vi "Cascade front panel-blockissues.vi"() -> ()   [LabVIEW 2016]
uses:
  sdi_12/SDI-12/Sonde Vertical Graph.ctl
  controls/Vertical Chart.ctl
  sdi_12/Groundwater header.ctl
  controls/MCC DAQ Setup.ctl
  controls/Aux Sensor.ctl
  KPRO_2016 subvis/Control 2.ctl
  KPRO_2016 subvis/Graph Controls 2.ctl
  KPRO_2016 subvis/Ik control.ctl
  controls/MCC DAQ Readings.ctl
  controls/Kpro pressure measurement cluster.ctl
  controls/Kpro hydraulic measurement cluster.ctl
  activeXtest/activeXtest 2015 Folder/sonde cluster from excel.ctl
  sdi_12/Sonde Value Percent Tol.ctl
  activeXtest/activeXtest 2015 Folder/sample data row cluster.ctl
  activeXtest/activeXtest 2015 Folder/sonde cluster.ctl
  KPRO_2016 subvis/Sensor Physical Measurements.ctl
  KPRO_2016 subvis/SS Control 7.ctl
  <vilib>/Utility/NIReport.llb/NI_report.lvclass
  controls/Action Control 1.ctl
  <extravilib>/ChannelInstances/One Element Stream-t'Action Control 1.ctl'/Instantiate.vi
  <extravilib>/ChannelInstances/One Element Stream-t'Action Control 1.ctl'/Endpoint.vi
  KPRO_2016 subvis/Kpro Globals.vi
  <vilib>/Utility/file.llb/Write Delimited Spreadsheet (string).vi
  <userlib>/_OpenG.lib/file/file.llb/Strip Path - Traditional__ogtk.vi
  <userlib>/_OpenG.lib/file/file.llb/Build Path - Traditional__ogtk.vi
  <vilib>/Utility/file.llb/Write Delimited Spreadsheet (DBL).vi
  <vilib>/ULx/Create Channel.llb/ULx Create Channel (AI-Voltage-Basic).vi
  <userlib>/_OpenG.lib/file/file.llb/Strip Path Extension - Path__ogtk.vi
  KPRO_2016 subvis/Global_SIM_switch.vi
  C:/Program Files (x86)/National Instruments/LabVIEW 2016/vi.lib/ULx/ULx_LV.dll
  Program Files (x86)/National Instruments/LabVIEW 2016/vi.lib/ULx/ULx_LV.dll
  <vilib>/Utility/config.llb/NI_LVConfig.lvlib
  <extravilib>/ChannelInstances/One Element Stream-t'Action Control 1.ctl'.lvlib
panel:
  out "Sonde OK":bool
  out "DAQ On":bool
  out "Number of Sample Sheets":i32
  out "Columns":i32[](array[numeric])
  in  "Create Excel File":bool
  out "output cluster":T1 caption="Cluster" {"Salinity" format="%_3g"; "Temp\ndeg C" format="%_2g"; "ORP" format="%_4g"; "pH" format="%_4g"; "Dissolved\nOxygen mg/L" format="%_3g"; "Specific\nCond (mS)" format="%_4g"; "Cumulative\nVolume (ml)" format="%#_4g"}
  out "Serial Number/MISC":string
  in  "Depth mode":bool caption="Use \nIncrement"
  in  "Sample Sheet Data Row Cluster 2":T2={"Head\nPressure"=0.0, "Depth"=0.0, "comment string"="", "Sonde Data Cluster"={"Cumulative\nVolume (ml)"=100.0, "Specific\nCond (mS)"=2.0, "Dissolved\nOxygen mg/L"=3.0, "pH"=4.0, "ORP"=5.0, "Temp\ndeg C"=26.0, "Salinity"=7.0}, "Aux1"=0.0, "Aux2"=0.0, "Aux3"=0.0} {"Sonde Data Cluster"."Salinity" format="%_3g"; "Sonde Data Cluster"."Temp\ndeg C" format="%_2g"; "Sonde Data Cluster"."ORP" format="%_4g"; "Sonde Data Cluster"."pH" format="%_4g"; "Sonde Data Cluster"."Dissolved\nOxygen mg/L" format="%_4g"; "Sonde Data Cluster"."Specific\nCond (mS)" format="%_4g"; "Sonde Data Cluster"."Cumulative\nVolume (ml)" format="%#_4g"; "Depth" format="%#.3g"; "Head\nPressure" format="%#.4g"}
  out "subarray":string[][](array[string])
  out "Initialization":i32
  in  "Increment Depth":bool
  in  "Finish Tests":bool
  in  "Start KPRO":bool
  in  "Record Continuous Samples":bool
  out "Current Time (s)":dbl
  in  "stop":bool
  in  "Write Data to csv file":bool
  in  "Sample Not Collected":bool
  in  "Record Single Sample":bool
  in  "Tab Control":T3(tab)
  out "12V Voltage Monitor":dbl format="%_3f"
  out "Found Quanta Sonde Com Port":refnum<visa-resource-name>
  in  "Temporary csv Data Files Directory":path=path "C:/Cascade/Data/Output Files"
  in  "Data File Directory":path=path "C:/Cascade/Data/Excel Reports"
  out "Quanta Sonde found?":bool
  in  "template file path":path=path "C:/Cascade/templates/Groundwater Profiling Log_empty_labview_template.xlsx"
  in  "Config File Path":path=path "C:/Cascade/Data/config files/DAQ Setup Config.ini"
  in  "Read Configuration File?":bool
  out "H-4191 Adapter found":bool
  in  "Save Configuration File?":bool
  out "Sonde Communication Error Out":errorcluster
  in  "Search for Comm Ports?":bool=TRUE
  in  "USB Serial Port Manual Entry":refnum<visa-resource-name>="COM13"
  in  "Sonde Parameters \nTolerance Limits":T4={"SC %"=10.0, "DO %"=10.0, "pH % "=10.0, "ORP % "=10.0, "Temp % "=10.0, "Salinity %"=10.0} {"Salinity %" format="%_2f%%"; "Temp %" format="%_2f%%"; "ORP %" format="%_2f%%"; "pH %" format="%_2f%%"; "DO %" format="%_2f%%"; "SC %" format="%_2f%%"}
  in  "Sonde Parameters \nInitial Values":T5 {"Salinity Initial" format="%_2f"; "Temp Initial" format="%_2f"; "ORP  Initial" format="%_2f"; "pH Initial" format="%_2f"; "DO Initial" format="%_2f"; "SC Initial" format="%_2f"}
  in  "Header path":path=path "C:/Cascade/templates/Fields for Excel sheets.xlsx"
  out "Sensor  Real \nMeasurements":T6 {"9V Monitor" format="%#.3g"; "Aux 3" format="%#.3g"; "Aux 2" format="%#.3g"; "Aux 1" format="%#.3g"; "String Pot" format="%#.3g"; "Top String Pot" format="%#_4g"; "Downhole Pressure" format="%#_4g"; "Flow" format="%#_4g"; "Uphole Pressure" format="%#_4g"}
  in  "MCC USB-DAQ Setup":T7={"Device Name in InstaCal"="Dev0", "Omega Pressure Sensor"={"DAQ Channel"=2.0, "Output Voltage Range"=1, "Enabled"=TRUE, "Description"="Uphole Pressure"}, "McMillian 102 Flowmeter"={"DAQ Channel"=11.0, "Output Voltage Range"=0, "Enabled"=TRUE, "Description"="Flow"}, "DHT Pressure Sensor"={"DAQ Channel"=3.0, "Output Voltage Range"=1, "Enabled"=TRUE, "Description"="Downhole Pressure"}, "Top String Pot"={"DAQ Channel"=0.0, "Output Voltage Range"=0, "Enabled"=TRUE, "Description"="Top String Pot"}, "String Pot Signal"={"DAQ Channel"=1.0, "Output Voltage Range"=0, "Enabled"=TRUE, "Description"="String Pot"}, "Aux Sensor 1"={"DAQ Channel"=5.0, "Output Voltage Range"=1, "Enabled"=TRUE, "Description"="Aux 1"}, "Aux Sensor 2"={"DAQ Channel"=6.0, "Output Voltage Range"=1, "Enabled"=TRUE, "Description"="Aux 2"}, "Aux Sensor 3"={"DAQ Channel"=7.0, "Output Voltage Range"=1, "Enabled"=TRUE, "Description"="Aux 3"}, "Voltage Monitor"={"DAQ Channel"=8.0, "Output Voltage Range"=0, "Enabled"=TRUE, "Description"="9V Monitor"}} {"Voltage Monitor"."Output Voltage Range" items=["+/-10 V Range", "+/-5 V Range", "+/-2.5V Range", "+/-1.25 V Range", "+/-0.625 V Range", "+/-0.3125 V Range", "+/-0.1562V Range", "+/-0.078125 V Range"]; "Aux Sensor 3"."Output Voltage Range" items=["+/-10 V Range", "+/-5 V Range", "+/-2.5V Range", "+/-1.25 V Range", "+/-0.625 V Range", "+/-0.3125 V Range", "+/-0.1562V Range", "+/-0.078125 V Range"]; "Aux Sensor 2"."Output Voltage Range" items=["+/-10 V Range", "+/-5 V Range", "+/-2.5V Range", "+/-1.25 V Range", "+/-0.625 V Range", "+/-0.3125 V Range", "+/-0.1562V Range", "+/-0.078125 V Range"]; "Aux Sensor 1"."Output Voltage Range" items=["+/-10 V Range", "+/-5 V Range", "+/-2.5V Range", "+/-1.25 V Range", "+/-0.625 V Range", "+/-0.3125 V Range", "+/-0.1562V Range", "+/-0.078125 V Range"]; "String Pot Signal"."Output Voltage Range" items=["+/-10 V Range", "+/-5 V Range", "+/-2.5V Range", "+/-1.25 V Range", "+/-0.625 V Range", "+/-0.3125 V Range", "+/-0.1562V Range", "+/-0.078125 V Range"]; "Top String Pot"."Output Voltage Range" items=["+/-10 V Range", "+/-5 V Range", "+/-2.5V Range", "+/-1.25 V Range", "+/-0.625 V Range", "+/-0.3125 V Range", "+/-0.1562V Range", "+/-0.078125 V Range"]; "DHT Pressure Sensor"."Output Voltage Range" items=["+/-10 V Range", "+/-5 V Range", "+/-2.5V Range", "+/-1.25 V Range", "+/-0.625 V Range", "+/-0.3125 V Range", "+/-0.1562V Range", "+/-0.078125 V Range"]; "McMillian 102 Flowmeter"."Output Voltage Range" items=["+/-10 V Range", "+/-5 V Range", "+/-2.5V Range", "+/-1.25 V Range", "+/-0.625 V Range", "+/-0.3125 V Range", "+/-0.1562V Range", "+/-0.078125 V Range"]; "Omega Pressure Sensor"."Output Voltage Range" items=["+/-10 V Range", "+/-5 V Range", "+/-2.5V Range", "+/-1.25 V Range", "+/-0.625 V Range", "+/-0.3125 V Range", "+/-0.1562V Range", "+/-0.078125 V Range"]}
  out "Rate":dbl=1000.0 caption="Sample Rate (Hz)"
  out "Number \nof Channels":u16
  in  "Channel \nData Rate S/s":dbl=3720.0 format="%#_13g"
  out "Descriptions":string[](array[string])
  out "Raw Voltages":dbl[](array[numeric])
  out "9V Voltage Monitor":dbl format="%#_3g"
  in  "Record DAQ Raw Voltages":bool
  out "Sensor Voltage Cluster":T9 {"9V Monitor" format="%#.3g"; "Aux 3" format="%#_3g"; "Aux 2" format="%#.3g"; "Aux 1" format="%#.3g"; "String Pot" format="%#.3g"; "Top String Pot" format="%#_3g"; "Downhole Pressure" format="%#.3g"; "Flow" format="%#_3g"; "Uphole Pressure" format="%-#1.3g"}
  out "KPRO Cumulative Output File Path":path=path "C:/Cascade/Data/Output Files/Output_files"
  in  "Clear Groundwater Header Values":bool
  in  "Groundwater Header":T10
  in  "Excel report file path":path=path "C:/Cascade/Data/Excel Reports/Groundwater Profiling Log_ara1.xlsx"
  out "Data Setup Indicator":string
  in  "Start Initialization":bool
  in  "Input Variables and Slopes":T11={"Total Volume"=0.0, "String Pot Slope"=1.6619999408721924, "Flow Slope"=39.040000915527344, "Up Hole Pressure Slope"=48.27000045776367, "Depth to Water Table"=-0.0, "Atmospheric Pressure"=32.22022530555725, "Reservoir Pressure"=-0.004827000045779073, "Height of Sample Box"=0.0, "DH Pressure Trans Slope"=42.0, "DH Pressure Offset"=0.0, "Up Hole  Pressure Offset"=0.0, "Aux 1 Slope"=1.0, "Aux 2 Slope"=1.0, "Aux 3 Slope"=1.0} {"Aux 3 Slope" format="%.2f"; "Aux 2 Slope" format="%.2f"; "Aux 1 Slope" format="%.2f"; "Up Hole  Pressure Offset" format="%.2f"; "DH Pressure Offset" format="%.2f"; "DH Pressure Trans Slope" format="%.2f"; "Height of Sample Box" format="%.2f"; "Reservoir Pressure" format="%.2f"; "Atmospheric Pressure" format="%.2f"; "Depth to Water Table" format="%.2f"; "Up Hole Pressure Slope" format="%.2f"; "Flow Slope" format="%.2f"; "String Pot Slope" format="%.2f"; "Total Volume" format="%.2f"}
  out "Pressure Offset":dbl
  out "appended path":path
  out "Down hole Pressure Transducer CSV":path
  out "Static IK path":path=path "C:/Cascade/Data/Output Files/Static Ik.csv"
  in  "Slopes File Path":path=path "C:/Cascade/Data/Output Files/slopes.csv"
  out "Output File Directory":path=path "C:/KPRO_2010/Output_files/Static Ik.txt"
  out "KPRO Session Output File Path":path=path "C:/Cascade/Data/Output Files/Output_files"
  in  "Slopes History File Path":path=path "C:/Cascade/Data/Output Files/slopes.csv"
  out "Sonde Recording Error file":path
  out "IK Recording Error file":path
  out "Sonde Data File":path
  out "Select Worksheet Index":i32
  out "NI_report out":refnum<class "NI_report.lvclass">
  out "column max value":i32
  out "Current Sample Sheet":string="Sample 1"
  out "last occupied cell's name":string
  out "row max value":i32
  in  "Current Sheet":i32=1
  out "Worksheet Names":string[](array[string])
  in  "Update Sonde":bool
  out "Sonde Data Array":T12[](array[typedef]) {"Salinity"."%" format="%_2f%%"; "Salinity"."Value" format="%_4g"; "Temperature"."%" format="%_2f%%"; "Temperature"."Value" format="%_4g"; "ORP"."%" format="%_2f%%"; "ORP"."Value" format="%_4g"; "pH"."%" format="%_2f%%"; "pH"."Value" format="%_4g"; "Dissolved Oxygen"."%" format="%_2f%%"; "Dissolved Oxygen"."Value" format="%_4g"; "Sp. Conductance"."%" format="%_2f%%"; "Sp. Conductance"."Value" format="%_4g"; "Cumulative\nVolume" format="%#_4g"}
  out "Table Label":string="Data from Sample Sheet %d from Excel File"
  out "Sonde Data Display Graphs":T14
  out "Temperature":cluster{"Y":dbl[], "Y":dbl[]}[](graph)
  in  "Record  Sonde Reason":bool
  in  "Select Reasons to Record Data":u16(ring) items=["Per Client Request", "Timed Out", "Sample stopped flowing", "Equipment Issue"]
  out "Sonde Recording Failure Path":path
  out "Sonde IK Behavior Path":path
  out "Recording Reason Sonde array":string[][](array[string])
  out "IK Reason array":string[][](array[string])
  out "SC Reference Calibration Response":string
  out "DO Reference Calibration Response":string
  out "Salinity Reference Calibration Response":string
  out "ORP Reference Calibration Response":string
  out "pH Reference Calibration Response":string
  out "SC  Reference\nCalibrate Response":bool
  out "DO  Reference\nCalibrate Response":bool
  in  "Salinity \nReference":dbl
  out "Salinity  Reference\nCalibrate Response":bool
  out "ORP  Reference\nCalibrate Response":bool
  in  "SC \nReference":dbl
  in  "DO \nReference":dbl
  in  "ORP Reference":dbl
  in  "pH Reference":dbl
  in  "pH Zero":dbl
  in  "Record  SC Calibration":bool
  in  "Record DO Calibration":bool
  in  "Record Salinity Calibration":bool
  in  "Record ORP Calibration":bool
  in  "Record pH Calibration Reference":bool
  in  "Record pH Calibration Zero":bool
  out "pH Zero \nCalibrate Response":bool
  out "pH  Reference\nCalibrate Response":bool
  out "pH Zero Calibration Response":string
  out "KPRO Finish\nIndicator":bool
  in  "Input Depths \nand Parameters Cluster":T16={"Flow"=0.21081600494384767, "Zeroed \nPressure"=74.74207969932556, "Ik"=0.003788962123473114, "Current Depth"=-100.6, "Feet of Stainless"=40, "Start Depth"=0.0, "Abs Start Depth"=0.0} {"Abs Start Depth" format="%.2f"; "Start Depth" format="%.2f"; "Current Depth" format="%.2f"; "Ik" format="%.2f"; "Zeroed \nPressure" format="%.2f"; "Flow" format="%.2f"}
  out "Zero Pressure\nIndicator":bool
  in  "Zero\nPressure":bool caption="Zero Pressure"
  in  "enable_IKMGS_file":bool
  in  "enable_slug_file":bool
  in  "enable_kpro_file":bool=TRUE
  in  "Simulate AD6B":bool
  out "KPRO Test\nIndicator":bool
  in  "Record DTW File":bool
  in  "Zero In-Line Pressure\n(F = leave as is)":bool=TRUE
  out "Current Session":sgl[][](array[numeric]) format="%.2f"
  in  "KPRO test report header":string[](array[string])=["Time(msecs)", "Uncorrected Depth", "Corrected Depth", "Drive_Rate", "Flow", "Feet_of Stainless", "Up Hole Pressure", "IK", "Corrected Pressure", "Atm Pressure", "Depth to water", "Height of box", "Res_Pressure", "Secs_since_1_JAN_1904", "Depth jumps more than 1_foot", "Down hole Pressure"]
  in  "Depth Cluster":T17
  out "Cumulative_data_from_file":sgl[][](array[numeric]) format="%.2f"
  in  "KPRO test report header 2":string[](array[string])=["Time(msecs)", "Uncorrected Depth", "Corrected Depth", "Drive_Rate", "Flow", "Feet_of Stainless", "Up Hole Pressure", "IK", "Corrected Pressure", "Atm Pressure", "Depth to water", "Height of box", "Res_Pressure", "Secs_since_1_JAN_1904", "Depth jumps more than 1_foot", "Down hole Pressure"]
  out "Cumulative_data_ready":bool
  out "Depth Rate\nft/min":dbl format="%#.2g"
  out "Ik":dbl=0.003788962123473114 caption="Real Time - Depth vs. lk" format="%.2f"
  out "Uphole Pressure":dbl format="%.2f"
  in  "New Depth":dbl
  in  "Update Depth":bool
  in  "Select Entry for IK Log File":u16(ring) items=["IK Increase", "IK stayed the Same", "IK decreased"]
  out "Large Depth IK Graph Cluster":T18={[0.003788962123473114, 0.0037174584307500765, 0.0037174584307500765, 0.0037174584307500765, 0.0037174584307500765, 0.003788962123473114], [-100.1, -100.2, -100.3, -100.4, -100.5, -100.6]}
  in  "Culmulative Graph Cluster":T19={"Cumulative - Depth vs. Ik"={[], []}, "Real Time - Depth vs. lk "={[0.003788962123473114, 0.0037174584307500765, 0.0037174584307500765, 0.0037174584307500765, 0.0037174584307500765, 0.003788962123473114], [-100.1, -100.2, -100.3, -100.4, -100.5, -100.6]}, "Cumulative - Depth vs. Drive Rate"={[], []}, "Real Time - Depth vs. Drive Rate"={[0.02036245163917736, 0.125, 0.16666666666666674, 0.16666666666666663, 0.16666666666666663, 0.16666666666666663], [-100.1, -100.2, -100.3, -100.4, -100.5, -100.6]}}
  out "Down hole Pressure":dbl format="%.2f"
  in  "Record IK Reason":bool
  in  "Corrected Pressure Cluster":T20
  out "Flow":dbl format="%#.2g"
  out "Current Depth":sgl=-100.6 format="%.2f"
  out "Current \nDepth (m)":sgl=-30.661383 format="%.2f"
  in  "Read String Pot":bool
  out "Large Depth IK Graph":dbl(graph)
  out "DAQ Error":errorcluster
  out "Initialization Finished":bool=TRUE
  out "Stop":bool
  out "error out":errorcluster
  in  "error in (no error)":errorcluster
  out "producer loop":i32
  out "consumer loop":i32
  out "Active Channel Array":string[](array[string])
  out "delimited string":string
  out "Voltage Range":dbl[](array[numeric])
  out "Stop 2":bool
  # "ft. water"
  # "mL/min."
  # "ft. water"
  # "ft."
  # "ft."
  # "Instructions for Sonde Calibration:\n1.  Use the Record Single Point to Record the Data prior to start of calibration procedure to record the initial points to the excel worksheet.\n2.  pH Calibration is a 2 step process:  A pH standard between 6.8 and 7.2 is treated as the “zero”\nand all other values are treated as the “slope”. First calibrate “zero”, then  add a second to calibrate “slope”. \n3.  Specific Conductance:  Wait for the specific conductance readings to stabilize in the calibration solution, which may\nrequire one or two minutes."
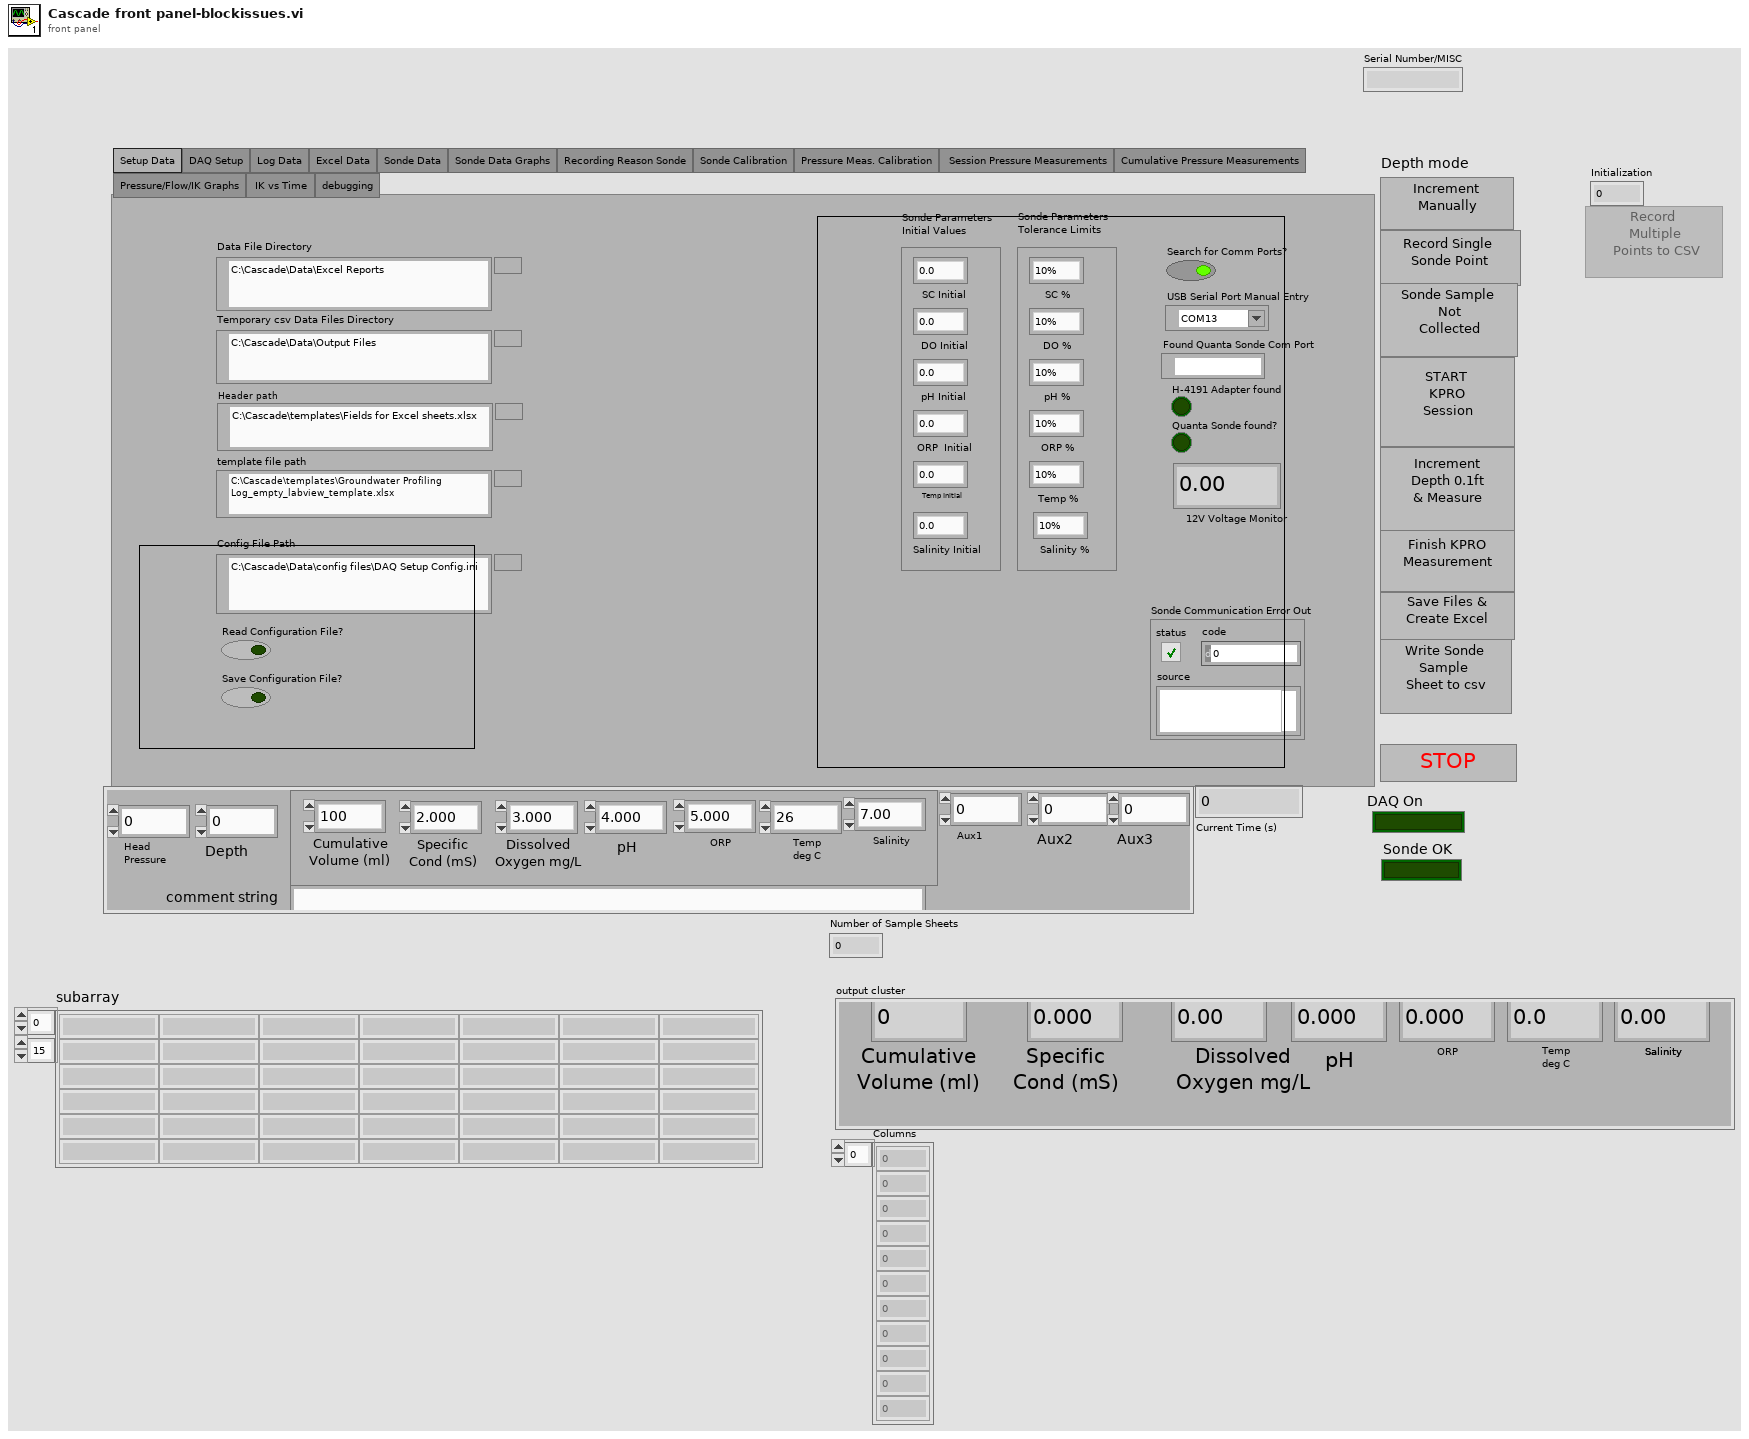
[diagram p1: front panel]
types:
  T1 = typedef "sonde cluster.ctl" = cluster{"Cumulative\nVolume (ml)":dbl, "Specific\nCond (mS)":dbl, "Dissolved\nOxygen mg/L":dbl, "pH":dbl, "ORP":dbl, "Temp\ndeg C":dbl, "Salinity":dbl}
  T2 = typedef "sample data row cluster.ctl" = cluster{"Head\nPressure":dbl, "Depth":dbl, "comment string":string, "Sonde Data Cluster":T1, "Aux1":dbl, "Aux2":dbl, "Aux3":dbl}
  T3 = enum32{"Setup Data", "DAQ Setup", "Log Data", "Excel Data", "Sonde Data", "Sonde Data Graphs", "Recording Reason Sonde", "Sonde Calibration", "Pressure Meas. Calibration", " Session Pressure Measurements", "Cumulative Pressure Measurements", "Pressure/Flow/IK Graphs", "IK vs Time ", "debugging"}
  T4 = cluster{"SC %":dbl, "DO %":dbl, "pH % ":dbl, "ORP % ":dbl, "Temp % ":dbl, "Salinity %":dbl}
  T5 = cluster{"SC Initial ":dbl, "DO Initial ":dbl, "pH Initial  ":dbl, "ORP  Initial":dbl, "Temp Initial":dbl, "Salinity Initial ":dbl}
  T6 = typedef "Sensor Physical Measurements.ctl" = cluster{"Uphole Pressure":dbl, "Flow":dbl, "Downhole Pressure":dbl, "Top String Pot":dbl, "String Pot":dbl, "Aux 1":dbl, "Aux 2":dbl, "Aux 3":dbl, "9V Monitor":dbl}
  T7 = typedef "MCC DAQ Setup.ctl" = cluster{"Device Name in InstaCal":string, "Omega Pressure Sensor":T8, "McMillian 102 Flowmeter":T8, "DHT Pressure Sensor":T8, "Top String Pot":T8, "String Pot Signal":T8, "Aux Sensor 1":T8, "Aux Sensor 2":T8, "Aux Sensor 3":T8, "Voltage Monitor":T8}
  T8 = typedef "Aux Sensor.ctl" = cluster{"DAQ Channel":dbl, "Output Voltage Range":u16, "Enabled":bool, "Description":string}
  T9 = typedef "MCC DAQ Readings.ctl" = cluster{"Uphole Pressure":dbl, "Flow":dbl, "Downhole Pressure":dbl, "Top String Pot":dbl, "String Pot":dbl, "Aux 1":dbl, "Aux 2":dbl, "Aux 3":dbl, "9V Monitor":dbl}
  T10 = typedef "Groundwater header.ctl" = cluster{"Location":string, "Date Finished":string, "CTS":string, "sampler":string, "Kpro box Serial ":string, "Sonde Serial":string, "Drilling Contractor":string, "Ave Depth to Water":string, "Gas/Peri Pump":string, "Atmospheric Pressure":string, "KPRO N2 Pressure":string, "Gas Drive N2 Pressure":string, "Profile ID":string}
  T11 = typedef "Control 2.ctl" = cluster{"Total Volume":dbl, "String Pot Slope":dbl, "Flow Slope":dbl, "Up Hole Pressure Slope":dbl, "Depth to Water Table":dbl, "Atmospheric Pressure":dbl, "Reservoir Pressure":dbl, "Height of Sample Box":dbl, "DH Pressure Trans Slope":dbl, "DH Pressure Offset":dbl, "Up Hole  Pressure Offset":dbl, "Aux 1 Slope":dbl, "Aux 2 Slope":dbl, "Aux 3 Slope":dbl}
  T12 = typedef "sonde cluster from excel.ctl" = cluster{"Head":dbl, "Depth":dbl, "Time":string, "Cumulative\nVolume":dbl, "Sp. Conductance":T13, "Dissolved Oxygen":T13, "pH":T13, "ORP":T13, "Temperature":T13, "Salinity":T13, "Final Tol.":bool, "Final":bool, "Time 2":timestamp, "Aux 1":dbl, "Aux 2":dbl, "Aux 3":dbl}
  T13 = typedef "Sonde Value Percent Tol.ctl" = cluster{"Value":dbl, "%":dbl, "Tol.":bool}
  T14 = typedef "Sonde Vertical Graph.ctl" = cluster{"pH":T15, "Conductance":T15, "Salinity":T15, "DO % Saturation":T15, "DO mg/L":T15, "ORP":T15}
  T15 = typedef "Vertical Chart.ctl" = cluster{"Y":dbl[], "Y":dbl[]}[]
  T16 = typedef "SS Control 7.ctl" = cluster{"Flow":dbl, "Zeroed \nPressure":dbl, "Ik":dbl, "Current Depth":sgl, "Feet of Stainless":i32, "Start Depth":sgl, "Abs Start Depth":sgl}
  T17 = typedef "Kpro hydraulic measurement cluster.ctl" = cluster{"Absolute Depth In":dbl, "Current Absolute Depth":dbl, "First Absolute Depth":dbl, "Previous Relative Depth":dbl, "Current Relative Depth":dbl, "First Relative Depth":dbl, "Last Filed Depth":dbl, "Total Volume In":dbl, "Total Volume Out":dbl, "Current Measurement Time":dbl, "Previous Measurement Time":dbl}
  T18 = typedef "Ik control.ctl" = cluster{dbl[], dbl[]}
  T19 = typedef "Graph Controls 2.ctl" = cluster{"Cumulative - Depth vs. Ik":cluster{dbl[], dbl[]}, "Real Time - Depth vs. lk ":cluster{dbl[], dbl[]}, "Cumulative - Depth vs. Drive Rate":cluster{dbl[], dbl[]}, "Real Time - Depth vs. Drive Rate":cluster{dbl[], dbl[]}}
  T20 = typedef "Kpro pressure measurement cluster.ctl" = cluster{"Up hole Corrected Pressure":dbl, "Down hole Corrected Pressure":dbl}
  T21 = typedef "Action Control 1.ctl" = enum16{"TimeOut", "Continuous  Sonde Data", "Init", "Exit", "Acq. Single Sonde Point", "Write Sonde Sample Sheet", "Acq. DAQ data", "Sample Not Collected", "Record Sonde Reason", "pH Calibration Zero", "pH Calibration Standard", "ORP Calibration Standard", "Salinity Calibration Standard", "DO Calibration Standard", "SC Calibration Standard", "Increment Depth Manually", "Start KPRO Measurements", "Finish KPRO Measurements", "Update Depth", "IK vs Time", "Record IK Reason", "Create Excel Files"}
  T22 = typedef "One Element Stream-t'Action Control 1.ctl'.lvlib/)Channel.ctl" = refnum<queue>
  T23 = typedef "NI_LVConfig.lvlib/Config Data RefNum.ctl" = refnum<k1>
  T24 = enum8{"Enabled", "Disabled", "Disabled and Grayed Out"}
  T25 = typedef "sonde cluster from excel.ctl" = cluster{"Head":dbl, "Depth":dbl, "Time":string, "Cumulative\nVolume":dbl, "Sp. Conductance":T13, "Dissolved Oxygen":T13, "pH":T13, "ORP":T13, "Temperature":T13, "Salinity":T13, "Final Tol.":bool, "Final":bool, "Time 2":string}
  T26 = enum16{"maximized", "minimized", "normal", "no change"}
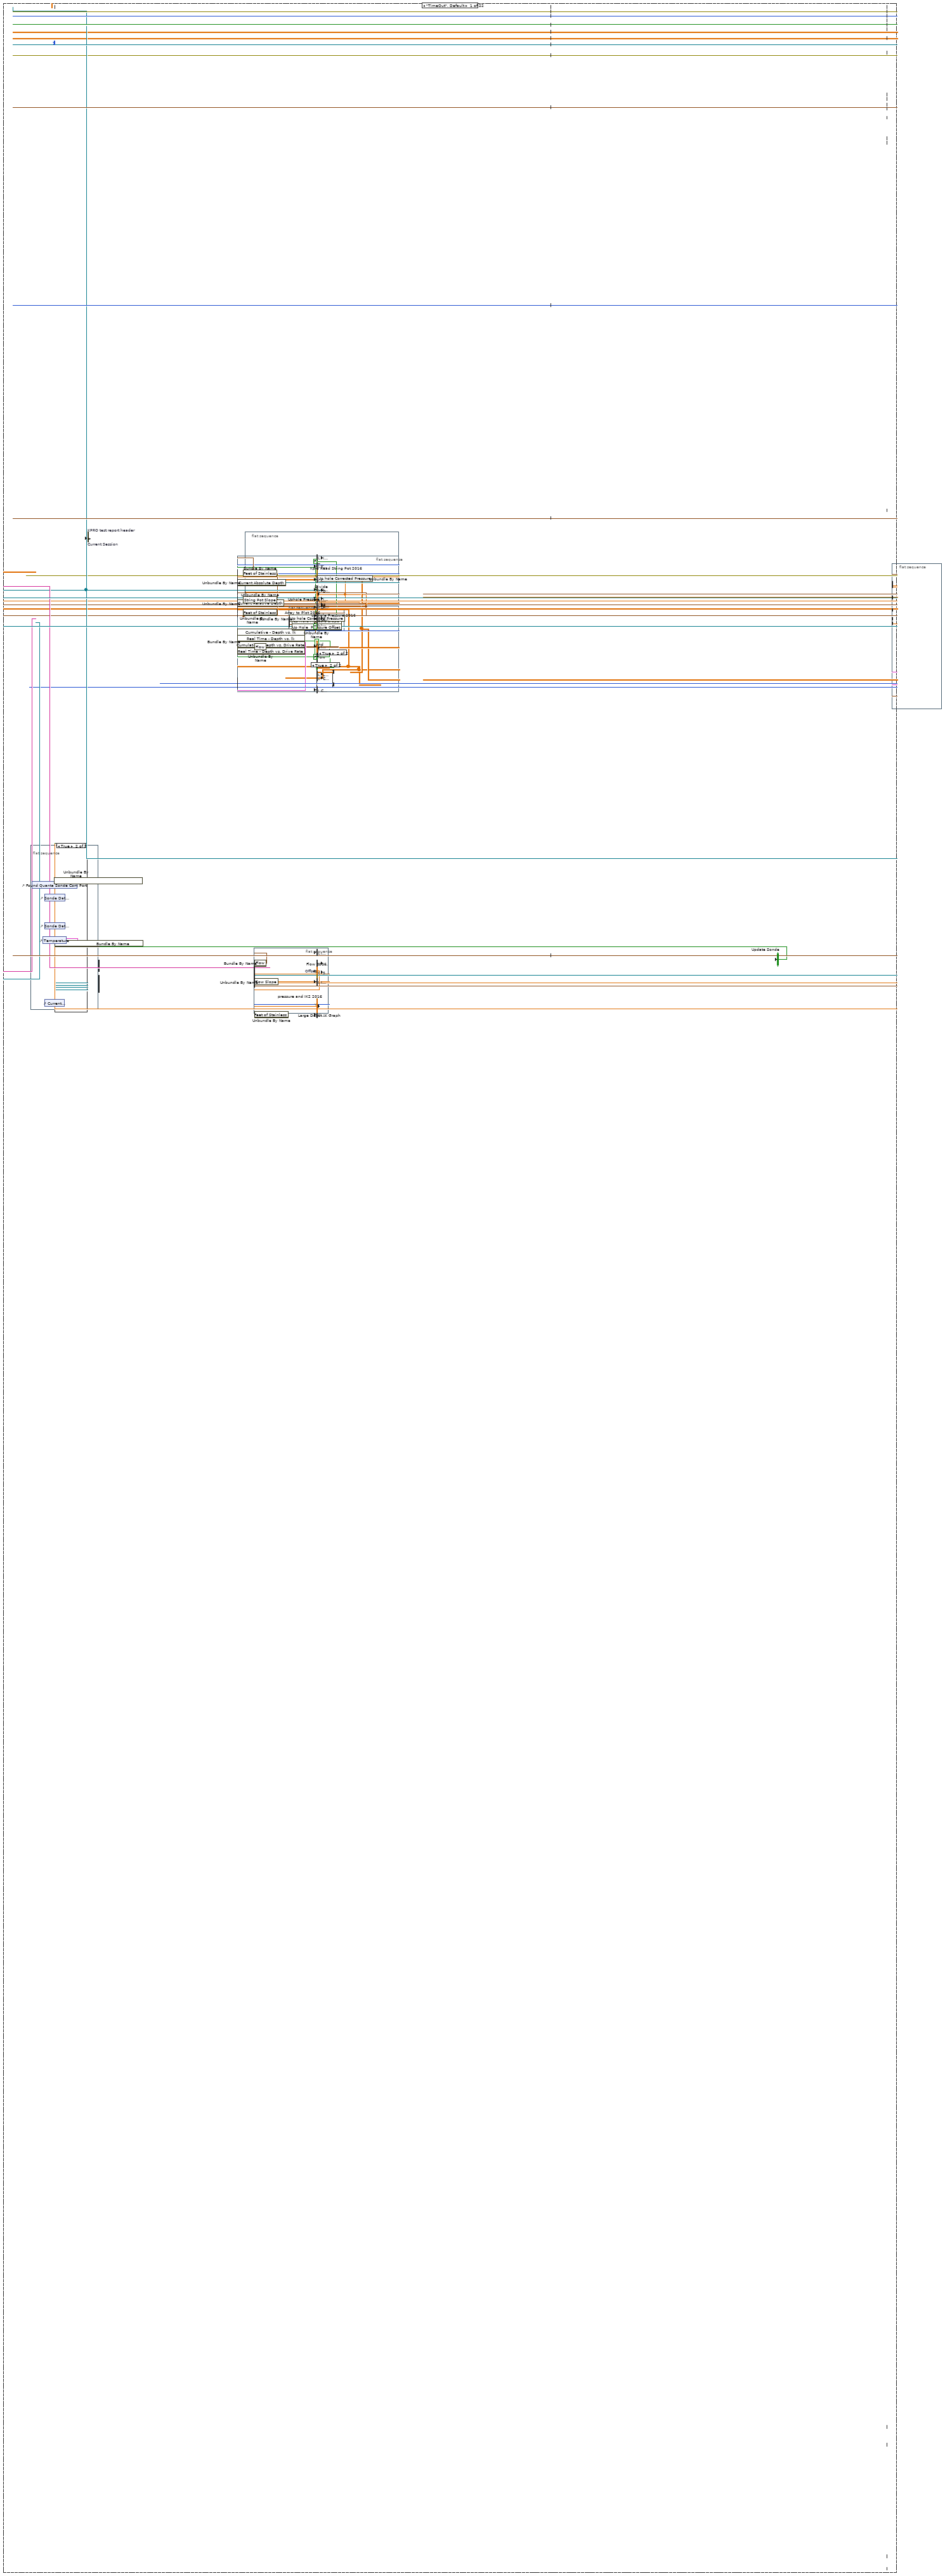
[diagram p4: hidden frame]
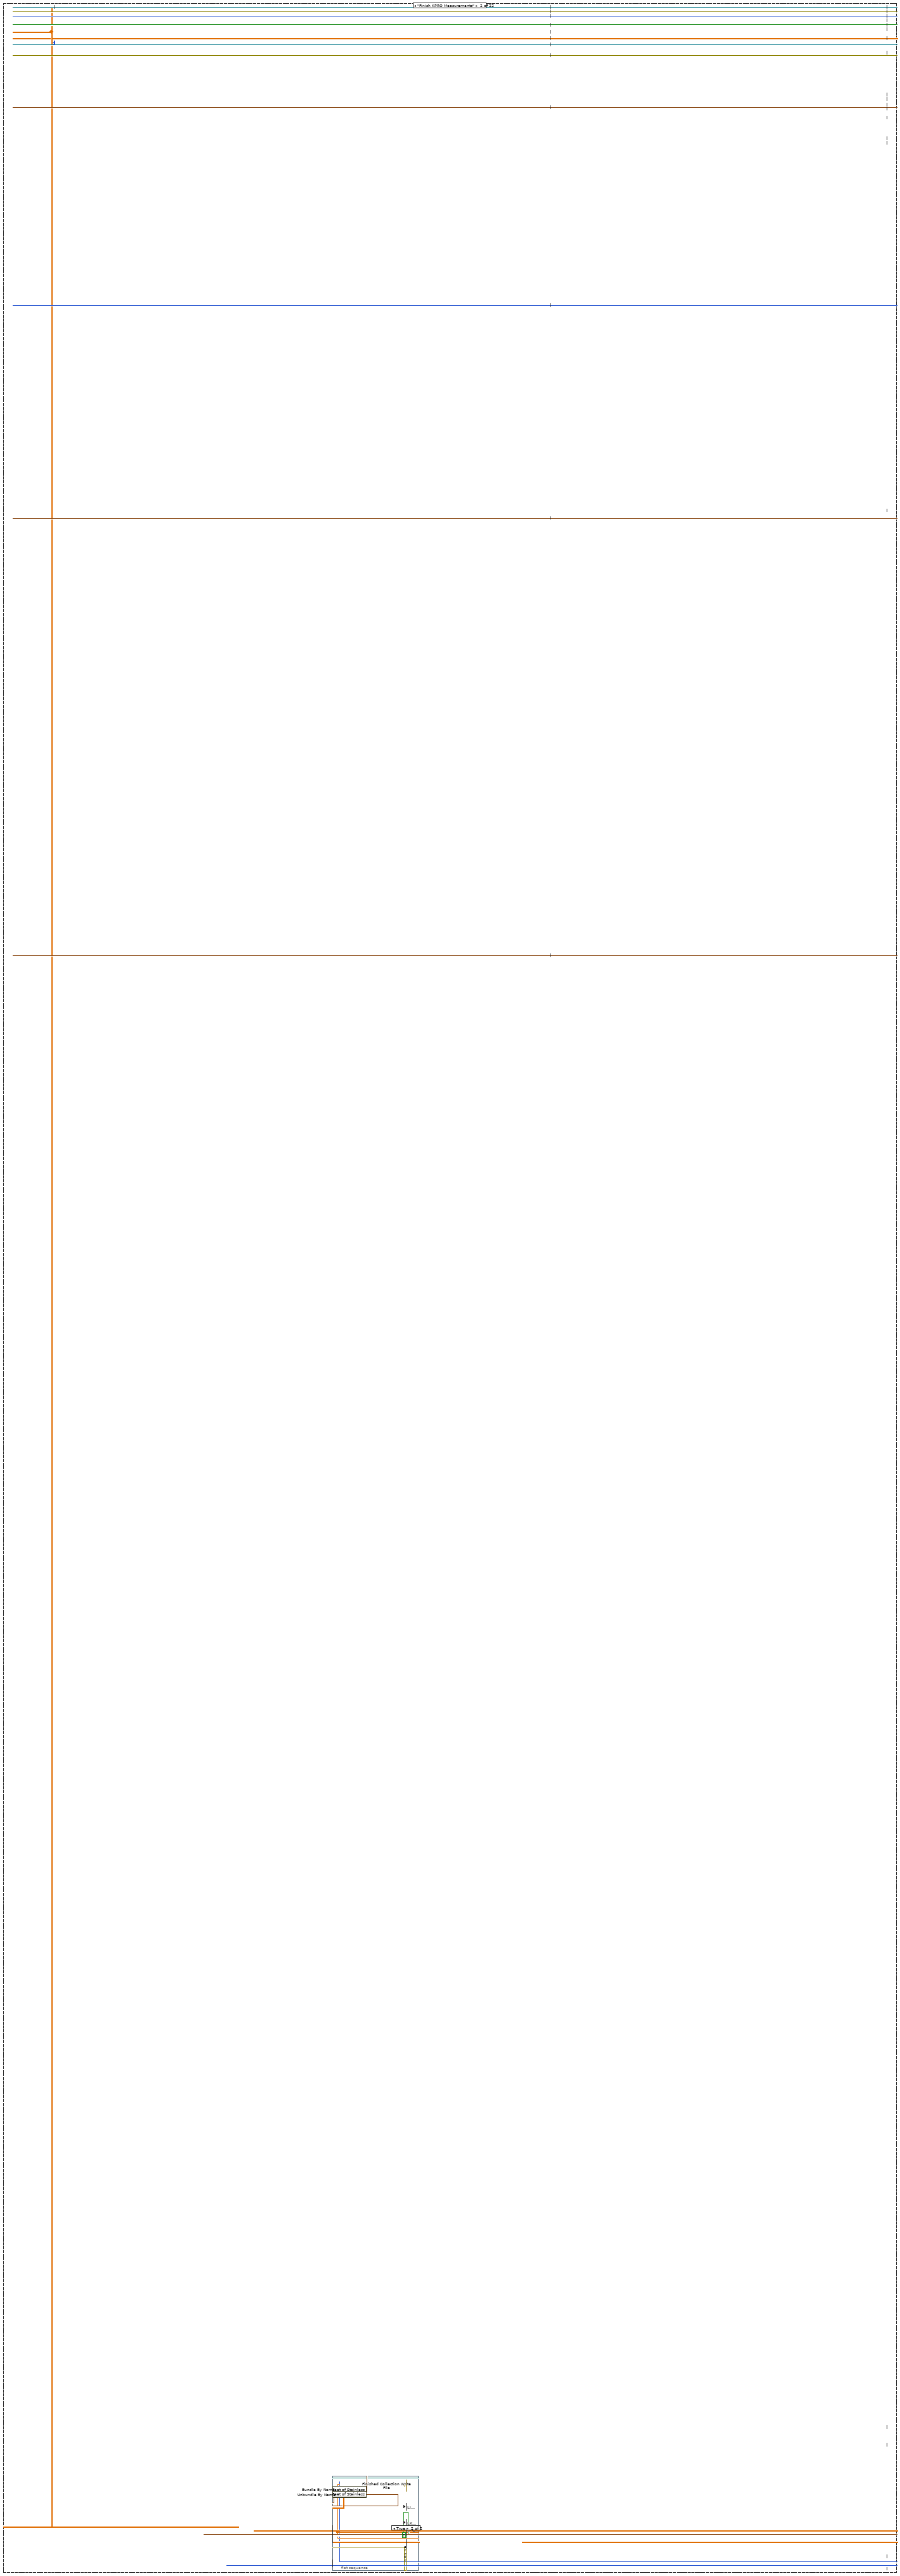
[diagram p8: hidden frame]
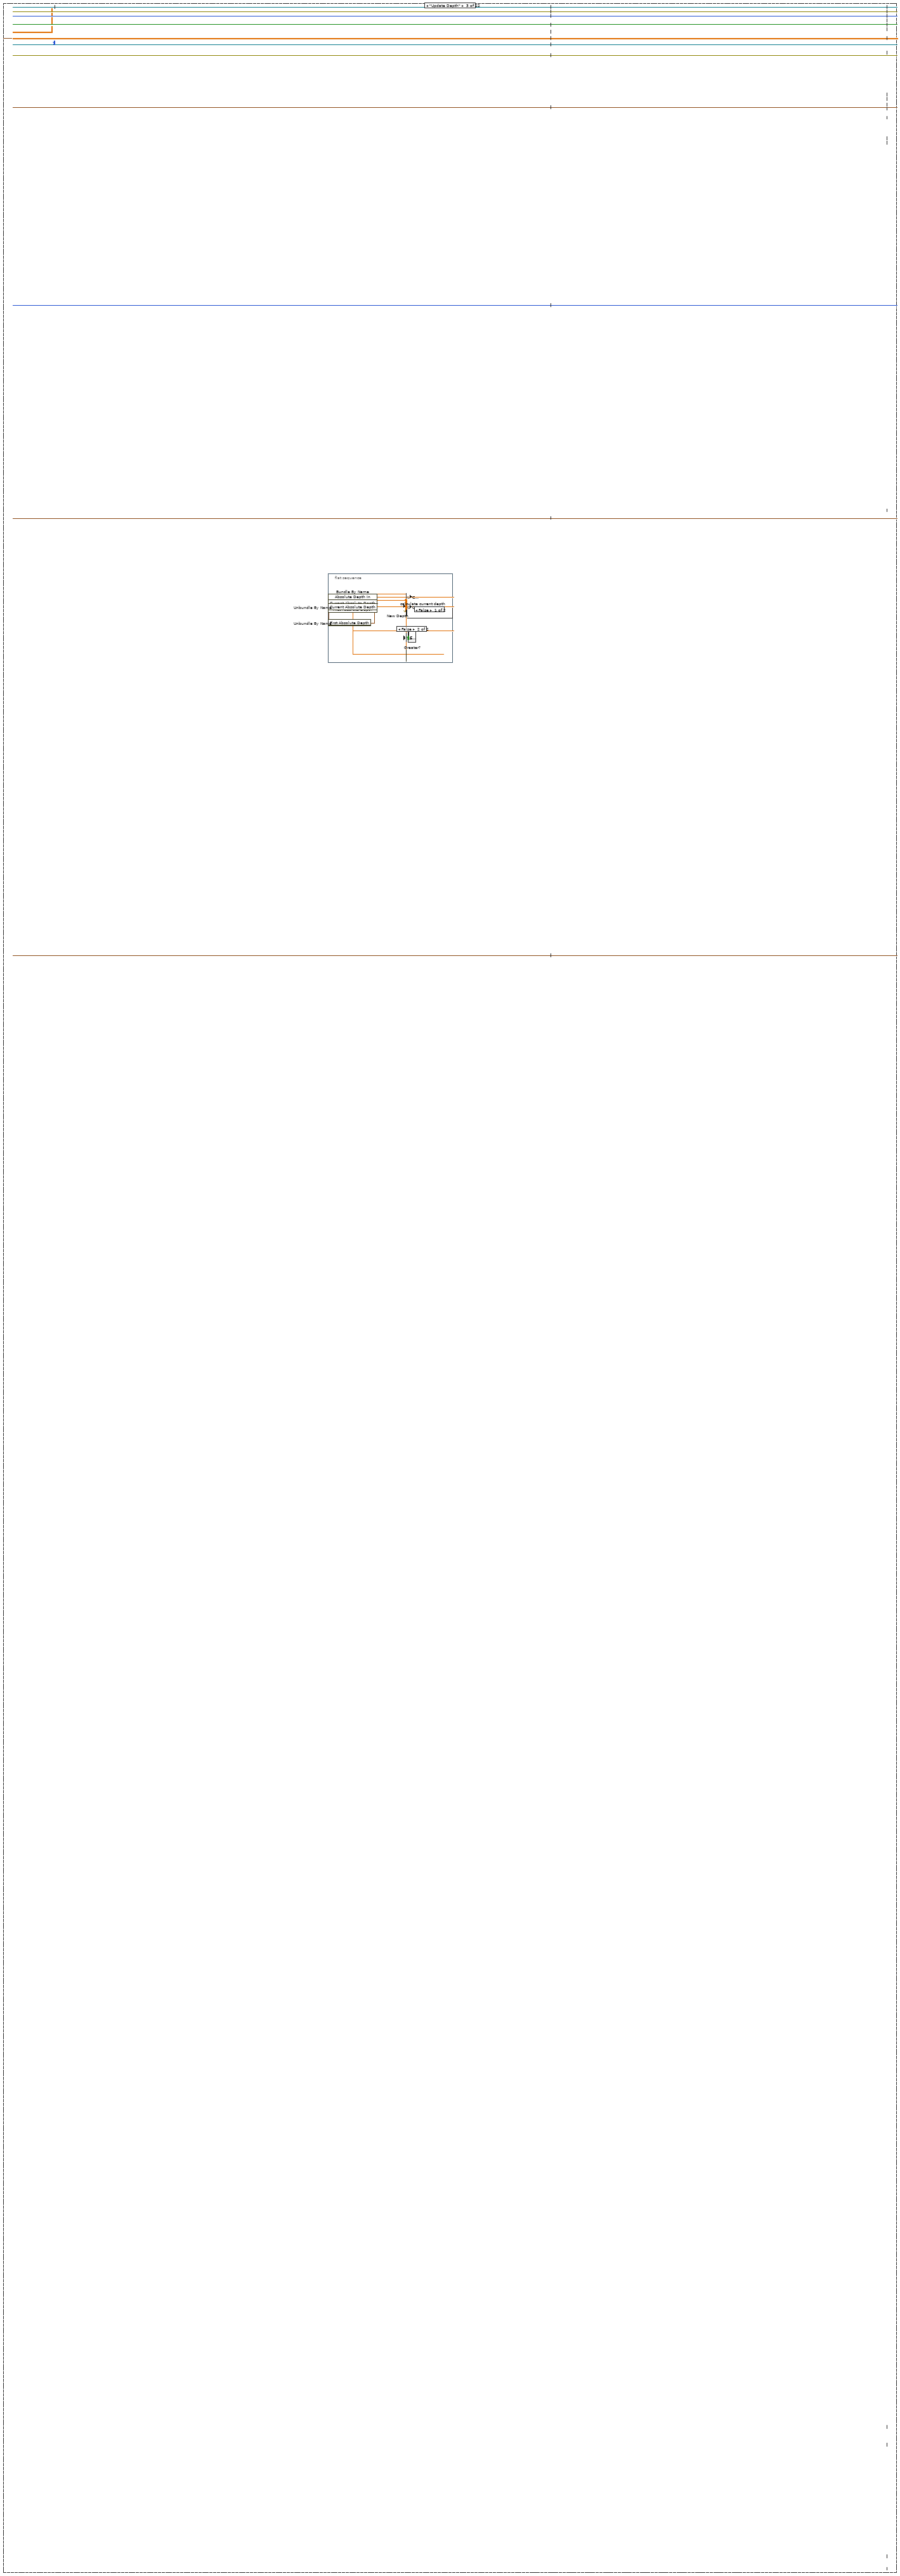
[diagram p10: hidden frame]
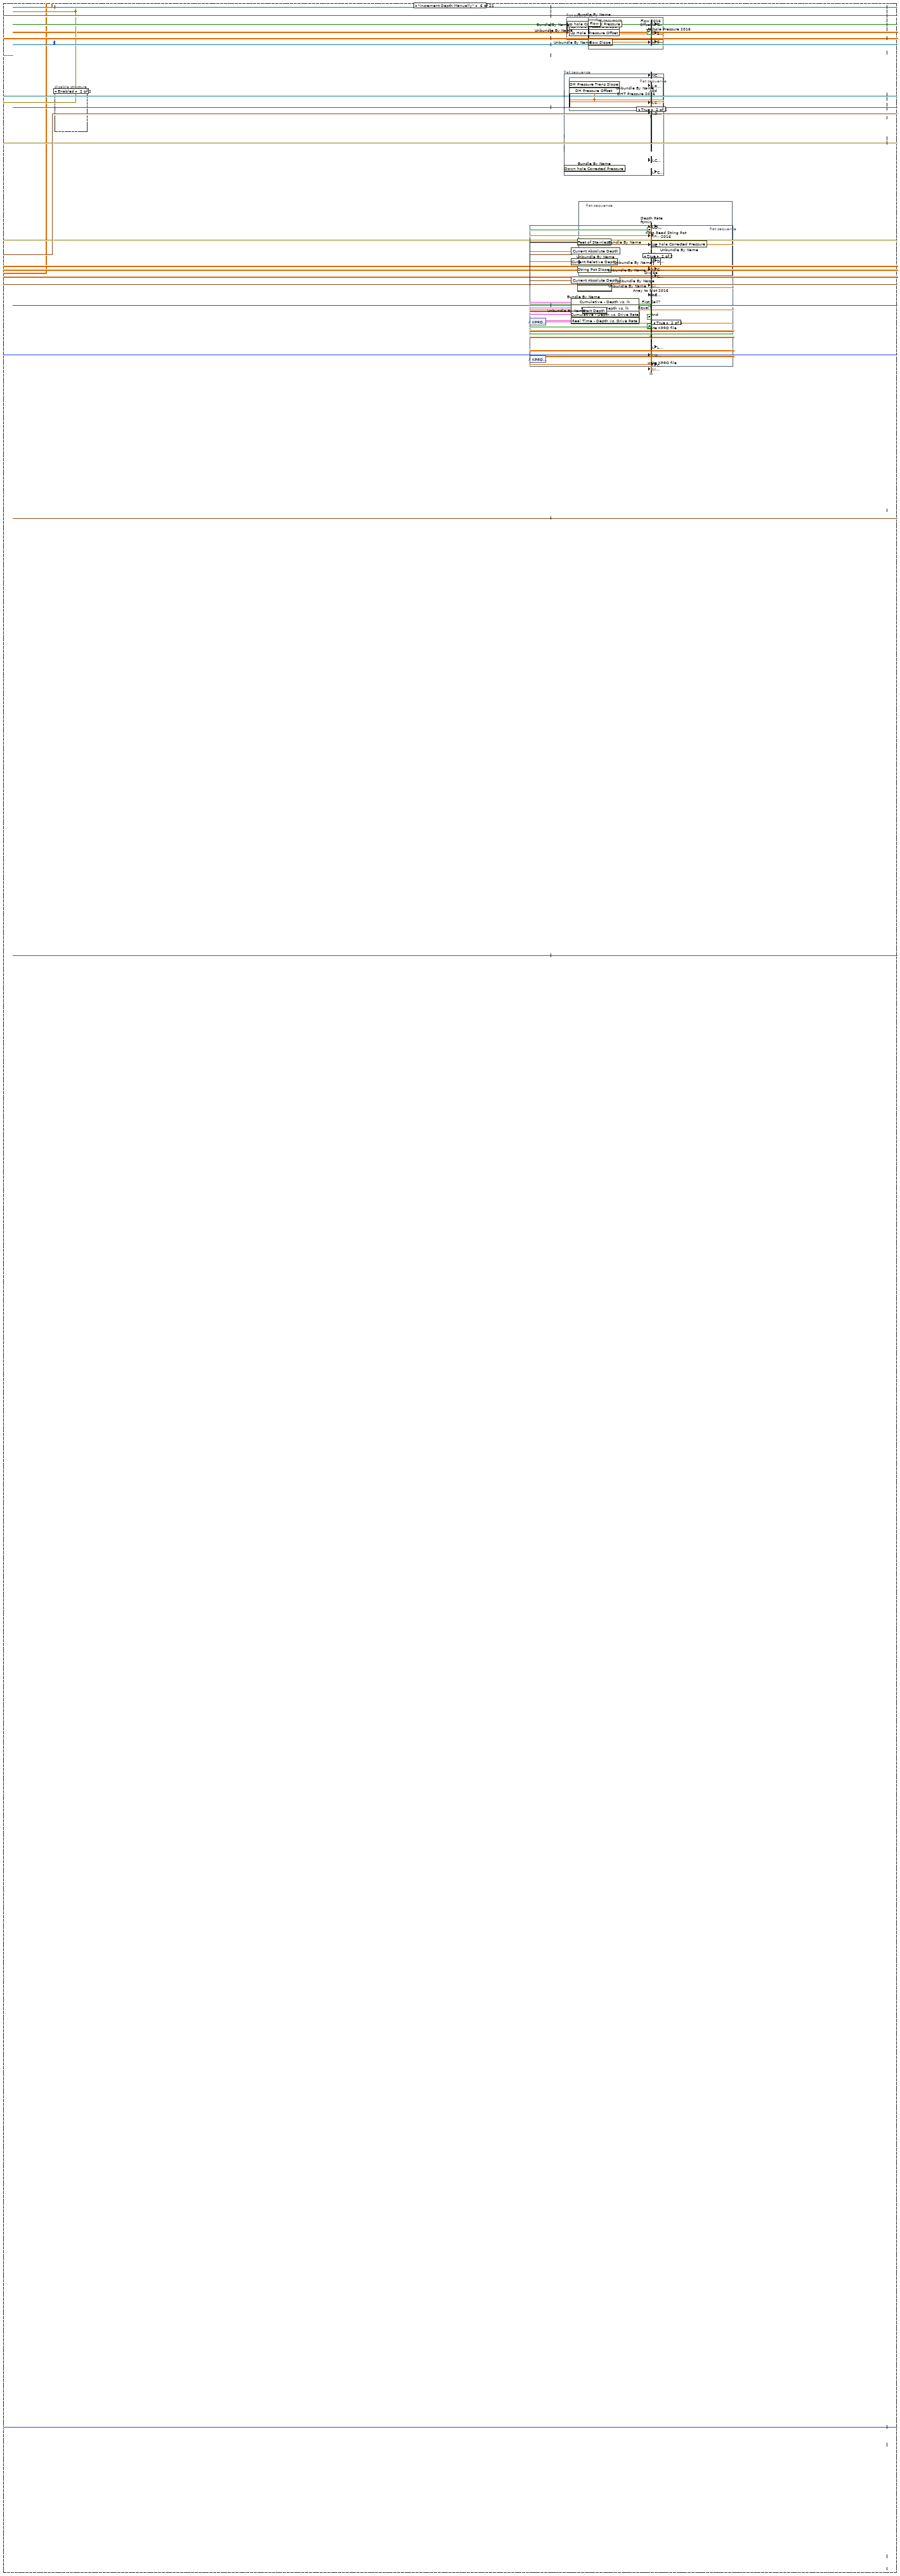
[diagram p17: hidden frame]
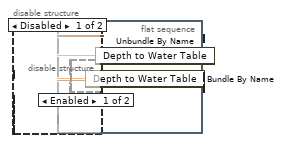
[diagram p18: hidden frame]
diagram:
  # "For calibrate command (XC) on SDI-12 address ‘a’, P is pH, C is specific conductance, S is\nsalinity or TDS, % is DO %Saturation, O is DO mg/L, R is ORP, D is depth, B is\nbarometric pressure, and t is TDS scale factor."
  n1 = flat-sequence {
    tunnel: [w16] -> w12
    tunnel: w8 -> [w15]
    tunnel: [w14] -> w4
    frame #0 {
      w13 = Action_Control_1."Init"  # Event
      n2 = while {
        shift-right: [w24] -> w16
        shift-left: w15 -> [w24]
        shift-right: [w19] -> _
        shift-left: w13 -> [w17]
        tunnel: [w25] -> w14
        i -> [w23]
        stop <- w21 stop-if-true
        # "User Interface Producer Loop"
        n3 = local read "Stop"() -> (w22:bool)
        n4 = First Call?() -> (First Call?: T/F=w18:bool)
        n5 = case shown="False" w18 {
          tunnel: w24 -> [w30 _]
          tunnel: [w28 FALSE ("Boolean")] -> w21
          tunnel: [w27 w225] -> w19
          tunnel: w17 -> [_ w225]
          frame False {
            w26 = Action_Control_1."TimeOut"  # Event
            n6 = event shown="[13] \"Write Data to csv file\": Value Change" {
              selector: _ -> [_ _ _ _ _ _ _ _ _ _ _ _ _ _ _ _ _ _ _ _ _]
              dyn-events: _ -> [_ _ _ _ _ _ _ _ _ _ _ _ _ _ _ _ _ _ _ _ _]
              timeout: 100 -> [_ _ _ _ _ _ _ _ _ _ _ _ _ _ _ _ _ _ _ _ _]
              tunnel: [w31 w34 w45 w51 w53 w66 w78 w90 w102 w114 w126 w138 w151 w162 w172 w180 w188 w196 w205 w213 _] -> w27
              tunnel: [FALSE w33 w44 TRUE w54 w67 w79 w91 w103 w115 w127 w139 w150 w161 w173 w181 w189 w197 w206 w214 _] -> w28
              tunnel: w30 -> [_ _ w42 _ w56 w69 w81 w93 w105 w117 w129 w141 _ w158 _ _ _ _ _ _ _]
              tunnel: [_ _ w42 _ w55 w68 w80 w92 w104 w116 w128 w140 _ _ _ _ _ _ _ _ _] -> _
              tunnel: w26 -> [w31 w35 w41 _ w52 w65 w77 w89 w101 w113 w125 w137 w149 w156 w170 w178 w187 w195 w204 w212 _]
              event Timeout {
                n7 = event-data() -> ()  [unwired: 1 in, 3 out]
              }
              event "Create Excel File": Value Change {
                n8 = event-data() -> ()  [unwired: 1 in, 6 out]
                n9 = case shown="True" "Create Excel File" {
                  tunnel: [FALSE FALSE] -> w33
                  tunnel: [w37 w39] -> w34
                  tunnel: w35 -> [_ w39]
                  frame True {
                    w37 = Action_Control_1."Create Excel Files"  # Event
                  }
                  frame False {
                  }
                }
              }
              event "stop": Value Change {
                n10 = case shown="True" "stop" {
                  tunnel: [w46 w48] -> w45
                  tunnel: [FALSE TRUE] -> w44
                  tunnel: w41 -> [w46 _]
                  frame False {
                  }
                  frame True {
                    w48 = Action_Control_1."Exit"  # Event
                  }
                }
                n11 = event-data() -> ()  [unwired: 1 in, 6 out]
              }
              event Panel Close? {
                w51 = Action_Control_1."Exit"  # Event
                n12 = event-data() -> ()  [unwired: 1 in, 4 out]
                n13 = event-data() -> ()  [unwired: 2 in, 1 out]
              }
              event "Record DAQ Raw Voltages": Value Change {
                n14 = case shown="False" "Record DAQ Raw Voltages" {
                  tunnel: [w58 w61] -> w53
                  tunnel: [FALSE FALSE ("Boolean")] -> w54
                  tunnel: [w59 w62] -> w55
                  tunnel: w56 -> [w59 w62]
                  tunnel: w52 -> [w58 _]
                  frame False {
                  }
                  frame True {
                    w61 = Action_Control_1."Acq. DAQ data"  # Event
                  }
                }
                n15 = event-data() -> ()  [unwired: 1 in, 6 out]
              }
              event "Record pH Calibration Zero": Value Change {
                n16 = case shown="True" "Record pH Calibration Zero" {
                  tunnel: [w70 w73] -> w66
                  tunnel: [FALSE FALSE ("Boolean")] -> w67
                  tunnel: [w71 w74] -> w68
                  tunnel: w69 -> [w71 w74]
                  tunnel: w65 -> [w70 _]
                  frame False {
                  }
                  frame True {
                    w73 = Action_Control_1."pH Calibration Zero"  # Event
                  }
                }
                n17 = event-data() -> ()  [unwired: 1 in, 6 out]
              }
              event "Record pH Calibration Reference": Value Change {
                n18 = case shown="True" "Record pH Calibration Reference" {
                  tunnel: [w82 w85] -> w78
                  tunnel: [FALSE FALSE ("Boolean")] -> w79
                  tunnel: [w83 w86] -> w80
                  tunnel: w81 -> [w83 w86]
                  tunnel: w77 -> [w82 _]
                  frame False {
                  }
                  frame True {
                    w85 = Action_Control_1."pH Calibration Standard"  # Event
                  }
                }
                n19 = event-data() -> ()  [unwired: 1 in, 6 out]
              }
              event "Record ORP Calibration": Value Change {
                n20 = case shown="True" "Record ORP Calibration" {
                  tunnel: [w94 w97] -> w90
                  tunnel: [FALSE FALSE ("Boolean")] -> w91
                  tunnel: [w95 w98] -> w92
                  tunnel: w93 -> [w95 w98]
                  tunnel: w89 -> [w94 _]
                  frame False {
                  }
                  frame True {
                    w97 = Action_Control_1."ORP Calibration Standard"  # Event
                  }
                }
                n21 = event-data() -> ()  [unwired: 1 in, 6 out]
              }
              event "Record Salinity Calibration": Value Change {
                n22 = case shown="True" "Record Salinity Calibration" {
                  tunnel: [w106 w109] -> w102
                  tunnel: [FALSE FALSE ("Boolean")] -> w103
                  tunnel: [w107 w110] -> w104
                  tunnel: w105 -> [w107 w110]
                  tunnel: w101 -> [w106 _]
                  frame False {
                  }
                  frame True {
                    w109 = Action_Control_1."Salinity Calibration Standard"  # Event
                  }
                }
                n23 = event-data() -> ()  [unwired: 1 in, 6 out]
              }
              event "Record DO Calibration": Value Change {
                n24 = case shown="True" "Record DO Calibration" {
                  tunnel: [w118 w121] -> w114
                  tunnel: [FALSE FALSE ("Boolean")] -> w115
                  tunnel: [w119 w122] -> w116
                  tunnel: w117 -> [w119 w122]
                  tunnel: w113 -> [w118 _]
                  frame False {
                  }
                  frame True {
                    w121 = Action_Control_1."DO Calibration Standard"  # Event
                  }
                }
                n25 = event-data() -> ()  [unwired: 1 in, 6 out]
              }
              event "Record  SC Calibration": Value Change {
                n26 = case shown="True" "Record  SC Calibration" {
                  tunnel: [w130 w133] -> w126
                  tunnel: [FALSE FALSE ("Boolean")] -> w127
                  tunnel: [w131 w134] -> w128
                  tunnel: w129 -> [w131 w134]
                  tunnel: w125 -> [w130 _]
                  frame False {
                  }
                  frame True {
                    w133 = Action_Control_1."SC Calibration Standard"  # Event
                  }
                }
                n27 = event-data() -> ()  [unwired: 1 in, 6 out]
              }
              event "Increment Depth": Value Change {
                n28 = case shown="True" "Increment Depth" {
                  tunnel: [w142 w145] -> w138
                  tunnel: [FALSE FALSE ("Boolean")] -> w139
                  tunnel: [w143 w146] -> w140
                  tunnel: w141 -> [w143 w146]
                  tunnel: w137 -> [w142 _]
                  frame False {
                  }
                  frame True {
                    w145 = Action_Control_1."Increment Depth Manually"  # Event
                  }
                }
                n29 = event-data() -> ()  [unwired: 1 in, 6 out]
              }
              event "Record Single Sample": Value Change {
                n30 = event-data() -> ()  [unwired: 1 in, 6 out]
                n31 = case shown="True" "Record Single Sample" {
                  tunnel: [w152 w154] -> w151
                  tunnel: [FALSE FALSE] -> w150
                  tunnel: w149 -> [w152 _]
                  frame False {
                  }
                  frame True {
                    w154 = Action_Control_1."Acq. Single Sonde Point"  # Event
                  }
                }
              }
              event "Write Data to csv file": Value Change {
                n32 = event-data() -> ("OldVal"=w160:bool, "NewVal"=w163:bool)  [unwired: 1 in, 4 out]
                n33 = Not(x=w160) -> (.not. x?=w159:bool)
                n34 = And(x=w159, y=w163) -> (x .and. y?=w157:bool)
                n35 = case shown="True" w157 {
                  tunnel: [w164 w167] -> w162
                  tunnel: [FALSE FALSE ("Boolean")] -> w161
                  tunnel: [w165 w168] -> _
                  tunnel: w158 -> [w165 w168]
                  tunnel: w156 -> [w164 _]
                  frame False {
                  }
                  frame True {
                    w167 = Action_Control_1."Write Sonde Sample Sheet"  # Event
                  }
                }
              }
              event "Sample Not Collected": Value Change {
                n36 = event-data() -> ("NewVal"=w171:bool)  [unwired: 1 in, 5 out]
                n37 = case shown="True" w171 {
                  tunnel: [FALSE FALSE] -> w173
                  tunnel: [w174 w176] -> w172
                  tunnel: w170 -> [_ w176]
                  frame True {
                    w174 = Action_Control_1."Sample Not Collected"  # Event
                  }
                  frame False {
                  }
                }
              }
              event "Record  Sonde Reason": Value Change {
                n38 = event-data() -> ("NewVal"=w179:bool)  [unwired: 1 in, 5 out]
                n39 = case shown="True" w179 {
                  tunnel: [FALSE FALSE] -> w181
                  tunnel: [w182 w184] -> w180
                  tunnel: w178 -> [_ w184]
                  frame True {
                    w182 = Action_Control_1."Record Sonde Reason"  # Event
                  }
                  frame False {
                  }
                }
              }
              event "Start KPRO": Value Change {
                n40 = event-data() -> ()  [unwired: 1 in, 6 out]
                n41 = case shown="True" "Start KPRO" {
                  tunnel: [FALSE FALSE] -> w189
                  tunnel: [w191 w193] -> w188
                  tunnel: w187 -> [_ w193]
                  frame True {
                    w191 = Action_Control_1."Start KPRO Measurements"  # Event
                    n42 = local write "KPRO Finish\nIndicator"(FALSE ("KPRO Finish\nIndicator")) -> ()
                  }
                  frame False {
                  }
                }
              }
              event "Update Depth": Value Change {
                n43 = case shown="True" "Update Depth" {
                  tunnel: [FALSE FALSE] -> w197
                  tunnel: [w199 w201] -> w196
                  tunnel: w195 -> [_ w201]
                  frame True {
                    w199 = Action_Control_1."Update Depth"  # Event
                  }
                  frame False {
                  }
                }
                n44 = event-data() -> ()  [unwired: 1 in, 6 out]
              }
              event "Record IK Reason": Value Change {
                n45 = case shown="True" "Record IK Reason" {
                  tunnel: [FALSE FALSE] -> w206
                  tunnel: [w207 w209] -> w205
                  tunnel: w204 -> [_ w209]
                  frame True {
                    w207 = Action_Control_1."Record IK Reason"  # Event
                  }
                  frame False {
                  }
                }
                n46 = event-data() -> ()  [unwired: 1 in, 6 out]
              }
              event "Finish Tests": Value Change {
                n47 = event-data() -> ()  [unwired: 1 in, 6 out]
                n48 = case shown="True" "Finish Tests" {
                  tunnel: [FALSE FALSE] -> w214
                  tunnel: [w216 w218] -> w213
                  tunnel: w212 -> [_ w218]
                  frame True {
                    w216 = Action_Control_1."Finish KPRO Measurements"  # Event
                    "KPRO Finish\nIndicator" <- TRUE ("KPRO Finish\nIndicator")
                  }
                  frame False {
                  }
                }
              }
              event "Depth mode": Value Change {
                n49 = case shown="True" "Depth mode" {
                  tunnel: [FALSE ("Read String Pot") TRUE ("Read String Pot")] -> w220
                  frame False {
                  }
                  frame True {
                  }
                }
                n50 = event-data() -> ()  [unwired: 1 in, 6 out]
                n51 = local write "Read String Pot"(w220) -> ()
              }
            }
          }
          frame True {
          }
        }
        "Stop" <- w21
        n52 = call <extravilib>:"Write With Abort.vi"("abort"=FALSE, "last element? (F)"=w21, "element"=w19) -> ("channel"=w25:T22)  [unwired: 6 in, 2 out]
        n53 = Or(x=w22, y=w21) -> ()  [unwired: 1 out]
        "producer loop" <- w23
      }
    }
  }
  n54 = flat-sequence {
    tunnel: [w228] -> w5
    tunnel: [w260] -> w7
    tunnel: w5 -> [w260]
    tunnel: [w256] -> w3
    tunnel: [w274] -> w9
    tunnel: w7 -> [w267]
    tunnel: [w267] -> w6
    tunnel: w9 -> [w305]
    tunnel: [w303] -> w8
    tunnel: [w306] -> w2
    tunnel: [w306] -> w1
    frame #0 {
      n55 = flat-sequence {
        tunnel: [w232] -> w228
        tunnel: w226 -> [w231]
        frame #0 {
          n56 = case shown="False" "Read Configuration File?" {
            selector: "Read Configuration File?" -> [_ w239]
            tunnel: [w233 w244] -> w232
            tunnel: w231 -> [w233 w241]
            tunnel: "Config File Path" -> [_ w240]
            frame False {
            }
            frame True {
              n57 = control-ref of="This VI"() -> (w242:refnum<vi>)
              n58 = call <vilib>:"Check if File or Folder Exists.vi"("error in (no error)"=w241, "path"=w240) -> ("error out"=w236:errorcluster, "file or folder exists?"=w237:bool, "dup path"=w235:path)  [unwired: 7 in]
              n59 = And(x=w239, y=w237) -> (x .and. y?=w238:bool)
              n60 = case shown="True" w238 {
                selector: w238 -> [w245 _]
                tunnel: w235 -> [_ w250]
                tunnel: w236 -> [w246 w254]
                tunnel: [w246 w247] -> w243
                tunnel: w242 -> [_ w255]
                frame False {
                  n61 = local write "Read Configuration File?"(w245) -> ()
                }
                frame True {
                  n62 = call <vilib>:"Open Config Data.vi"("error in (no error)"=w254, "create file if necessary (T)"=FALSE, "configuration file path"=w250) -> ("error out"=w252:errorcluster, "refnum"=w253:T23)  [unwired: 6 in, 1 out]
                  n63 = call <userlib>:"Read Panel from INI__ogtk.vi"("error in (no error)"=w252, "VI ref"=w255, "refnum"=w253) -> ("error out"=w248:errorcluster, "refnum out"=w249:T23)  [unwired: 7 in]
                  n64 = call <vilib>:"Close Config Data.vi"("error in (no error)"=w248, "refnum"=w249) -> ("error out"=w247:errorcluster)  [unwired: 8 in, 1 out]
                }
              }
              n65 = call <vilib>:"Clear Errors.vi"("error in (no error)"=w243) -> ("error out"=w234:errorcluster)  [unwired: 5 in, 1 out]
              n66 = Merge Errors(w234) -> (w244:errorcluster)
            }
          }
        }
      }
      n67 = invoke on="error out" class="Clust (strict)" method="Reinit To Default"(error in="error in (no error)") -> (error out=w226:errorcluster)  [unwired: 2 in, 2 out]
    }
    frame #1 {
      n68 = Get Date/Time In Seconds() -> (seconds since 1Jan1904=w256:timestamp)
      n69 = Get Date/Time In Seconds() -> (seconds since 1Jan1904=w257:timestamp)
      n70 = Subtract(x=w256, y=w257) -> (x-y=w258:dbl)
      n71 = To Double Precision Float(number=w258) -> (double precision float=→"Current Time (s)":dbl)
      n72 = local write "Current Sheet"(1 ("Current Sheet")) -> ()
    }
    frame #2 {
      w270 = T24."Enabled" ("Disabled")
      w290 = T24."Disabled and Grayed Out" ("Disabled")
      n73 = invoke on="DAQ On" class="Bool (strict)" method="Reinit To Default"() -> ()  [unwired: 3 in, 3 out]
      n74 = invoke on="Sonde OK" class="Bool (strict)" method="Reinit To Default"() -> ()  [unwired: 3 in, 3 out]
      n75 = local read "Groundwater Header"() -> (w271:T10)
      n76 = call "search for Quanta Sonde devices.vi"("VISA resource name"="USB Serial Port Manual Entry", "Search for Comm Ports?"="Search for Comm Ports?", "error in (no error)"=w267) -> ("12V monitor"=w266:dbl, "Com Port with Quanta Sonde devices"=w296:refnum<visa-resource-name>[], "Number of Quanta Sonde devices"=w295:i32, "Serial Number/MISC"=w272:string, "Number of Quanta Sonde devices > 0?"=w262:bool, "H-4191 Adapter found"=→"H-4191 Adapter found":bool, "Error Out"=w278:errorcluster)  [unwired: 4 in, 2 out]
      "Quanta Sonde found?" <- w262
      "12V Voltage Monitor" <- w266
      "Sonde Communication Error Out" <- w278
      "Serial Number/MISC" <- w272
      n77 = case shown="1" w295 {
        tunnel: w296 -> [_ w302]
        tunnel: [refnum<visa-resource-name> refnum ("RS232 Port Out") w300] -> w294
        frame 0, Default {
        }
        frame 1 {
          n78 = Index Array(array=w302, index=0) -> (element=w300:refnum<visa-resource-name>)
        }
      }
      "Found Quanta Sonde Com Port" <- w294
      n79 = Greater Or Equal?(x=w266, y=11.5) -> (x >= y?=w264:bool)
      n80 = And(x=w262, y=w264) -> (x .and. y?=→"Sonde OK":bool)
      n81 = Bundle By Name(cluster=w271, "Sonde Serial"=w272) -> (w273:T10)
      n82 = local write "Groundwater Header"(w273) -> ()
      n83 = call <vilib>:"Clear Errors.vi"("error in (no error)"=w278) -> ("error out"=w269:errorcluster)  [unwired: 5 in, 1 out]
      n84 = flat-sequence {
        tunnel: [w298] -> w268
        tunnel: w275 -> [w298]
        frame #0 {
          n85 = local write "Tab Control"(T3."Log Data" ("Tab Control")) -> ()
        }
      }
      n86 = local write "Initialization Finished"(FALSE ("Initialization Finished")) -> ()
      n87 = invoke on="Data Setup Indicator" class="Str" method="Reinit To Default"(error in=w268) -> (error out=w274:errorcluster)  [unwired: 2 in, 2 out]
      n88 = invoke on="Stop" class="Bool (strict)" method="Reinit To Default"(error in=w269) -> (error out=w280:errorcluster)  [unwired: 2 in, 2 out]
      n89 = invoke on="Stop 2" class="Bool (strict)" method="Reinit To Default"(error in=w280) -> (error out=w279:errorcluster)  [unwired: 2 in, 2 out]
      n90 = invoke on="Current Session" class="Arr (strict)" method="Reinit To Default"(error in=w268) -> ()  [unwired: 2 in, 3 out]
      n91 = property on="Clear Groundwater Header Values" class="Bool"(error in=w268, "DisabledEnum"=w270) -> ()  [unwired: 1 in, 2 out]
      n92 = property on="Start Initialization" class="Bool"(error in=w268, "DisabledEnum"=w270) -> ()  [unwired: 1 in, 2 out]
      n93 = flat-sequence {
        frame #0 {
          n94 = invoke on="Sonde Data Array" class="Arr (strict)" method="Reinit To Default"() -> ()  [unwired: 3 in, 3 out]
          n95 = control-ref of="Sonde Data Display"() -> ()  [unwired: 1 out]
        }
      }
      n96 = invoke on="Current Sheet" class="DigNum (strict)" method="Reinit To Default"(error in=w267) -> (error out=w283:errorcluster)  [unwired: 2 in, 2 out]
      n97 = invoke on="Sample Not Collected" class="Bool" method="Reinit To Default"(error in=w283) -> (error out=w287:errorcluster)  [unwired: 2 in, 2 out]
      n98 = invoke on="Record Continuous Samples" class="Bool" method="Reinit To Default"(error in=w287) -> (error out=w286:errorcluster)  [unwired: 2 in, 2 out]
      n99 = invoke on="Write Data to csv file" class="Bool" method="Reinit To Default"(error in=w286) -> (error out=w285:errorcluster)  [unwired: 2 in, 2 out]
      n100 = invoke on="Record Single Sample" class="Bool" method="Reinit To Default"(error in=w285) -> (error out=w284:errorcluster)  [unwired: 2 in, 2 out]
      n101 = invoke on="stop" class="Bool" method="Reinit To Default"(error in=w284) -> (error out=w289:errorcluster)  [unwired: 2 in, 2 out]
      n102 = property on="Write Data to csv file" class="Bool"(error in=w289, "DisabledEnum"=w290) -> (error out=w281:errorcluster)  [unwired: 1 in, 1 out]
      n103 = property on="Record Continuous Samples" class="Bool"("DisabledEnum"=w290) -> (error out=w291:errorcluster)  [unwired: 2 in, 1 out]
      n104 = property on="Record Single Sample" class="Bool"(error in=w291, "DisabledEnum"=w290) -> (error out=w292:errorcluster)  [unwired: 1 in, 1 out]
      n105 = property on="Sample Not Collected" class="Bool"(error in=w292, "DisabledEnum"=w290) -> (error out=w288:errorcluster)  [unwired: 1 in, 1 out]
      n106 = Merge Errors(w269, w279, w281, w288) -> (w275:errorcluster)
    }
    frame #3 {
      n107 = flat-sequence {
        tunnel: w304 -> [w331]
        tunnel: [w331] -> w303
        frame #0 {
          w332 = T24."Disabled and Grayed Out" ("Disabled")
          n108 = local write "KPRO Finish\nIndicator"(FALSE ("KPRO Finish\nIndicator")) -> ()
          n109 = property on="Clear Groundwater Header Values" class="Bool"("DisabledEnum"=w332) -> ()  [unwired: 2 in, 2 out]
          n110 = property on="Start Initialization" class="Bool"("DisabledEnum"=w332) -> ()  [unwired: 2 in, 2 out]
        }
      }
      n111 = while {
        tunnel: w305 -> [w313]
        tunnel: [w310] -> w304
        tunnel: [w312] -> _
        i -> [w312]
        stop <- w307 stop-if-true
        n112 = Quotient & Remainder(x=w312, y=100) -> (floor(x/y)=w308:i32)  [unwired: 1 out]
        n113 = call <userlib>:"Wait (ms)__ogtk.vi"("error in (no error)"=w313, "milliseconds to wait"=u32 100) -> ("error out"=w310:errorcluster)  [unwired: 8 in, 1 out]
        n114 = case shown="0" w308 {
          tunnel: w310 -> [w317 w319]
          frame 1, Default {
            n115 = property on="Data Setup Indicator" class="Str"(error in=w317, "Text.TextColor"=u32 0) -> ()  [unwired: 1 in, 2 out]
          }
          frame 0 {
            n116 = property on="Data Setup Indicator" class="Str"(error in=w319, "Text.TextColor"=u32 16716800) -> ()  [unwired: 1 in, 2 out]
          }
        }
        n117 = event shown="[2] \"stop\": Value Change" {
          selector: _ -> [_ _ _ _]
          dyn-events: _ -> [_ _ _ _]
          timeout: 100 -> [_ _ _ _]
          tunnel: [FALSE w322 TRUE _] -> w307
          event Timeout {
            n118 = event-data() -> ()  [unwired: 1 in, 3 out]
          }
          event "Start Initialization": Value Change {
            n119 = case shown="True" "Start Initialization" {
              tunnel: [FALSE ("Stop") TRUE ("Stop")] -> w322
              frame False {
              }
              frame True {
                n120 = invoke on="Data Setup Indicator" class="Str" method="Reinit To Default"() -> ()  [unwired: 3 in, 3 out]
                n121 = invoke on="Start Initialization" class="Bool" method="Reinit To Default"() -> ()  [unwired: 3 in, 3 out]
              }
            }
            n122 = event-data() -> ()  [unwired: 1 in, 3 out]
          }
          event "stop": Value Change {
            n123 = event-data() -> ()  [unwired: 1 in, 6 out]
          }
          event "Clear Groundwater Header Values": Value Change {
            n124 = case shown="True" "Clear Groundwater Header Values" {
              frame False {
              }
              frame True {
                n125 = invoke on="Groundwater Header" class="Clust (strict)" method="Reinit To Default"() -> (error out=w327:errorcluster)  [unwired: 3 in, 2 out]
                n126 = flat-sequence {
                  tunnel: w327 -> [_]
                  frame #0 {
                    n127 = local read "Groundwater Header"() -> (w328:T10)
                    n128 = local read "Serial Number/MISC"() -> (w329:string)
                    n129 = Bundle By Name(cluster=w328, "Sonde Serial"=w329) -> (w330:T10)
                    n130 = local write "Groundwater Header"(w330) -> ()
                  }
                }
              }
            }
            n131 = event-data() -> ()  [unwired: 1 in, 6 out]
          }
        }
        "Data Setup Indicator" <- "Hit the Start Key after Data Entry of Log Parameters and File Names." ("Data Setup Indicator")
      }
      n132 = flat-sequence {
        tunnel: [w335] -> w306
        tunnel: w303 -> [w334]
        frame #0 {
          n133 = flat-sequence {
            tunnel: w334 -> [w343]
            frame #0 {
              n134 = invoke on="Finish Tests" class="Bool" method="Reinit To Default"(error in=w343) -> (error out=w342:errorcluster)  [unwired: 2 in, 2 out]
              n135 = invoke on="Start KPRO" class="Bool" method="Reinit To Default"(error in=w342) -> (error out=w341:errorcluster)  [unwired: 2 in, 2 out]
              n136 = invoke on="Increment Depth" class="Bool" method="Reinit To Default"(error in=w341) -> (error out=w340:errorcluster)  [unwired: 2 in, 2 out]
              n137 = invoke on="Update Sonde" class="Bool (strict)" method="Reinit To Default"(error in=w340) -> (error out=w339:errorcluster)  [unwired: 2 in, 2 out]
              n138 = invoke on="Recording Reason Sonde array" class="Arr (strict)" method="Reinit To Default"(error in=w339) -> (error out=w338:errorcluster)  [unwired: 2 in, 2 out]
              n139 = invoke on="IK Reason array" class="Arr (strict)" method="Reinit To Default"(error in=w338) -> ()  [unwired: 2 in, 3 out]
            }
          }
          n140 = local read "Input Depths \nand Parameters Cluster"() -> (w337:T16)
          n141 = Unbundle By Name(w337) -> ("Feet of Stainless"=w335:i32)
          n142 = Bundle By Name(cluster=w337, "Feet of Stainless"=w335) -> (w336:T16)
          n143 = local write "Input Depths \nand Parameters Cluster"(w336) -> ()
        }
      }
    }
  }
  n144 = Merge Errors(w12, w11) -> (→"error out":errorcluster)
  n145 = flat-sequence {
    tunnel: [w369] -> w11
    tunnel: w8 -> [w368]
    tunnel: w6 -> [w364]
    tunnel: w4 -> [w363]
    tunnel: w3 -> [w361]
    tunnel: w2 -> [w360]
    tunnel: w1 -> [w359]
    frame #0 {
      w349 = dbl[][] []  # Cumulative Data over 1 string pot
      w353 = T5 {"SC Initial "=0.0, "DO Initial "=0.0, "pH Initial  "=0.0, "ORP  Initial"=0.0, "Temp Initial"=0.0, "Salinity Initial "=0.0}  # Sonde Parameters  Initial Values
      w354 = FALSE  # Read String Pot
      w355 = T16 {"Flow"=0.21081600494384767, "Zeroed \nPressure"=74.74207969932556, "Ik"=0.003788962123473114, "Current Depth"=-100.6, "Feet of Stainless"=40, "Start Depth"=0.0, "Abs Start Depth"=0.0}  # Input Depths  and Parameters Cluster
      w356 = T17 {"Absolute Depth In"=0.0, "Current Absolute Depth"=0.0, "First Absolute Depth"=0.0, "Previous Relative Depth"=0.0, "Current Relative Depth"=0.0, "First Relative Depth"=0.0, "Last Filed Depth"=0.0, "Total Volume In"=0.0, "Total Volume Out"=0.0, "Current Measurement Time"=0.0, "Previous Measurement Time"=0.0}  # Depth Cluster
      w357 = dbl[][] []  # Cumulative Data From File
      n146 = Get Date/Time In Seconds() -> (seconds since 1Jan1904=w352:timestamp)
      n147 = To Double Precision Float(number=w352) -> (double precision float=w351:dbl)
      n148 = flat-sequence {
        tunnel: [w375] -> _
        tunnel: [w374] -> w344
        tunnel: [w373] -> w345
        tunnel: [w372] -> w346
        tunnel: [w371] -> w347
        tunnel: [w370] -> w348
        frame #0 {
          n149 = local read "Worksheet Names"() -> (w370:string[])
          n150 = local read "Number of Sample Sheets"() -> (w371:i32)
          n151 = local read "row max value"() -> (w372:i32)
          n152 = local read "Columns"() -> (w373:i32[])
          n153 = local read "NI_report out"() -> (w374:refnum<class "NI_report.lvclass">)
          n154 = local read "Select Worksheet Index"() -> (w375:i32)
        }
      }
      n155 = while {
        tunnel: w368 -> [w426]
        tunnel: [w427] -> w369
        tunnel: w363 -> [w407]
        tunnel: w344 -> [w378]
        shift-right: [w417] -> _
        shift-left: "Current Sheet" -> [w380]
        tunnel: w348 -> [w419]
        tunnel: w346 -> [w424]
        shift-right: [w418] -> _
        shift-left: 0 ("row index") -> [w423]
        tunnel: [w422] -> _
        shift-right: [w421] -> _
        shift-left: cluster{"row":i32, "column":i32} {"row"=0, "column"=0} ("start of last occupied row") -> [w420]
        tunnel: w347 -> [w416]
        shift-right: [w413] -> _
        shift-left: dbl[] [] ("Time Array") -> [w414]
        shift-right: [w412] -> _
        shift-left: w357 -> [w411]
        tunnel: w351 -> [w410]
        tunnel: [w409] -> _
        tunnel: w364 -> [w397]
        shift-right: [w405] -> _
        shift-left: refnum<k24>[] [] -> [w396]
        tunnel: w361 -> [w385]
        shift-right: [w384] -> _
        shift-left: w360 -> [w386]
        shift-right: [w404] -> _
        shift-left: w359 -> [w404]
        shift-right: [w402] -> _
        shift-left: w354 -> [w401]
        shift-right: [w389] -> _
        shift-left: w356 -> [w400]
        shift-right: [w399] -> _
        shift-left: w355 -> [w398]
        shift-right: [w393] -> _
        shift-left: w353 -> [_]
        shift-right: [w391] -> _
        shift-left: dbl[][] [] ("Cumulative Sonde \nData Out") -> [w390]
        shift-right: [w388] -> _
        shift-left: w349 -> [w387]
        shift-right: [w377] -> _
        shift-left: w345 -> [w425]
        i -> [w394]
        stop <- w408 stop-if-true
        # "Consumer Data Handling Loop"
        n156 = feedback-in #1(w383) -> ()
        n157 = feedback #1() -> (w376:T21)  [unwired: 1 in]
        n158 = local read "Columns"() -> (w377:i32[])
        n159 = flat-sequence {
          tunnel: w394 -> [w432]
          frame #0 {
            "consumer loop" <- w432
          }
        }
        n160 = disable-structure shown="Enabled" {
          disable-tunnel: w397 -> [w439 _]
          disable-tunnel: w396 -> [w438 w447]
          disable-tunnel: [w437 w447] -> w395
          disable-tunnel: w394 -> [w436 _]
          frame Enabled {
            n161 = case shown="1, Default" w436 {
              tunnel: w438 -> [w440 w446]
              tunnel: w439 -> [_ w445]
              tunnel: [w440 w443] -> w437
              frame 0 {
              }
              frame 1, Default {
                n162 = local read "Descriptions"() -> (w444:string[])
                n163 = call "Measure DAQ Voltages.vi"("error in (no error)"=w445, "Descriptions"=w444, "Array in"=w446) -> ("Raw Voltages"=w442:dbl[], "Array out"=w443:refnum<k24>[], "Sensor Cluster"=w441:T9)  [unwired: 6 in]
                n164 = local write "Sensor Voltage Cluster"(w441) -> ()
                n165 = local write "Raw Voltages"(w442) -> ()
              }
            }
          }
          frame Disabled {
          }
        }
        n166 = flat-sequence {
          tunnel: w407 -> [w430]
          tunnel: [w429] -> w406
          tunnel: [w428] -> w383
          frame #0 {
            n167 = call <extravilib>:"Read With Abort.vi"("abort"=FALSE, "channel"=w430) -> ("last element?"=w429:bool, "element"=w428:T21)  [unwired: 5 in, 3 out]
          }
        }
        n168 = flat-sequence {
          tunnel: w385 -> [w433]
          frame #0 {
            n169 = Get Date/Time In Seconds() -> (seconds since 1Jan1904=w434:timestamp)
            n170 = Subtract(x=w434, y=w433) -> (x-y=w435:dbl)
            n171 = local write "Current Time (s)"(w435) -> ()
          }
        }
        n172 = call <userlib>:"Wait (ms)__ogtk.vi"("error in (no error)"=w426, "milliseconds to wait"=u32 50) -> ("error out"=w379:errorcluster)  [unwired: 8 in, 1 out]
        n173 = Format Into String(format string="Sample Sheet %d ", error in=w379, w380) -> (resulting string=→"Table Label":string, error out=w403:errorcluster)  [unwired: 1 in]
        n174 = case shown="\"Init\"" w383 {
          selector: w383 -> [_ _ _ _ _ _ _ _ _ _ _ _ _ _ _ _ _ w2010 _ _ _ _]
          tunnel: w403 -> [w462 w621 w662 w705 w728 w873 w1062 w1079 w1115 w1158 w1191 w1297 w1416 w1536 w1656 w1775 w1894 w2016 w2136 w2620 w2636 w2710]
          tunnel: [w462 w621 w662 w705 w724 w869 w1062 w1079 w1115 w1157 w1189 w1295 w1414 w1534 w1654 w1773 w1892 w2000 w2136 w2620 w2646 w2711] -> w427
          tunnel: w406 -> [_ _ _ _ _ _ _ _ _ _ _ _ _ _ _ _ _ _ _ _ _ _]
          tunnel: w378 -> [w478 w611 w661 w704 w745 w893 w1061 w1078 w1114 w1152 w1166 w1312 w1430 w1550 w1670 w1790 w1908 w2017 w2143 w2619 w2637 _]
          tunnel: [w477 w620 w660 w703 w744 w892 w1060 w1077 w1113 w1151 w1187 w1292 w1411 w1531 w1651 w1770 w1889 w2005 w2142 w2618 w2651 w2726] -> w418
          tunnel: w425 -> [_ _ _ _ _ _ _ _ _ _ w1193 w1310 w1428 w1548 w1668 w1788 w1906 _ _ _ _ _]
          tunnel: w424 -> [_ _ _ _ _ _ _ _ _ _ w1164 w1309 w1427 w1547 w1667 w1787 w1905 _ _ _ _ _]
          tunnel: w423 -> [w477 w620 w660 w703 w744 w892 w1060 w1077 w1113 w1151 w1162 w1293 w1412 w1532 w1652 w1771 w1890 w1994 w2142 w2618 w2651 w2726]
          tunnel: [w478 w611 w661 w704 w745 w893 w1061 w1078 w1114 w1152 w1192 w1298 w1417 w1537 w1657 w1776 w1895 w2015 w2143 w2619 w2652 w2727] -> w422
          tunnel: w380 -> [w476 w619 w659 w702 w732 w877 w1059 w1076 w1112 w1150 w1163 w1306 w1424 w1544 w1664 w1784 w1902 w2012 w2141 w2617 w2650 w2706]
          tunnel: [w476 w619 w659 w702 w732 w877 w1059 w1076 w1112 w1150 w1163 w1306 w1424 w1544 w1664 w1784 w1902 w2011 w2141 w2617 w2650 w2706] -> w417
          tunnel: [w475 w618 w658 w701 w743 w891 w1058 w1075 w1111 w1149 w1188 w1294 w1413 w1533 w1653 w1772 w1891 w2008 w2140 w2616 w2649 w2725] -> w421
          tunnel: w420 -> [w475 w618 w658 w701 w743 w891 w1058 w1075 w1111 w1149 w1165 w1276 w1395 w1514 w1634 w1754 w1872 w1991 w2140 w2616 w2649 w2725]
          tunnel: w419 -> [_ _ _ _ _ _ _ _ _ _ _ _ _ _ _ _ _ w2014 _ _ _ _]
          tunnel: w416 -> [_ _ _ _ _ _ _ _ _ _ _ _ _ _ _ _ _ w2013 _ _ _ _]
          tunnel: w376 -> [_ _ _ _ _ _ _ _ _ _ _ _ _ _ _ _ _ w2009 _ _ _ _]
          tunnel: w414 -> [w461 w617 w657 w700 w742 w890 w1057 w1074 w1110 w1148 w1186 w1291 w1410 w1530 w1650 w1769 w1888 w2004 w2139 w2615 w2648 w2724]
          tunnel: [w460 w617 w657 w700 w742 w890 w1057 w1074 w1110 w1148 w1185 w1290 w1409 w1529 w1649 w1768 w1887 w2004 w2139 w2615 w2648 w2724] -> w413
          tunnel: [w455 w604 w656 w699 w730 w875 w1056 w1073 w1109 w1147 w1184 w1289 w1408 w1519 w1648 w1767 w1886 w2003 w2128 w2614 w2647 w2723] -> w412
          tunnel: w411 -> [w456 w605 w656 w699 w736 w882 w1056 w1073 w1109 w1147 w1183 w1288 w1407 w1519 w1647 w1766 w1885 w2003 w2129 w2614 w2647 w2723]
          tunnel: w410 -> [_ _ _ _ _ _ _ _ _ _ w1173 w1287 w1406 w1528 w1646 w1765 w1884 _ _ _ _ _]
          tunnel: w395 -> [w470 w616 w655 w698 w739 w887 w1055 w1072 w1108 w1146 w1181 w1285 w1404 w1526 w1644 w1763 w1882 w2002 _ w2612 w2641 w2720]
          tunnel: [w474 w615 w654 w697 w718 w868 w1054 w1063 w1107 w1145 w1182 w1286 w1405 w1527 w1645 w1764 w1883 w2001 w2135 _ w2642 w2721] -> w409
          tunnel: w397 -> [w474 w615 w654 w697 w719 w868 w1054 w1064 w1107 w1145 w1182 w1286 w1405 w1527 w1645 w1764 w1883 w2001 w2137 w2611 w2645 w2712]
          tunnel: [_ _ _ _ _ _ _ _ _ _ _ _ _ _ _ _ _ _ FALSE ("aborted?") FALSE ("aborted?") w2644 w2722] -> w408
          tunnel: [w466 w616 w655 w698 w739 w887 w1055 w1072 w1108 w1146 w1181 w1285 w1404 w1526 w1644 w1763 w1882 w2002 w2126 w2610 w2641 w2720] -> w405
          tunnel: [w473 w614 w653 w696 w741 w889 w1053 w1071 w1106 w1144 w1180 w1283 w1402 w1524 w1642 w1761 w1880 w1999 "Read String Pot" w2609 w2640 w2719] -> w402
          tunnel: w401 -> [w473 w614 w653 w696 w741 w889 w1053 w1071 w1106 w1144 w1180 w1283 w1402 w1524 w1642 w1761 w1880 w1999 _ w2609 w2640 w2719]
          tunnel: [w453 w606 w648 w692 w734 w879 w1052 w1070 w1105 w1143 w1179 w1282 w1401 w1523 w1641 w1760 w1879 w1998 w2132 w2608 w2639 w2718] -> w389
          tunnel: w400 -> [w454 w606 w649 w692 w711 w880 w1052 w1070 w1105 w1143 w1179 w1282 w1401 w1523 w1641 w1760 w1879 w1998 w2118 w2608 w2639 w2718]
          tunnel: [w472 w613 w652 w695 w740 w888 w1051 w1069 w1104 w1142 w1178 w1281 w1400 w1522 w1640 w1759 w1878 w1997 w2131 w2607 w2638 w2717] -> w399
          tunnel: w398 -> [w472 w613 w652 w695 w740 w888 w1051 w1069 w1104 w1142 w1178 w1281 w1400 w1522 w1640 w1759 w1878 w1997 _ w2607 w2638 w2717]
          tunnel: [w471 w612 w651 w694 w729 w874 w1050 w1068 w1103 w1141 w1171 w1280 w1399 w1521 w1639 w1758 w1877 w1996 w2122 w2606 w2633 w2716] -> w393
          tunnel: "Sonde Parameters \nInitial Values" -> [w471 w612 w651 w694 w729 w874 w1050 w1068 w1103 w1141 w1176 w1280 w1399 w1521 w1639 w1758 w1877 w1996 w2122 w2606 w2633 w2716]
          tunnel: w386 -> [w450 w608 w650 w693 w727 w872 w1049 w1067 w1102 w1140 w1175 w1279 w1398 w1520 w1638 w1757 w1876 w1995 w2121 w2605 w2632 w2715]
          tunnel: [w449 w607 w650 w693 w706 w862 w1049 w1067 w1102 w1140 w1175 w1279 w1398 w1520 w1638 w1757 w1876 w1995 w2121 w2605 w2632 w2715] -> w384
          tunnel: [w459 w610 w647 w691 w712 w866 w1048 w1066 w1101 w1139 w1172 w1278 w1397 w1518 w1637 w1756 w1875 w1993 w2119 w2604 w2631 w2714] -> w391
          tunnel: w390 -> [w458 w610 w647 w691 w712 w866 w1048 w1066 w1101 w1139 w1172 w1278 w1397 w1517 w1637 w1756 w1875 w1993 w2119 w2604 w2631 w2714]
          tunnel: [w451 w609 w646 w690 w708 w865 w1047 w1065 w1100 w1138 w1170 w1277 w1396 w1516 w1636 w1755 w1874 w1992 w2116 w2603 w2630 w2713] -> w388
          tunnel: w387 -> [w452 w609 w646 w690 w709 w864 w1047 w1065 w1100 w1138 w1170 w1277 w1396 w1516 w1636 w1755 w1874 w1992 w2116 w2603 w2630 w2713]
          frame "TimeOut", Default {
            n175 = case shown="True" "Update Sonde" {
              tunnel: w461 -> [w480 w487]
              tunnel: [w480 w486] -> w460
              tunnel: [w479 w485] -> w459
              tunnel: w458 -> [w479 w484]
              frame False {
              }
              frame True {
                n176 = flat-sequence {
                  tunnel: w483 -> [w505]
                  tunnel: [w504] -> w482
                  tunnel: w487 -> [w503]
                  tunnel: [w502] -> w486
                  tunnel: [w501] -> w485
                  tunnel: w484 -> [w500]
                  tunnel: [w490] -> _
                  tunnel: [w499] -> _
                  tunnel: w481 -> [w498]
                  frame #0 {
                    n177 = control-ref of="Found Quanta Sonde Com Port"() -> (w497:refnum<vi>)
                    n178 = control-ref of="Temperature"() -> (w494:refnum<vi>)
                    n179 = control-ref of="Sonde Data Display"() -> (w496:refnum<vi>)
                    n180 = control-ref of="Sonde Data Display Graphs"() -> (w495:refnum<vi>)
                    n181 = control-ref of="Current Time (s)"() -> (w493:refnum<vi>)
                    n182 = local read "Sample Sheet Data Row Cluster 2"() -> (w491:T2)
                    n183 = Unbundle By Name(w491) -> ("Sonde Data Cluster.Cumulative\nVolume (ml)"=w488:dbl)
                    n184 = call "Sonde Single Measurement Subvi.vi"("VISAResourceName in"=w497, "Time Array"=w503, "Cumulative Sonde Data"=w500, "Previous time"=w498, "Sonde Data Display"=w496, "Sonde Graph in"=w495, "Temp Graph 3"=w494, "error in (no error)"=w505, "Row Cluster Input"=w491, "reference 5"=w493) -> ("seconds since 1Jan1904"=w499:timestamp, "Cumulative Sonde \nData Out"=w501:dbl[][], "Sample Sheet Data Row Cluster 2"=w490:T2, "output cluster"=w492:T1, "time array out"=w502:dbl[], "error out"=w504:errorcluster)
                    n185 = Bundle By Name(cluster=w490, "Sonde Data Cluster.Cumulative\nVolume (ml)"=w488) -> (w489:T2)
                    n186 = local write "output cluster"(w492) -> ()
                    n187 = local write "Sample Sheet Data Row Cluster 2"(w489) -> ()
                  }
                }
                n188 = local read "Current Time (s)"() -> (w481:dbl)
                n189 = local write "Sonde Communication Error Out"(w482) -> ()
                n190 = local read "Sonde Communication Error Out"() -> (w483:errorcluster)
              }
            }
            n191 = property on="Current Session" class="Arr (strict)"() -> ("Index Values"=w448:u32[])  [unwired: 2 in, 2 out]
            n192 = property on="KPRO test report header" class="Arr (strict)"("Index Values"=w448) -> ()  [unwired: 2 in, 2 out]
            n193 = flat-sequence {
              tunnel: w467 -> [w544]
              tunnel: w456 -> [w523]
              tunnel: w465 -> [w543]
              tunnel: w454 -> [w527]
              tunnel: [w542] -> w453
              tunnel: w464 -> [w541]
              tunnel: w466 -> [w535]
              tunnel: [w534] -> _
              tunnel: [w506] -> w455
              tunnel: [w528] -> _
              tunnel: w463 -> [w520]
              tunnel: w462 -> [w517]
              tunnel: w452 -> [w516]
              tunnel: [w507] -> w451
              tunnel: w450 -> [w511]
              tunnel: [w510] -> w449
              frame #0 {
                # "Timeout"
                n194 = Unbundle By Name(w527) -> ("Current Relative Depth"=w526:dbl)
                n195 = flat-sequence {
                  tunnel: w525 -> [w554]
                  frame #0 {
                    n196 = local read "Corrected Pressure Cluster"() -> (w556:T20)
                    n197 = Divide(x=w554, y=3.281) -> (x/y=w555:dbl)
                    n198 = local write "Current \nDepth (m)"(w555) -> ()
                    n199 = local write "Current Depth"(w554) -> ()
                    n200 = local read "Sample Sheet Data Row Cluster 2"() -> (w558:T2)
                    n201 = global write "Kpro Globals.vi" "Current Depth"(w554) -> ()
                    n202 = Unbundle By Name(w556) -> ("Up hole Corrected Pressure"=w553:dbl)
                    "Uphole Pressure" <- w553
                    n203 = Bundle By Name(cluster=w558, "Depth"=w554, "Head\nPressure"=w553) -> (w557:T2)
                    n204 = local write "Sample Sheet Data Row Cluster 2"(w557) -> ()
                  }
                }
                n205 = local read "KPRO Session Output File Path"() -> (w528:path)
                n206 = local read "KPRO Finish\nIndicator"() -> (w522:bool)
                n207 = local read "Depth mode"() -> (w524:bool)
                n208 = local read "Input Variables and Slopes"() -> (w540:T11)
                n209 = Unbundle By Name(w540) -> ("String Pot Slope"=w539:dbl)
                n210 = local read "Input Depths \nand Parameters Cluster"() -> (w538:T16)
                n211 = Unbundle By Name(w538) -> ()  [unwired: 1 out]
                n212 = local read "Uphole Pressure"() -> (w512:dbl)
                n213 = call "Kpro Read String Pot 2016.vi"("Read String Pot"=w524, "Feet of\nStainless to be\nUsed (Count) in"=w511, "Session Array in"=w516, "Flow"=w541, "Manual Depth In"=w526, "Finished In"=w522, "Depth Cluster in"=w527, "error in (no error)"=w517, "String Pot \nSlope in"=w539, "Sensor Cluster In in"=w543, "Descriptions"=w544, "Pressure in"=w512, "Array in"=w535, "Downhole Pressure Sensor"=w520, "Initial Measurement Input"=FALSE) -> ("Sensor Cluster 2"=w536:T9, "IK"=w519:dbl, "Array out"=w534:refnum<k24>[], "Generate Array Calc IK"=w508:bool, "Feet of\nStainless to be\nUsed (Count) out"=w510:i32, "Depth Cluster out"=w542:T17, "Single String Pot Session Array out"=w507:dbl[][])  [unwired: 4 in, 2 out]
                n214 = Unbundle By Name(w542) -> ("Current Absolute Depth"=w525:dbl)
                n215 = Bundle By Name(cluster=w538, "Feet of Stainless"=w510) -> (w537:T16)
                n216 = local write "Sensor Voltage Cluster"(w536) -> ()
                n217 = local write "Input Depths \nand Parameters Cluster"(w537) -> ()
                n218 = local write "Ik"(w519) -> ()
                n219 = local read "Input Depths \nand Parameters Cluster"() -> (w530:T16)
                n220 = Unbundle By Name(w530) -> ("Flow"=→"Flow":dbl)
                n221 = And(x=w508, y=w524) -> ()  [unwired: 1 out]
                n222 = case shown="True" FALSE {
                  tunnel: w523 -> [w549 w552]
                  tunnel: w507 -> [_ w550]
                  tunnel: [w549 w551] -> w506
                  frame False {
                  }
                  frame True {
                    n223 = Build Array (concatenate)(w552, w550) -> (w551:dbl[][])
                  }
                }
                n224 = call "Array to Plot 2016.vi"("Input Cumulative Array"=w506, "Input Real Time Array"=w507) -> ("Cumulative - Depth vs.Drive Rate"=w513:cluster{dbl[], dbl[]}, "Cumulative - Depth vs. Ik"=w531:cluster{dbl[], dbl[]}, "Real Time - Depth vs. Drive Rate"=w514:cluster{dbl[], dbl[]}, "Real Time - Depth vs. Ik"=w521:cluster{dbl[], dbl[]}, "Depth Rate"=w518:dbl)  [unwired: 2 in, 1 out]
                n225 = local write "Depth Rate\nft/min"(w518) -> ()
                n226 = case shown="True" w508 {
                  tunnel: w507 -> [_ w546]
                  tunnel: w506 -> [_ w545]
                  frame False {
                  }
                  frame True {
                    n227 = control-ref of="KPRO Session Output File Path"() -> (w548:refnum<vi>)
                    n228 = control-ref of="KPRO Cumulative Output File Path"() -> (w547:refnum<vi>)
                    n229 = call "write KPRO file.vi"("Corrected Array in"=w546, "Path in"=w548) -> ()  [unwired: 8 in, 2 out]
                    n230 = call "write KPRO file.vi"("Corrected Array in"=w545, "Path in"=w547) -> ()  [unwired: 8 in, 2 out]
                  }
                }
                n231 = local write "Large Depth IK Graph Cluster"(w521) -> ()
                n232 = local write "Cumulative_data_from_file"(w506) -> ()
                n233 = local read "Culmulative Graph Cluster"() -> (w533:T19)
                n234 = Bundle By Name(cluster=w533, "Cumulative - Depth vs. Ik"=w531, "Real Time - Depth vs. lk"=w521, "Cumulative - Depth vs. Drive Rate"=w513, "Real Time - Depth vs. Drive Rate"=w514) -> (w532:T19)
                n235 = local write "Culmulative Graph Cluster"(w532) -> ()
                n236 = local write "Current Session"(w507) -> ()
              }
            }
            n237 = flat-sequence {
              tunnel: w469 -> [w566]
              tunnel: w468 -> [w569]
              tunnel: [w565] -> w465
              tunnel: [w566] -> w467
              tunnel: [w562] -> w464
              tunnel: [w564] -> w466
              frame #0 {
                w570 = 0.0  # Offset
                n238 = local read "Input Depths \nand Parameters Cluster"() -> (w572:T16)
                n239 = local read "Input Variables and Slopes"() -> (w568:T11)
                n240 = Unbundle By Name(w568) -> ("Flow Slope"=w567:dbl)
                n241 = call "Flow 2016.vi"("Descriptions"=w566, "Array in"=w569, "Flow Slope"=w567, "Offset"=w570) -> ("Sensor Cluster"=w565:T9, "Flow (ml/min)"=w562:dbl, "Array out"=w564:refnum<k24>[])  [unwired: 4 in]
                n242 = Bundle By Name(cluster=w572, "Flow"=w562) -> (w571:T16)
                n243 = local write "Input Depths \nand Parameters Cluster"(w571) -> ()
                n244 = local write "Sensor Voltage Cluster"(w565) -> ()
                n245 = local read "Input Depths \nand Parameters Cluster"() -> (w561:T16)
                n246 = Unbundle By Name(w561) -> ("Feet of Stainless"=w560:i32)
                n247 = call "pressure and IK2 2016.vi"("Ft. of SS"=w560, "flow"=w562) -> ("IK"=→"Large Depth IK Graph":dbl)  [unwired: 1 in, 1 out]
              }
            }
            n248 = flat-sequence {
              tunnel: w470 -> [w579]
              tunnel: [w575] -> w469
              tunnel: [w574] -> w468
              frame #0 {
                n249 = local read "Descriptions"() -> (w575:string[])
                n250 = local read "Input Variables and Slopes"() -> (w582:T11)
                n251 = Unbundle By Name(w582) -> ("Up Hole Pressure Slope"=w581:dbl, "Up Hole  Pressure Offset"=w578:dbl)
                n252 = local write "Input Variables and Slopes"(w582) -> ()
                n253 = local read "Sensor Voltage Cluster"() -> (w583:T9)
                n254 = call "up hole Pressure 2016.vi"("Sensor Cluster"=w583, "Pressure Offset"=w578, "Array in"=w579, "Pressure \nSlope"=w581, "Descriptions"=w575, "Zero Pressure\n(F = leave as is)"=TRUE) -> ("Array out"=w574:refnum<k24>[], "Uphole Pressure"=w573:dbl, "Sensor Cluster 2"=w580:T9)  [unwired: 6 in, 1 out]
                n255 = local write "Sensor Voltage Cluster"(w580) -> ()
                n256 = local write "Uphole Pressure"(w573) -> ()
                n257 = local read "Corrected Pressure Cluster"() -> (w577:T20)
                n258 = Bundle By Name(cluster=w577, "Up hole Corrected Pressure"=w573) -> (w576:T20)
                n259 = local write "Corrected Pressure Cluster"(w576) -> ()
              }
            }
            n260 = flat-sequence {
              tunnel: [w591] -> _
              tunnel: [w595] -> w463
              tunnel: [w603] -> _
              tunnel: [w602] -> _
              tunnel: w470 -> [w601]
              tunnel: [w600] -> _
              frame #0 {
                n261 = local read "Input Variables and Slopes"() -> (w597:T11)
                n262 = Unbundle By Name(w597) -> ("DH Pressure Trans Slope"=w603:dbl, "DH Pressure Offset"=w602:dbl)
                n263 = global read "Kpro Globals.vi" "Current Depth"() -> (w591:sgl)
                n264 = local read "Sensor Voltage Cluster"() -> (w598:T9)
                n265 = local read "Descriptions"() -> (w599:string[])
                n266 = local read "Zero In-Line Pressure\n(F = leave as is)"() -> (w596:bool)
                n267 = call "DHT Pressure 2016.vi"("Sensor Cluster"=w598, "DHT Pressure Offset"=w602, "Array in"=w601, "DHT Pressure \nSlope"=w603, "Descriptions"=w599, "Zero Pressure\n(F = leave as is)"=w596) -> ("Array out"=w600:refnum<k24>[], "DHT Pressure"=w595:dbl, "Sensor Cluster 2"=w592:T9)  [unwired: 7 in]
                n268 = Add(x=w595, y=w591) -> ()  [unwired: 1 out]
                n269 = local write "Down hole Pressure"(w595) -> ()
                n270 = local write "Sensor Voltage Cluster"(w592) -> ()
                n271 = local read "Sensor  Real \nMeasurements"() -> (w594:T6)
                n272 = local read "Input Variables and Slopes"() -> (w593:T11)
                n273 = call "convert sensor voltage to real measurements.vi"("Input Variables and Slopes"=w593, "Sensor  Real Measurements in"=w594, "Sensor Cluster"=w592) -> ("Sensor  Real Measurements out"=w588:T9)  [unwired: 8 in]
                n274 = Unbundle By Name(w588) -> ("Aux 1"=w587:dbl, "Aux 2"=w586:dbl, "Aux 3"=w585:dbl)
                n275 = local write "Sensor  Real \nMeasurements"(w588) -> ()
                n276 = local read "Sample Sheet Data Row Cluster 2"() -> (w590:T2)
                n277 = Bundle By Name(cluster=w590, "Aux1"=w587, "Aux2"=w586, "Aux3"=w585) -> (w589:T2)
                n278 = local write "Sample Sheet Data Row Cluster 2"(w589) -> ()
              }
            }
          }
          frame "Finish KPRO Measurements" {
            n279 = flat-sequence {
              tunnel: w606 -> [w624]
              tunnel: [w635] -> w604
              tunnel: w605 -> [w632]
              tunnel: w609 -> [w626]
              tunnel: w608 -> [w625]
              tunnel: [w623] -> _
              tunnel: [w622] -> w607
              frame #0 {
                n280 = Build Array (concatenate)(w632, w626) -> (w627:dbl[][])
                n281 = local read "Input Depths \nand Parameters Cluster"() -> (w634:T16)
                n282 = Unbundle By Name(w634) -> ()  [unwired: 1 out]
                n283 = local read "KPRO Session Output File Path"() -> (w630:path)
                n284 = case shown="True" TRUE {
                  tunnel: w630 -> [w636 w645]
                  tunnel: errorcluster {"status"=FALSE, "code"=0, "source"=""} ("error constant") -> [w637 w642]
                  tunnel: [w637 w641] -> _
                  tunnel: [w636 w638] -> w629
                  frame False {
                  }
                  frame True {
                    n285 = call-poly <vilib>:"Write Delimited Spreadsheet.vi"("file path (dialog if empty)"=w645, "1D data"="KPRO test report header", "append to file? (new file:F)"=FALSE, "error in (no error)"=w642, "transpose? (no:F)"=FALSE, "delimiter (\\t)"="," ("delimiter (\\t)")) -> ("new file path (Not A Path if cancelled)"=w638:path, "error out"=w641:errorcluster)  [unwired: 8 in]
                  }
                }
                n286 = call "Finished Collection Write File.vi"("Cluster in"=w624, "Corrected Array in"=w627, "Feet of\nStainless to be\nUsed (Count) in"=w625, "Output KPRO"=w629) -> ("Corrected Array out"=w635:dbl[][], "Depth to \nbe Used \n(Feet)"=w623:sgl, "Feet of\nStainless to be\nUsed (Count) out"=w622:i32)  [unwired: 5 in]
                n287 = Bundle By Name(cluster=w634, "Feet of Stainless"=w622) -> (w633:T16)
                n288 = local write "Input Depths \nand Parameters Cluster"(w633) -> ()
                n289 = local write "Current Depth"(w623) -> ()
              }
            }
          }
          frame "Update Depth" {
            n290 = flat-sequence {
              tunnel: w649 -> [w674]
              tunnel: [w671] -> w648
              frame #0 {
                n291 = Unbundle By Name(w674) -> ("First Absolute Depth"=w672:dbl)
                n292 = local read "Current Depth"() -> (w668:sgl)
                n293 = local read "Read String Pot"() -> (w663:bool)
                n294 = Greater?(x="New Depth", y=w668) -> (0:w667:bool)
                n295 = local read "Sensor  Real \nMeasurements"() -> (w675:T6)
                n296 = Unbundle By Name(w675) -> ("String Pot"=w664:dbl)
                n297 = case shown="False" w667 {
                  tunnel: [w684 w689] -> w673
                  tunnel: w672 -> [w683 w688]
                  tunnel: "New Depth" -> [w681 w686]
                  tunnel: w668 -> [w680 w685]
                  frame True {
                    n298 = Subtract(x=w680, y=w681) -> (x-y=w682:dbl)
                    n299 = Subtract(x=w683, y=w682) -> (x-y=w684:dbl)
                  }
                  frame False {
                    # "Reverse inputs \non Subtraction"
                    n300 = Subtract(x=w686, y=w685) -> (x-y=w687:dbl)
                    n301 = Subtract(x=w688, y=w687) -> (x-y=w689:dbl)
                  }
                }
                n302 = Bundle By Name(cluster=w674, "Absolute Depth In"="New Depth", "Current Absolute Depth"="New Depth", "First Absolute Depth"=w673) -> (w666:T17)
                n303 = case shown="False" w663 {
                  tunnel: w666 -> [w676 w679]
                  tunnel: [w676 w678] -> w665
                  tunnel: w664 -> [_ w677]
                  frame False {
                  }
                  frame True {
                    n304 = Bundle By Name(cluster=w679, "Current Relative Depth"=w677) -> (w678:T17)
                  }
                }
                n305 = call "calculate current depth.vi"("Cluster in"=w665) -> ("Cluster out"=w671:T17)  [unwired: 10 in]
                n306 = Unbundle By Name(w671) -> ("Current Absolute Depth"=w670:dbl)
                n307 = local write "Current Depth"(w670) -> ()
                n308 = global write "Kpro Globals.vi" "Current Depth"(w670) -> ()
              }
            }
          }
          frame "IK vs Time" {
          }
          frame "Start KPRO Measurements" {
            n309 = flat-sequence {
              tunnel: w714 -> [w767]
              tunnel: [w766] -> w713
              frame #0 {
                w768 = 15  # Filter Size
                # "Functional Global in \nBoxcar Integrator\nInitialize filter array to \ncurrent string pot value"
                n310 = call "Boxcar filter2016.vi"("Initialize"=TRUE, "Filter Size"=w768, "Filter Input"=w767) -> ("Filter Output"=w766:dbl)
              }
            }
            n311 = flat-sequence {
              tunnel: [w770] -> w715
              frame #0 {
                n312 = Tick Count (ms)() -> (millisecond timer value=w772:u32)
                n313 = Divide(x=w772, y=u32 1000) -> (x/y=w770:dbl)
              }
            }
            n314 = local read "Input Variables and Slopes"() -> (w717:T11)
            n315 = Unbundle By Name(w717) -> ("String Pot Slope"=w716:dbl)
            n316 = call "depth read from string pot 2016.vi"("Descriptions"=w722, "error in (no error)"=w719, "String Pot \nSlope"=w716, "Array in"=w721) -> ("Array out"=w720:refnum<k24>[], "Depth"=w714:dbl, "error out"=w718:errorcluster)  [unwired: 12 in, 1 out]
            n317 = flat-sequence {
              tunnel: [w777] -> w710
              tunnel: w713 -> [w774]
              tunnel: w715 -> [w776]
              tunnel: w711 -> [w775]
              frame #0 {
                n318 = local read "Current Depth"() -> (w773:sgl)
                n319 = Bundle By Name(cluster=w775, "Previous Relative Depth"=w774, "Current Relative Depth"=w774, "First Relative Depth"=w774, "Current Measurement Time"=w776, "Previous Measurement Time"=w776, "Absolute Depth In"=w773, "Current Absolute Depth"=w773, "First Absolute Depth"=w773) -> (w777:T17)
              }
            }
            n320 = flat-sequence {
              tunnel: w737 -> [w828]
              tunnel: w736 -> [w808]
              tunnel: w735 -> [w827]
              tunnel: w710 -> [w826]
              tunnel: [w825] -> w734
              tunnel: w733 -> [w824]
              tunnel: w731 -> [w818]
              tunnel: [w817] -> _
              tunnel: [w799] -> w730
              tunnel: w723 -> [w812]
              tunnel: w709 -> [w803]
              tunnel: [w800] -> w708
              tunnel: w707 -> [w796]
              tunnel: [w794] -> w706
              frame #0 {
                n321 = control-ref of="KPRO Session Output File Path"() -> (w811:refnum<vi>)
                n322 = flat-sequence {
                  tunnel: w807 -> [w833]
                  frame #0 {
                    n323 = local read "Corrected Pressure Cluster"() -> (w836:T20)
                    n324 = Divide(x=w833, y=3.281) -> (x/y=w834:dbl)
                    n325 = local write "Current \nDepth (m)"(w834) -> ()
                    n326 = local write "Current Depth"(w833) -> ()
                    n327 = local read "Sample Sheet Data Row Cluster 2"() -> (w838:T2)
                    n328 = global write "Kpro Globals.vi" "Current Depth"(w833) -> ()
                    n329 = Unbundle By Name(w836) -> ("Up hole Corrected Pressure"=w835:dbl)
                    n330 = Bundle By Name(cluster=w838, "Depth"=w833, "Head\nPressure"=w835) -> (w837:T2)
                    n331 = local write "Sample Sheet Data Row Cluster 2"(w837) -> ()
                  }
                }
                n332 = local read "KPRO Finish\nIndicator"() -> (w813:bool)
                n333 = local read "Depth mode"() -> (w809:bool)
                n334 = local read "Input Variables and Slopes"() -> (w823:T11)
                n335 = Unbundle By Name(w823) -> ("String Pot Slope"=w822:dbl)
                n336 = local read "Input Depths \nand Parameters Cluster"() -> (w821:T16)
                n337 = Unbundle By Name(w821) -> ()  [unwired: 1 out]
                n338 = local read "Culmulative Graph Cluster"() -> (w816:T19)
                n339 = Build Array (concatenate)(w808, w803) -> (w804:dbl[][])
                n340 = local read "Uphole Pressure"() -> (w795:dbl)
                n341 = call "Kpro Read String Pot 2016.vi"("Read String Pot"=w809, "Feet of\nStainless to be\nUsed (Count) in"=w796, "Session Array in"=dbl[][] [], "Flow"=w824, "Finished In"=w813, "Depth Cluster in"=w826, "String Pot \nSlope in"=w822, "Sensor Cluster In in"=w827, "Descriptions"=w828, "Pressure in"=w795, "Array in"=w818, "Downhole Pressure Sensor"=w812, "Initial Measurement Input"=TRUE) -> ("Sensor Cluster 2"=w819:T9, "Array out"=w817:refnum<k24>[], "Generate Array Calc IK"=w801:bool, "Feet of\nStainless to be\nUsed (Count) out"=w794:i32, "Depth Cluster out"=w825:T17, "Single String Pot Session Array out"=w800:dbl[][])  [unwired: 6 in, 3 out]
                n342 = Bundle By Name(cluster=w821, "Feet of Stainless"=w794) -> (w820:T16)
                n343 = Unbundle By Name(w825) -> ("Current Absolute Depth"=w807:dbl)
                n344 = local write "Sensor Voltage Cluster"(w819) -> ()
                n345 = local write "Input Depths \nand Parameters Cluster"(w820) -> ()
                n346 = case shown="True" FALSE {
                  tunnel: w800 -> [_ w832]
                  tunnel: [w829 w831] -> w799
                  tunnel: w804 -> [w829 w830]
                  frame False {
                  }
                  frame True {
                    n347 = Build Array (concatenate)(w830, w832) -> (w831:dbl[][])
                  }
                }
                n348 = call "Array to Plot 2016.vi"("Input Cumulative Array"=w799, "Input Real Time Array"=w800) -> ("Cumulative - Depth vs.Drive Rate"=w798:cluster{dbl[], dbl[]}, "Cumulative - Depth vs. Ik"=w814:cluster{dbl[], dbl[]}, "Real Time - Depth vs. Drive Rate"=w797:cluster{dbl[], dbl[]}, "Real Time - Depth vs. Ik"=w810:cluster{dbl[], dbl[]}, "Depth Rate"=w806:dbl)  [unwired: 2 in, 1 out]
                n349 = Bundle By Name(cluster=w816, "Cumulative - Depth vs. Ik"=w814, "Real Time - Depth vs. lk"=w810, "Cumulative - Depth vs. Drive Rate"=w798, "Real Time - Depth vs. Drive Rate"=w797) -> (w815:T19)
                n350 = local write "Depth Rate\nft/min"(w806) -> ()
                n351 = local write "Culmulative Graph Cluster"(w815) -> ()
                n352 = call "write KPRO file.vi"("Corrected Array in"=w799, "Generate Array Calc IK"=w801, "Path in"=w811) -> ()  [unwired: 7 in, 2 out]
                n353 = local write "Large Depth IK Graph Cluster"(w810) -> ()
                n354 = local write "Cumulative_data_from_file"(w799) -> ()
                n355 = local write "Current Session"(w800) -> ()
              }
            }
            n356 = flat-sequence {
              tunnel: w738 -> [w856]
              tunnel: [w852] -> w722
              tunnel: [w851] -> w721
              frame #0 {
                n357 = local read "Descriptions"() -> (w852:string[])
                n358 = local read "Input Variables and Slopes"() -> (w859:T11)
                n359 = Unbundle By Name(w859) -> ("Up Hole Pressure Slope"=w858:dbl, "Up Hole  Pressure Offset"=w855:dbl)
                n360 = local write "Input Variables and Slopes"(w859) -> ()
                n361 = local read "Sensor Voltage Cluster"() -> (w860:T9)
                n362 = call "up hole Pressure 2016.vi"("Sensor Cluster"=w860, "Pressure Offset"=w855, "Array in"=w856, "Pressure \nSlope"=w858, "Descriptions"=w852, "Zero Pressure\n(F = leave as is)"=TRUE) -> ("Array out"=w851:refnum<k24>[], "Uphole Pressure"=w850:dbl, "Sensor Cluster 2"=w857:T9)  [unwired: 6 in, 1 out]
                n363 = local write "Sensor Voltage Cluster"(w857) -> ()
                n364 = local write "Uphole Pressure"(w850) -> ()
                n365 = local read "Corrected Pressure Cluster"() -> (w854:T20)
                n366 = Bundle By Name(cluster=w854, "Up hole Corrected Pressure"=w850) -> (w853:T20)
                n367 = local write "Corrected Pressure Cluster"(w853) -> ()
              }
            }
            n368 = flat-sequence {
              tunnel: w728 -> [w755]
              tunnel: w727 -> [w754]
              tunnel: [w753] -> w726
              tunnel: [w752] -> w725
              tunnel: [w749] -> w707
              frame #0 {
                n369 = local read "Input Depths \nand Parameters Cluster"() -> (w751:T16)
                n370 = local read "Input Variables and Slopes"() -> (w747:T11)
                n371 = Unbundle By Name(w747) -> ("Depth to Water Table"=w748:dbl)
                n372 = disable-structure shown="Enabled" {
                  disable-tunnel: w748 -> [w762 w763]
                  disable-tunnel: [w761 w763] -> w746
                  disable-tunnel: w755 -> [w760 w765]
                  disable-tunnel: [w759 w765] -> w752
                  disable-tunnel: w754 -> [w758 w764]
                  disable-tunnel: [w757 w764] -> w749
                  frame Enabled {
                    n373 = call <vilib>:"Clear Errors.vi"("error in (no error)"=w760) -> ("error out"=w756:errorcluster)  [unwired: 5 in, 1 out]
                    n374 = call "New Stainless Correction Pop Up 2016.vi"("error in (no error)"=w756, "New Feet\n of Stainless\n(Count)"=w758, "Depth to \nWater Table\nInput"=w762) -> ("error in (no error) 2"=w759:errorcluster, "Feet of\nStainless to be\nUsed (Count)"=w757:i32, "Depth to \nWater Table\nOutput"=w761:dbl)  [unwired: 6 in]
                  }
                  frame Disabled {
                  }
                }
                n375 = Bundle By Name(cluster=w747, "Depth to Water Table"=w746) -> (w753:T11)
                n376 = Bundle By Name(cluster=w751, "Feet of Stainless"=w749) -> (w750:T16)
                n377 = local write "Input Depths \nand Parameters Cluster"(w750) -> ()
              }
            }
            n378 = flat-sequence {
              tunnel: w722 -> [w843]
              tunnel: w720 -> [w846]
              tunnel: [w841] -> w735
              tunnel: [w843] -> w737
              tunnel: [w842] -> w733
              tunnel: [w840] -> w731
              frame #0 {
                w847 = 0.0  # Offset
                n379 = local read "Input Depths \nand Parameters Cluster"() -> (w849:T16)
                n380 = local read "Input Variables and Slopes"() -> (w845:T11)
                n381 = Unbundle By Name(w845) -> ("Flow Slope"=w844:dbl)
                n382 = call "Flow 2016.vi"("Descriptions"=w843, "Array in"=w846, "Flow Slope"=w844, "Offset"=w847) -> ("Sensor Cluster"=w841:T9, "Flow (ml/min)"=w842:dbl, "Array out"=w840:refnum<k24>[])  [unwired: 4 in]
                n383 = Bundle By Name(cluster=w849, "Flow"=w842) -> (w848:T16)
                n384 = local write "Input Depths \nand Parameters Cluster"(w848) -> ()
                n385 = local write "Sensor Voltage Cluster"(w841) -> ()
              }
            }
            n386 = flat-sequence {
              tunnel: w739 -> [w792]
              tunnel: [w791] -> w738
              tunnel: w726 -> [w790]
              tunnel: w725 -> [w789]
              tunnel: [w788] -> w724
              tunnel: [w779] -> w723
              frame #0 {
                n387 = control-ref of="Zero In-Line Pressure\n(F = leave as is)"() -> (w782:refnum<vi>)
                n388 = control-ref of="Input Variables and Slopes"() -> (w785:refnum<vi>)
                n389 = control-ref of="Sensor Voltage Cluster"() -> (w783:refnum<vi>)
                n390 = control-ref of="Descriptions"() -> (w784:refnum<vi>)
                n391 = control-ref of="Down hole Pressure Transducer CSV"() -> (w786:refnum<vi>)
                n392 = property on="Large Depth IK Graph" class="WFChart (strict)"("History Data"=dbl[] []) -> ()  [unwired: 2 in, 2 out]
                n393 = invoke on="Update Sonde" class="Bool (strict)" method="Reinit To Default"() -> ()  [unwired: 3 in, 3 out]
                n394 = local read "Corrected Pressure Cluster"() -> (w781:T20)
                n395 = call "measure down hole pressure and save to csv file.vi"("Path in"=w786, "reference 3"=w784, "reference in"=w785, "reference 4"=w783, "reference 5"=w782, "Record DTW File"="Record DTW File", "error in (no error)"=w789, "Array in"=w792, "Input Variables and Slopes"=w790) -> ("Array out"=w791:refnum<k24>[], "In-Line Pressure"=w779:dbl, "error out"=w788:errorcluster)  [unwired: 3 in, 1 out]
                "Down hole Pressure" <- w779
                n396 = Bundle By Name(cluster=w781, "Down hole Corrected Pressure"=w779) -> (w780:T20)
                n397 = local write "Corrected Pressure Cluster"(w780) -> ()
              }
            }
          }
          frame "Increment Depth Manually" {
            n398 = disable-structure shown="Enabled" {
              disable-tunnel: w873 -> [w898 w916]
              disable-tunnel: w872 -> [w897 _]
              disable-tunnel: [w896 _] -> w863
              disable-tunnel: [w895 w917] -> w871
              disable-tunnel: [w894 w916] -> w870
              frame Disabled {
                n399 = flat-sequence {
                  tunnel: w898 -> [w906]
                  tunnel: [w905] -> w894
                  tunnel: w897 -> [w904]
                  tunnel: [w903] -> w896
                  tunnel: [w899] -> w895
                  frame #0 {
                    n400 = local read "Input Variables and Slopes"() -> (w901:T11)
                    n401 = Unbundle By Name(w901) -> ("Depth to Water Table"=w902:dbl)
                    n402 = disable-structure shown="Enabled" {
                      disable-tunnel: w902 -> [w912 w913]
                      disable-tunnel: [w911 w913] -> w900
                      disable-tunnel: w906 -> [w910 w915]
                      disable-tunnel: [w909 w915] -> w905
                      disable-tunnel: w904 -> [w908 w914]
                      disable-tunnel: [w907 w914] -> w903
                      frame Enabled {
                        n403 = call "New Stainless Correction Pop Up 2016.vi"("error in (no error)"=w910, "New Feet\n of Stainless\n(Count)"=w908, "Depth to \nWater Table\nInput"=w912) -> ("error in (no error) 2"=w909:errorcluster, "Feet of\nStainless to be\nUsed (Count)"=w907:i32, "Depth to \nWater Table\nOutput"=w911:dbl)  [unwired: 6 in]
                      }
                      frame Disabled {
                      }
                    }
                    n404 = Bundle By Name(cluster=w901, "Depth to Water Table"=w900) -> (w899:T11)
                  }
                }
              }
              frame Enabled {
                n405 = local read "Input Variables and Slopes"() -> (w917:T11)
              }
            }
            n406 = flat-sequence {
              tunnel: w883 -> [w964]
              tunnel: w882 -> [w936]
              tunnel: w881 -> [w963]
              tunnel: w880 -> [w921]
              tunnel: [w962] -> w879
              tunnel: w878 -> [w961]
              tunnel: w876 -> [w955]
              tunnel: [w954] -> _
              tunnel: [w928] -> w875
              tunnel: w868 -> [w950]
              tunnel: w867 -> [w943]
              tunnel: [w927] -> w865
              tunnel: w864 -> [w934]
              tunnel: w863 -> [w923]
              tunnel: [w922] -> w862
              frame #0 {
                n407 = control-ref of="KPRO Session Output File Path"() -> (w929:refnum<vi>)
                n408 = control-ref of="KPRO Cumulative Output File Path"() -> (w918:refnum<vi>)
                n409 = Unbundle By Name(w921) -> ("Current Relative Depth"=w944:dbl)
                n410 = Unbundle By Name(w921) -> ("Current Absolute Depth"=w920:dbl)
                n411 = flat-sequence {
                  tunnel: w938 -> [w973]
                  frame #0 {
                    n412 = local read "Corrected Pressure Cluster"() -> (w976:T20)
                    n413 = local read "Sample Sheet Data Row Cluster 2"() -> (w978:T2)
                    n414 = Divide(x=w973, y=3.281) -> (x/y=w974:dbl)
                    n415 = local write "Current \nDepth (m)"(w974) -> ()
                    n416 = local write "Current Depth"(w973) -> ()
                    n417 = global write "Kpro Globals.vi" "Current Depth"(w973) -> ()
                    n418 = Unbundle By Name(w976) -> ("Up hole Corrected Pressure"=w975:dbl)
                    n419 = Bundle By Name(cluster=w978, "Depth"=w973, "Head\nPressure"=w975) -> (w977:T2)
                    n420 = local write "Sample Sheet Data Row Cluster 2"(w977) -> ()
                  }
                }
                n421 = local read "Depth mode"() -> (w933:bool)
                n422 = local read "KPRO Finish\nIndicator"() -> (w947:bool)
                n423 = global read "Kpro Globals.vi" "increment_amount"() -> (w948:dbl)
                n424 = local read "Input Variables and Slopes"() -> (w960:T11)
                n425 = Unbundle By Name(w960) -> ("String Pot Slope"=w959:dbl)
                n426 = local read "Input Depths \nand Parameters Cluster"() -> (w958:T16)
                n427 = Unbundle By Name(w958) -> ()  [unwired: 2 out]
                n428 = local read "Culmulative Graph Cluster"() -> (w953:T19)
                n429 = First Call?() -> ()  [unwired: 1 out]
                n430 = local read "Uphole Pressure"() -> (w924:dbl)
                n431 = local read "Input Depths \nand Parameters Cluster"() -> (w946:T16)
                n432 = Unbundle By Name(w946) -> ("Start Depth"=w945:sgl)
                n433 = Equal?(x=w920, y=w945) -> (x = y?=w941:bool)
                n434 = And(x=w941, y=FALSE) -> (x .and. y?=w942:bool)
                n435 = case shown="True" w942 {
                  tunnel: w944 -> [w967 w968]
                  tunnel: [w966 w968] -> w949
                  tunnel: w948 -> [w965 _]
                  frame False {
                    n436 = Add(x=w965, y=w967) -> (x+y=w966:dbl)
                  }
                  frame True {
                  }
                }
                n437 = call "Kpro Read String Pot 2016.vi"("Read String Pot"=w933, "Feet of\nStainless to be\nUsed (Count) in"=w923, "Session Array in"=w934, "Flow"=w961, "Manual Depth In"=w949, "Finished In"=w947, "Depth Cluster in"=w921, "error in (no error)"=w950, "String Pot \nSlope in"=w959, "Sensor Cluster In in"=w963, "Descriptions"=w964, "Pressure in"=w924, "Array in"=w955, "Downhole Pressure Sensor"=w943, "Initial Measurement Input"=FALSE) -> ("Sensor Cluster 2"=w956:T9, "IK"=w935:dbl, "Array out"=w954:refnum<k24>[], "Generate Array Calc IK"=w932:bool, "Depth Rate"=→"Depth Rate\nft/min":dbl, "Feet of\nStainless to be\nUsed (Count) out"=w922:i32, "Depth Cluster out"=w962:T17, "Single String Pot Session Array out"=w927:dbl[][])  [unwired: 4 in, 1 out]
                "Ik" <- w935
                n438 = Unbundle By Name(w962) -> ("Current Absolute Depth"=w938:dbl)
                n439 = Bundle By Name(cluster=w958, "Feet of Stainless"=w922) -> (w957:T16)
                n440 = local write "Sensor Voltage Cluster"(w956) -> ()
                n441 = local write "Input Depths \nand Parameters Cluster"(w957) -> ()
                n442 = And(x=w933, y=w932) -> ()  [unwired: 1 out]
                n443 = case shown="True" FALSE {
                  tunnel: w927 -> [_ w970]
                  tunnel: [w969 w971] -> w928
                  tunnel: w936 -> [w969 w972]
                  frame False {
                  }
                  frame True {
                    n444 = Build Array (concatenate)(w972, w970) -> (w971:dbl[][])
                  }
                }
                n445 = call "Array to Plot 2016.vi"("Input Cumulative Array"=w928, "Input Real Time Array"=w927) -> ("Cumulative - Depth vs.Drive Rate"=w925:cluster{dbl[], dbl[]}, "Cumulative - Depth vs. Ik"=w951:cluster{dbl[], dbl[]}, "Real Time - Depth vs. Drive Rate"=w926:cluster{dbl[], dbl[]}, "Real Time - Depth vs. Ik"=w940:cluster{dbl[], dbl[]}, "Depth Rate"=w937:dbl)  [unwired: 2 in, 1 out]
                n446 = Bundle By Name(cluster=w953, "Cumulative - Depth vs. Ik"=w951, "Real Time - Depth vs. lk"=w940, "Cumulative - Depth vs. Drive Rate"=w925, "Real Time - Depth vs. Drive Rate"=w926) -> (w952:T19)
                n447 = local write "Depth Rate\nft/min"(w937) -> ()
                n448 = local write "Culmulative Graph Cluster"(w952) -> ()
                n449 = call "write KPRO file.vi"("Corrected Array in"=w927, "Generate Array Calc IK"=w932, "Path in"=w929) -> ()  [unwired: 7 in, 2 out]
                n450 = local write "Large Depth IK Graph Cluster"(w940) -> ()
                n451 = call "write KPRO file.vi"("Corrected Array in"=w928, "Path in"=w918) -> ()  [unwired: 8 in, 2 out]
                n452 = local write "Cumulative_data_from_file"(w928) -> ()
                n453 = local write "Current Session"(w927) -> ()
                n454 = local write "Ik"(w935) -> ()
              }
            }
            n455 = flat-sequence {
              tunnel: w887 -> [w1010]
              tunnel: [w1009] -> w886
              tunnel: w871 -> [w1008]
              tunnel: w870 -> [w1007]
              tunnel: [w1006] -> w869
              tunnel: [w1002] -> w867
              frame #0 {
                n456 = flat-sequence {
                  tunnel: [w1027] -> w1015
                  tunnel: [w1016] -> w1014
                  tunnel: [w1026] -> w1013
                  tunnel: [w1025] -> w1012
                  tunnel: [w1024] -> w1011
                  tunnel: w1010 -> [w1023]
                  tunnel: [w1022] -> w1009
                  tunnel: w1008 -> [w1018]
                  tunnel: [w1016] -> w1002
                  frame #0 {
                    n457 = Unbundle By Name(w1018) -> ("DH Pressure Trans Slope"=w1025:dbl, "DH Pressure Offset"=w1024:dbl)
                    n458 = local write "Input Variables and Slopes"(w1018) -> ()
                    n459 = global read "Kpro Globals.vi" "Current Depth"() -> (w1027:sgl)
                    n460 = local read "Sensor Voltage Cluster"() -> (w1020:T9)
                    n461 = local read "Descriptions"() -> (w1021:string[])
                    n462 = local read "Zero In-Line Pressure\n(F = leave as is)"() -> (w1017:bool)
                    n463 = call "DHT Pressure 2016.vi"("Sensor Cluster"=w1020, "DHT Pressure Offset"=w1024, "Array in"=w1023, "DHT Pressure \nSlope"=w1025, "Descriptions"=w1021, "Zero Pressure\n(F = leave as is)"=w1017) -> ("Array out"=w1022:refnum<k24>[], "DHT Pressure"=w1026:dbl, "Sensor Cluster 2"=w1019:T9)  [unwired: 7 in]
                    n464 = Add(x=w1026, y=w1027) -> (x+y=w1016:dbl)
                    n465 = local write "Sensor Voltage Cluster"(w1019) -> ()
                    n466 = local write "Down hole Pressure"(w1016) -> ()
                  }
                }
                n467 = local read "Record DTW File"() -> (w1005:bool)
                n468 = case shown="True" w1005 {
                  selector: w1005 -> [w1029 _]
                  tunnel: [w1029 FALSE ("Boolean")] -> _
                  tunnel: w1014 -> [_ w1041]
                  tunnel: w1015 -> [_ w1042]
                  tunnel: w1011 -> [_ w1039]
                  tunnel: w1013 -> [_ w1040]
                  tunnel: w1012 -> [_ w1038]
                  tunnel: w1007 -> [w1028 w1033]
                  tunnel: [w1028 w1032] -> w1006
                  frame False {
                  }
                  frame True {
                    n469 = local read "Output File Directory"() -> (w1037:path)
                    n470 = call-poly <userlib>:"Strip Path__ogtk.vi"("path"=w1037) -> ("stripped path"=w1036:path)  [unwired: 1 out]
                    n471 = Build Array(w1042, w1041, w1040, w1039, w1038) -> (w1045:dbl[])
                    n472 = call-poly <userlib>:"Strip Path__ogtk.vi"("path"=path "DTW.csv") -> ("name"=w1034:string)  [unwired: 1 out]
                    n473 = call-poly <userlib>:"Build Path__ogtk.vi"("name or relative path"=w1034, "base path"=w1036) -> ("appended path"=w1030:path)
                    n474 = local write "Down hole Pressure Transducer CSV"(w1030) -> ()
                    n475 = call-poly <vilib>:"Write Delimited Spreadsheet.vi"("file path (dialog if empty)"=w1030, "1D data"=w1045, "append to file? (new file:F)"=TRUE, "error in (no error)"=w1033, "delimiter (\\t)"="," ("delimiter (\\t)")) -> ("error out"=w1032:errorcluster)  [unwired: 9 in, 1 out]
                  }
                }
                n476 = local read "Corrected Pressure Cluster"() -> (w1003:T20)
                n477 = Bundle By Name(cluster=w1003, "Down hole Corrected Pressure"=w1002) -> (w1004:T20)
                n478 = local write "Corrected Pressure Cluster"(w1004) -> ()
              }
            }
            n479 = flat-sequence {
              tunnel: w886 -> [w996]
              tunnel: [w992] -> w885
              tunnel: [w991] -> w884
              frame #0 {
                n480 = local read "Descriptions"() -> (w992:string[])
                n481 = local read "Input Variables and Slopes"() -> (w999:T11)
                n482 = Unbundle By Name(w999) -> ("Up Hole Pressure Slope"=w998:dbl, "Up Hole  Pressure Offset"=w995:dbl)
                n483 = local write "Input Variables and Slopes"(w999) -> ()
                n484 = local read "Sensor Voltage Cluster"() -> (w1000:T9)
                n485 = call "up hole Pressure 2016.vi"("Sensor Cluster"=w1000, "Pressure Offset"=w995, "Array in"=w996, "Pressure \nSlope"=w998, "Descriptions"=w992, "Zero Pressure\n(F = leave as is)"=TRUE) -> ("Array out"=w991:refnum<k24>[], "Uphole Pressure"=w990:dbl, "Sensor Cluster 2"=w997:T9)  [unwired: 6 in, 1 out]
                n486 = local write "Sensor Voltage Cluster"(w997) -> ()
                n487 = local write "Uphole Pressure"(w990) -> ()
                n488 = local read "Corrected Pressure Cluster"() -> (w994:T20)
                n489 = Bundle By Name(cluster=w994, "Up hole Corrected Pressure"=w990) -> (w993:T20)
                n490 = local write "Corrected Pressure Cluster"(w993) -> ()
              }
            }
            n491 = flat-sequence {
              tunnel: w885 -> [w983]
              tunnel: w884 -> [w986]
              tunnel: [w981] -> w881
              tunnel: [w983] -> w883
              tunnel: [w982] -> w878
              tunnel: [w980] -> w876
              frame #0 {
                w987 = 0.0  # Offset
                n492 = local read "Input Depths \nand Parameters Cluster"() -> (w989:T16)
                n493 = local read "Input Variables and Slopes"() -> (w985:T11)
                n494 = Unbundle By Name(w985) -> ("Flow Slope"=w984:dbl)
                n495 = call "Flow 2016.vi"("Descriptions"=w983, "Array in"=w986, "Flow Slope"=w984, "Offset"=w987) -> ("Sensor Cluster"=w981:T9, "Flow (ml/min)"=w982:dbl, "Array out"=w980:refnum<k24>[])  [unwired: 4 in]
                n496 = Bundle By Name(cluster=w989, "Flow"=w982) -> (w988:T16)
                n497 = local write "Input Depths \nand Parameters Cluster"(w988) -> ()
                n498 = local write "Sensor Voltage Cluster"(w981) -> ()
              }
            }
          }
          frame "Sample Not Collected" {
            n499 = local write "Tab Control"(T3."Recording Reason Sonde" ("Tab Control")) -> ()
          }
          frame "Record Sonde Reason" {
            n500 = flat-sequence {
              tunnel: w1064 -> [w1083]
              tunnel: [w1082] -> w1063
              frame #0 {
                n501 = local read "Sonde Recording Error file"() -> (w1081:path)
                n502 = local write "Tab Control"(T3."Recording Reason Sonde" ("Tab Control")) -> ()
                n503 = Get Date/Time In Seconds() -> (seconds since 1Jan1904=w1098:timestamp)
                n504 = Format Date/Time String(seconds (now)=w1098) -> (date/time string=w1095:string)  [unwired: 2 in]
                n505 = local read "Sample Sheet Data Row Cluster 2"() -> (w1099:T2)
                n506 = Unbundle By Name(w1099) -> ("Head\nPressure"=w1097:dbl, "Depth"=w1096:dbl)
                n507 = Format Into String(w1097) -> (resulting string=w1094:string)  [unwired: 3 in, 1 out]
                n508 = Format Into String(w1096) -> (resulting string=w1093:string)  [unwired: 3 in, 1 out]
                n509 = Format Into String("Select Reasons to Record Data") -> (resulting string=w1092:string)  [unwired: 3 in, 1 out]
                n510 = local read "Recording Reason Sonde array"() -> (w1086:string[][])
                n511 = property on="Select Reasons to Record Data" class="Ring (strict)"() -> ("Strings []"=w1091:string[])  [unwired: 2 in, 2 out]
                n512 = Index Array(array=w1091, index="Select Reasons to Record Data") -> (element=w1089:string)
                n513 = Build Array(w1095, w1094, w1093, w1092, w1089) -> (w1084:string[])
                n514 = call-poly <vilib>:"Write Delimited Spreadsheet.vi"("file path (dialog if empty)"=w1081, "1D data"=w1084, "append to file? (new file:F)"=TRUE, "error in (no error)"=w1083, "delimiter (\\t)"="," ("delimiter (\\t)")) -> ("error out"=w1082:errorcluster)  [unwired: 9 in, 1 out]
                n515 = Build Array (concatenate)(w1086, w1084) -> (→"Recording Reason Sonde array":string[][])
              }
            }
          }
          frame "Record IK Reason" {
            n516 = flat-sequence {
              frame #0 {
                n517 = local write "Tab Control"(T3."Pressure/Flow/IK Graphs" ("Tab Control")) -> ()
                n518 = local read "Sonde IK Behavior Path"() -> (w1117:path)
                n519 = Get Date/Time In Seconds() -> (seconds since 1Jan1904=w1132:timestamp)
                n520 = Format Date/Time String(seconds (now)=w1132) -> (date/time string=w1129:string)  [unwired: 2 in]
                n521 = local read "Sample Sheet Data Row Cluster 2"() -> (w1133:T2)
                n522 = Unbundle By Name(w1133) -> ("Head\nPressure"=w1131:dbl, "Depth"=w1130:dbl)
                n523 = Format Into String(w1131) -> (resulting string=w1128:string)  [unwired: 3 in, 1 out]
                n524 = Format Into String(w1130) -> (resulting string=w1127:string)  [unwired: 3 in, 1 out]
                n525 = local read "Select Entry for IK Log File"() -> (w1122:u16)
                n526 = Format Into String(w1122) -> (resulting string=w1126:string)  [unwired: 3 in, 1 out]
                n527 = local read "IK Reason array"() -> (w1118:string[][])
                n528 = property on="Select Entry for IK Log File" class="Ring (strict)"() -> ("Strings []"=w1121:string[])  [unwired: 2 in, 2 out]
                n529 = Index Array(array=w1121, index=w1122) -> (element=w1125:string)
                n530 = Build Array(w1129, w1128, w1127, w1126, w1125) -> (w1124:string[])
                n531 = call-poly <vilib>:"Write Delimited Spreadsheet.vi"("file path (dialog if empty)"=w1117, "1D data"=w1124, "append to file? (new file:F)"=TRUE, "delimiter (\\t)"="," ("delimiter (\\t)")) -> ()  [unwired: 10 in, 2 out]
                n532 = Build Array (concatenate)(w1118, w1124) -> (→"IK Reason array":string[][])
              }
            }
          }
          frame "Continuous  Sonde Data" {
            n533 = control-ref of="Sonde Data Display"() -> (w1159:refnum<vi>)
            n534 = local read "Sample Sheet Data Row Cluster 2"() -> (w1137:T2)
            n535 = Unbundle By Name(w1137) -> ("Sonde Data Cluster.Cumulative\nVolume (ml)"=w1136:dbl)
            n536 = local read "Found Quanta Sonde Com Port"() -> (w1156:refnum<visa-resource-name>)
            n537 = call "SDI-12 Continuous Operations.vi"("RS232 Port In"=w1156, "Sensor Address In"="0", "Sonde Data Ctl Refnum"=w1159, "Error In (No Error)"=w1158) -> ("output cluster"=w1135:T1, "Temperature"=w1154:cluster{"Y":dbl[], "Y":dbl[]}[], "Sonde Data Display"=w1153:T14, "Error Out"=w1157:errorcluster)  [unwired: 8 in, 4 out]
            n538 = local write "Temperature"(w1154) -> ()
            n539 = local write "Sonde Data Display Graphs"(w1153) -> ()
            n540 = Bundle By Name(cluster=w1135, "Cumulative\nVolume (ml)"=w1136) -> (w1134:T1)
            n541 = Bundle By Name(cluster=w1137, "Sonde Data Cluster"=w1134) -> (w1155:T2)
            n542 = local write "Sample Sheet Data Row Cluster 2"(w1155) -> ()
          }
          frame "Acq. Single Sonde Point" {
            n543 = disable-structure shown="Disabled" {
              disable-tunnel: w1193 -> [w1208 _]
              disable-tunnel: w1164 -> [w1207 _]
              disable-tunnel: [w1204 _] -> w1192
              disable-tunnel: [w1203 w1246] -> w1189
              disable-tunnel: [w1202 w1245] -> w1188
              disable-tunnel: [w1201 w1244] -> w1187
              disable-tunnel: w1177 -> [w1200 _]
              disable-tunnel: w1161 -> [w1199 w1244]
              disable-tunnel: w1168 -> [w1194 w1246]
              disable-tunnel: w1166 -> [w1197 _]
              disable-tunnel: w1165 -> [_ w1245]
              frame Disabled {
                n544 = flat-sequence {
                  tunnel: w1197 -> [w1216]
                  tunnel: [w1212] -> w1195
                  tunnel: [w1211] -> w1196
                  tunnel: [w1210] -> w1206
                  tunnel: w1194 -> [w1209]
                  frame #0 {
                    n545 = flat-sequence {
                      tunnel: w1213 -> [w1228]
                      tunnel: [w1221] -> _
                      tunnel: w1214 -> [w1226]
                      tunnel: [w1225] -> w1212
                      tunnel: [w1224] -> _
                      tunnel: [w1223] -> w1210
                      tunnel: w1215 -> [w1221]
                      frame #0 {
                        n546 = local read "Current Sample Sheet"() -> (w1220:string)
                        n547 = call "find last occupied cell.vi"("data"=w1221, "Active Sheet"=w1220, "Header Rows to remove"=3, "sub array start"=w1226, "error in (no error)"=w1228) -> ("row max value"=w1224:i32, "column max value"=w1219:i32, 13:"start of last occupied row"=w1223:cluster{"row":i32, "column":i32}, 14:"start of last occupied row"=w1218:string, "error out"=w1225:errorcluster)  [unwired: 4 in, 2 out]
                        n548 = local write "row max value"(w1219) -> ()
                        n549 = Array Subset(array=w1221, index (col)=2 ("index")) -> (w1217:string[][])  [unwired: 3 in]
                        n550 = local write "subarray"(w1217) -> ()
                        n551 = local write "last occupied cell's name"(w1218) -> ()
                      }
                    }
                    n552 = call "get sample sheet data cells.vi"("error in (no error)"=w1209, "NI_report in"=w1216) -> ("error out"=w1213:errorcluster, "data"=w1215:string[][], "NI_report out"=w1211:refnum<class "NI_report.lvclass">, "left edge output cluster"=w1214:cluster{"row":i32, "column":i32})  [unwired: 5 in, 1 out]
                  }
                }
                n553 = flat-sequence {
                  tunnel: w1198 -> [w1243]
                  tunnel: w1205 -> [w1242]
                  tunnel: [w1241] -> w1204
                  tunnel: [w1236] -> w1203
                  tunnel: [w1234] -> w1202
                  frame #0 {
                    n554 = local read "Current Sample Sheet"() -> (w1232:string)
                    n555 = call <vilib>:"Clear Errors.vi"("error in (no error)"=w1243) -> ("error out"=w1230:errorcluster)  [unwired: 5 in, 1 out]
                    n556 = call "get sample sheet data cells.vi"("error in (no error)"=w1230, "NI_report in"=w1242) -> ("error out"=w1237:errorcluster, "data"=w1238:string[][], "NI_report out"=w1241:refnum<class "NI_report.lvclass">, "left edge output cluster"=w1235:cluster{"row":i32, "column":i32})  [unwired: 5 in, 1 out]
                    n557 = Array Subset(array=w1238, index (col)=2 ("index")) -> (w1229:string[][])  [unwired: 3 in]
                    n558 = local write "subarray"(w1229) -> ()
                    n559 = call "find last occupied cell.vi"("data"=w1238, "Active Sheet"=w1232, "Header Rows to remove"=3, "sub array start"=w1235, "error in (no error)"=w1237) -> ("row max value"=w1233:i32, 13:"start of last occupied row"=w1234:cluster{"row":i32, "column":i32}, 14:"start of last occupied row"=w1231:string, "error out"=w1236:errorcluster)  [unwired: 4 in, 3 out]
                    n560 = local write "row max value"(w1233) -> ()
                    n561 = local write "last occupied cell's name"(w1231) -> ()
                  }
                }
                n562 = call "write out sonde row.vi"("NI_report in"=w1196, "Columns"=w1208, "Column of Volume"=w1207, "Sample Sheet Data Row Cluster"=w1200, "row index"=w1199, "error in (no error)"=w1195, "start of last occupied row"=w1206) -> ("NI_report out"=w1205:refnum<class "NI_report.lvclass">, "row index out"=w1201:i32, "error out"=w1198:errorcluster)  [unwired: 6 in]
              }
              frame Enabled {
              }
            }
            n563 = flat-sequence {
              tunnel: w1167 -> [w1275]
              tunnel: [w1274] -> w1169
              tunnel: w1186 -> [w1273]
              tunnel: [w1272] -> w1185
              tunnel: [w1271] -> w1184
              tunnel: w1183 -> [w1270]
              tunnel: [w1261] -> w1177
              tunnel: [w1269] -> w1174
              tunnel: w1173 -> [w1268]
              frame #0 {
                n564 = local write "Tab Control"(T3."Sonde Data" ("Tab Control")) -> ()
                n565 = local read "Sample Sheet Data Row Cluster 2"() -> (w1260:T2)
                n566 = control-ref of="Found Quanta Sonde Com Port"() -> (w1267:refnum<vi>)
                n567 = control-ref of="Temperature"() -> (w1264:refnum<vi>)
                n568 = control-ref of="Sonde Data Display"() -> (w1266:refnum<vi>)
                n569 = control-ref of="Sonde Data Display Graphs"() -> (w1265:refnum<vi>)
                n570 = control-ref of="Current Time (s)"() -> (w1263:refnum<vi>)
                n571 = call "Sonde Single Measurement Subvi.vi"("VISAResourceName in"=w1267, "Time Array"=w1273, "Cumulative Sonde Data"=w1270, "Previous time"=w1268, "Sonde Data Display"=w1266, "Sonde Graph in"=w1265, "Temp Graph 3"=w1264, "error in (no error)"=w1275, "Row Cluster Input"=w1260, "reference 5"=w1263) -> ("seconds since 1Jan1904"=w1269:timestamp, "Cumulative Sonde \nData Out"=w1271:dbl[][], "Sample Sheet Data Row Cluster 2"=w1261:T2, "output cluster"=→"output cluster":T1, "time array out"=w1272:dbl[], "error out"=w1274:errorcluster)
                n572 = local write "Sample Sheet Data Row Cluster 2"(w1261) -> ()
              }
            }
            n573 = flat-sequence {
              tunnel: w1177 -> [w1258]
              tunnel: w1176 -> [w1255]
              tunnel: w1162 -> [w1248]
              tunnel: [w1252] -> w1171
              tunnel: w1169 -> [w1251]
              tunnel: [w1247] -> w1168
              tunnel: w1163 -> [_]
              tunnel: [w1249] -> w1161
              frame #0 {
                n574 = local read "Sonde Data Array"() -> (w1254:T12[])
                n575 = Increment(x=w1248) -> (x+1=w1249:i32)
                n576 = call "populate sonde row cluster from sonde data cluster.vi"("Initialize \nInitial Value \nCluster"=TRUE ("Initialize \nInitial Value \nCluster"), "error in (no error)"=w1251, "Sonde Parameters \nInitial Values"=w1255, "Sample Sheet Data Row Cluster"=w1258, "Sonde Parameters \nTolerance Limits"="Sonde Parameters \nTolerance Limits") -> ("error out"=w1247:errorcluster, "Cluster"=w1250:T12, "Sonde Parameters \nInitial Values Out"=w1252:T5)  [unwired: 4 in]
                n577 = Insert Into Array(array=w1254, index=w1248, new element=w1250) -> (w1253:T12[])
                n578 = local write "Sonde Data Array"(w1253) -> ()
                n579 = local write "Sonde Parameters \nInitial Values"(w1252) -> ()
              }
            }
            n580 = To Double Precision Float(number=w1174) -> ()  [unwired: 1 out]
            n581 = invoke on="Record Single Sample" class="Bool" method="Reinit To Default"(error in=w1191) -> (error out=w1190:errorcluster)  [unwired: 2 in, 2 out]
            n582 = call <vilib>:"Clear Errors.vi"("error in (no error)"=w1190) -> ("error out"=w1167:errorcluster)  [unwired: 5 in, 1 out]
          }
          frame "pH Calibration Zero" {
            n583 = local read "Found Quanta Sonde Com Port"() -> (w1301:refnum<visa-resource-name>)
            n584 = Equal?(x=w1301, y=refnum<visa-resource-name> refnum ("RS232 Port Out")) -> (x = y?=w1303:bool)
            n585 = invoke on="Record Single Sample" class="Bool" method="Reinit To Default"(error in=w1297) -> (error out=w1296:errorcluster)  [unwired: 2 in, 2 out]
            n586 = call <vilib>:"Clear Errors.vi"("error in (no error)"=w1296) -> ("error out"=w1284:errorcluster)  [unwired: 5 in, 1 out]
            n587 = disable-structure shown="Disabled" {
              disable-tunnel: w1312 -> [w1320 w1332]
              disable-tunnel: [w1316 w1333] -> w1311
              disable-tunnel: [w1315 w1332] -> w1307
              disable-tunnel: [w1314 w1331] -> w1305
              disable-tunnel: w1284 -> [w1313 w1333]
              disable-tunnel: w1276 -> [_ w1331]
              frame Disabled {
                n588 = flat-sequence {
                  tunnel: w1317 -> [w1330]
                  tunnel: [w1324] -> _
                  tunnel: w1318 -> [w1328]
                  tunnel: [w1327] -> w1316
                  tunnel: [w1326] -> _
                  tunnel: [w1325] -> w1314
                  tunnel: w1319 -> [w1324]
                  frame #0 {
                    n589 = local read "Current Sample Sheet"() -> (w1323:string)
                    n590 = call "find last occupied cell.vi"("data"=w1324, "Active Sheet"=w1323, "Header Rows to remove"=3, "sub array start"=w1328, "error in (no error)"=w1330) -> ("row max value"=w1326:i32, "column max value"=w1322:i32, 13:"start of last occupied row"=w1325:cluster{"row":i32, "column":i32}, 14:"start of last occupied row"=w1321:string, "error out"=w1327:errorcluster)  [unwired: 4 in, 2 out]
                    n591 = local write "row max value"(w1322) -> ()
                    n592 = local write "last occupied cell's name"(w1321) -> ()
                  }
                }
                n593 = call "get sample sheet data cells.vi"("error in (no error)"=w1313, "NI_report in"=w1320) -> ("error out"=w1317:errorcluster, "data"=w1319:string[][], "NI_report out"=w1315:refnum<class "NI_report.lvclass">, "left edge output cluster"=w1318:cluster{"row":i32, "column":i32})  [unwired: 5 in, 1 out]
              }
              frame Enabled {
              }
            }
            n594 = case shown="False" w1303 {
              tunnel: w1301 -> [w1359 _]
              tunnel: [w1367 w1390] -> w1304
              tunnel: w1311 -> [w1361 w1393]
              tunnel: [w1370 w1393] -> w1308
              tunnel: w1291 -> [w1366 w1392]
              tunnel: [w1365 w1380] -> w1290
              tunnel: [w1364 w1379] -> w1289
              tunnel: w1288 -> [w1363 w1391]
              tunnel: w1287 -> [_ w1376]
              frame False {
                w1362 = "0" ("Sensor Address In")
                n595 = control-ref of="Sonde Data Display"() -> (w1371:refnum<vi>)
                n596 = call "Calibrate pH Sensor.vi"("Calibration Standard"="pH Zero", "Error In (No Error)"=w1361, "Sensor Address In"=w1362, "RS232 Port In"=w1359) -> ("Error Out"=w1360:errorcluster, "Sensor Calibrate Response"=→"pH Zero \nCalibrate Response":bool, "RS232 Port Out"=w1358:refnum<visa-resource-name>, "Calibration Response String"=→"pH Zero Calibration Response":string)  [unwired: 3 in, 1 out]
                n597 = call "SDI-12 Single Operation with output cluster.vi"("RS232 Port In"=w1358, "Sensor Address In"=w1362, "Sonde Data Ctl Refnum"=w1371, "Error In (No Error)"=w1360, "Time Array In"=w1366, "Measurement Array In"=w1363) -> ("time array out"=w1365:dbl[], "Measurement  array Out"=w1364:dbl[][], "output cluster"=w1369:T1, "Temperature"=w1373:cluster{"Y":dbl[], "Y":dbl[]}[], "Sonde Data Display"=w1372:T14, "Error Out"=w1370:errorcluster)  [unwired: 12 in, 4 out]
                n598 = local write "Temperature"(w1373) -> ()
                n599 = local write "Sonde Data Display Graphs"(w1372) -> ()
                n600 = local read "Sample Sheet Data Row Cluster 2"() -> (w1368:T2)
                n601 = Bundle By Name(cluster=w1368, "Sonde Data Cluster"=w1369) -> (w1367:T2)
              }
              frame True {
                n602 = local read "Sample Sheet Data Row Cluster 2"() -> (w1390:T2)
                n603 = Unbundle By Name(w1390) -> ("Sonde Data Cluster.Temp\ndeg C"=w1375:dbl, "Sonde Data Cluster.pH"=w1389:dbl, "Sonde Data Cluster.Specific\nCond (mS)"=w1388:dbl, "Sonde Data Cluster.Salinity"=w1387:dbl, "Sonde Data Cluster.Dissolved\nOxygen mg/L"=w1386:dbl, "Sonde Data Cluster.ORP"=w1385:dbl)  [unwired: 1 out]
                n604 = Build Array(w1375, w1389, w1388, w1387, w1386, 0.0 ("element"), w1385) -> (w1383:dbl[])
                n605 = Build Array (concatenate)(w1391, w1383) -> (w1379:dbl[][])
                n606 = Get Date/Time In Seconds() -> (seconds since 1Jan1904=w1382:timestamp)
                n607 = To Double Precision Float(number=w1382) -> (double precision float=w1381:dbl)
                n608 = Subtract(x=w1381, y=w1376) -> (x-y=w1374:dbl)
                n609 = Build Array (concatenate)(w1392, w1374) -> (w1380:dbl[])
                n610 = call "format into Sonde Vertical Graph Data Input.vi"("Sonde Measurement Array"=w1379, "Time Array"=w1380) -> ("Sonde Data Display"=w1378:T14, "Temperature"=w1377:cluster{"X":dbl[], "Y":dbl[]}[])  [unwired: 8 in]
                n611 = local write "Temperature"(w1377) -> ()
                n612 = local write "Sonde Data Display Graphs"(w1378) -> ()
                n613 = local write "Current Time (s)"(w1374) -> ()
              }
            }
            n614 = local write "Sample Sheet Data Row Cluster 2"(w1304) -> ()
            n615 = call "write out sonde row.vi"("NI_report in"=w1307, "Columns"=w1310, "Column of Volume"=w1309, "Sample Sheet Data Row Cluster"=w1304, "row index"=w1293, "error in (no error)"=w1308, "start of last occupied row"=w1305) -> ("NI_report out"=w1299:refnum<class "NI_report.lvclass">, "row index out"=w1292:i32, "error out"=w1300:errorcluster)  [unwired: 6 in]
            n616 = disable-structure shown="Enabled" {
              disable-tunnel: w1300 -> [w1338 w1353]
              disable-tunnel: w1299 -> [w1337 w1354]
              disable-tunnel: [w1336 w1354] -> w1298
              disable-tunnel: [w1335 w1353] -> w1295
              disable-tunnel: [w1334 _] -> w1294
              frame Disabled {
                n617 = flat-sequence {
                  tunnel: w1338 -> [w1352]
                  tunnel: w1337 -> [w1351]
                  tunnel: [w1350] -> w1336
                  tunnel: [w1345] -> w1335
                  tunnel: [w1343] -> w1334
                  frame #0 {
                    (unwired) 3 ("Header Rows to remove")
                    n618 = local read "Current Sample Sheet"() -> (w1341:string)
                    n619 = call <vilib>:"Clear Errors.vi"("error in (no error)"=w1352) -> ("error out"=w1339:errorcluster)  [unwired: 5 in, 1 out]
                    n620 = call "get sample sheet data cells.vi"("error in (no error)"=w1339, "NI_report in"=w1351) -> ("error out"=w1346:errorcluster, "data"=w1347:string[][], "NI_report out"=w1350:refnum<class "NI_report.lvclass">, "left edge output cluster"=w1344:cluster{"row":i32, "column":i32})  [unwired: 5 in, 1 out]
                    n621 = Array Subset(array=w1347, index (col)=2 ("index")) -> ()  [unwired: 3 in, 1 out]
                    n622 = call "find last occupied cell.vi"("data"=w1347, "Active Sheet"=w1341, "Header Rows to remove"=3, "sub array start"=w1344, "error in (no error)"=w1346) -> ("row max value"=w1342:i32, 13:"start of last occupied row"=w1343:cluster{"row":i32, "column":i32}, 14:"start of last occupied row"=w1340:string, "error out"=w1345:errorcluster)  [unwired: 4 in, 3 out]
                    n623 = local write "row max value"(w1342) -> ()
                    n624 = local write "last occupied cell's name"(w1340) -> ()
                  }
                }
              }
              frame Enabled {
              }
            }
          }
          frame "pH Calibration Standard" {
            n625 = local read "Found Quanta Sonde Com Port"() -> (w1420:refnum<visa-resource-name>)
            n626 = Equal?(x=w1420, y=refnum<visa-resource-name> refnum ("RS232 Port Out")) -> (x = y?=w1422:bool)
            n627 = invoke on="Record Single Sample" class="Bool" method="Reinit To Default"(error in=w1416) -> (error out=w1415:errorcluster)  [unwired: 2 in, 2 out]
            n628 = call <vilib>:"Clear Errors.vi"("error in (no error)"=w1415) -> ("error out"=w1403:errorcluster)  [unwired: 5 in, 1 out]
            n629 = disable-structure shown="Disabled" {
              disable-tunnel: w1430 -> [w1438 w1451]
              disable-tunnel: [w1434 w1452] -> w1429
              disable-tunnel: [w1433 w1451] -> w1425
              disable-tunnel: [w1432 w1450] -> w1394
              disable-tunnel: w1403 -> [w1431 w1452]
              disable-tunnel: w1395 -> [_ w1450]
              frame Disabled {
                n630 = flat-sequence {
                  tunnel: w1435 -> [w1449]
                  tunnel: [w1442] -> _
                  tunnel: w1436 -> [w1447]
                  tunnel: [w1446] -> w1434
                  tunnel: [w1445] -> _
                  tunnel: [w1444] -> w1432
                  tunnel: w1437 -> [w1442]
                  frame #0 {
                    n631 = local read "Current Sample Sheet"() -> (w1441:string)
                    n632 = call "find last occupied cell.vi"("data"=w1442, "Active Sheet"=w1441, "Header Rows to remove"=3, "sub array start"=w1447, "error in (no error)"=w1449) -> ("row max value"=w1445:i32, "column max value"=w1440:i32, 13:"start of last occupied row"=w1444:cluster{"row":i32, "column":i32}, 14:"start of last occupied row"=w1439:string, "error out"=w1446:errorcluster)  [unwired: 4 in, 2 out]
                    n633 = local write "row max value"(w1440) -> ()
                    n634 = Array Subset(array=w1442, index (col)=2 ("index")) -> ()  [unwired: 3 in, 1 out]
                    n635 = local write "last occupied cell's name"(w1439) -> ()
                  }
                }
                n636 = call "get sample sheet data cells.vi"("error in (no error)"=w1431, "NI_report in"=w1438) -> ("error out"=w1435:errorcluster, "data"=w1437:string[][], "NI_report out"=w1433:refnum<class "NI_report.lvclass">, "left edge output cluster"=w1436:cluster{"row":i32, "column":i32})  [unwired: 5 in, 1 out]
              }
              frame Enabled {
              }
            }
            n637 = case shown="True" w1422 {
              tunnel: w1420 -> [w1476 _]
              tunnel: [w1486 w1510] -> w1423
              tunnel: w1429 -> [w1479 w1513]
              tunnel: [w1489 w1513] -> w1426
              tunnel: w1410 -> [w1485 w1512]
              tunnel: [w1484 w1500] -> w1409
              tunnel: [w1483 w1499] -> w1408
              tunnel: w1407 -> [w1482 w1511]
              tunnel: w1406 -> [_ w1496]
              frame False {
                n638 = control-ref of="Sonde Data Display"() -> (w1490:refnum<vi>)
                n639 = call "Calibrate pH Sensor.vi"("Calibration Standard"="pH Reference", "Error In (No Error)"=w1479, "Sensor Address In"="0", "RS232 Port In"=w1476) -> ("Error Out"=w1478:errorcluster, "Sensor Calibrate Response"=→"pH  Reference\nCalibrate Response":bool, "RS232 Port Out"=w1475:refnum<visa-resource-name>)  [unwired: 3 in, 2 out]
                n640 = call "SDI-12 Single Operation with output cluster.vi"("RS232 Port In"=w1475, "Sensor Address In"="0", "Sonde Data Ctl Refnum"=w1490, "Error In (No Error)"=w1478, "Time Array In"=w1485, "Measurement Array In"=w1482) -> ("time array out"=w1484:dbl[], "Measurement  array Out"=w1483:dbl[][], "output cluster"=w1488:T1, "Temperature"=w1492:cluster{"Y":dbl[], "Y":dbl[]}[], "Sonde Data Display"=w1491:T14, "Error Out"=w1489:errorcluster)  [unwired: 12 in, 4 out]
                n641 = local write "Temperature"(w1492) -> ()
                n642 = local write "Sonde Data Display Graphs"(w1491) -> ()
                n643 = local read "Sample Sheet Data Row Cluster 2"() -> (w1487:T2)
                n644 = Bundle By Name(cluster=w1487, "Sonde Data Cluster"=w1488) -> (w1486:T2)
              }
              frame True {
                n645 = local read "Sample Sheet Data Row Cluster 2"() -> (w1510:T2)
                n646 = Unbundle By Name(w1510) -> ("Sonde Data Cluster.Temp\ndeg C"=w1495:dbl, "Sonde Data Cluster.pH"=w1509:dbl, "Sonde Data Cluster.Specific\nCond (mS)"=w1508:dbl, "Sonde Data Cluster.Salinity"=w1507:dbl, "Sonde Data Cluster.Dissolved\nOxygen mg/L"=w1506:dbl, "Sonde Data Cluster.ORP"=w1505:dbl)  [unwired: 1 out]
                n647 = Build Array(w1495, w1509, w1508, w1507, w1506, 0.0 ("element"), w1505) -> (w1503:dbl[])
                n648 = Build Array (concatenate)(w1511, w1503) -> (w1499:dbl[][])
                n649 = Get Date/Time In Seconds() -> (seconds since 1Jan1904=w1502:timestamp)
                n650 = To Double Precision Float(number=w1502) -> (double precision float=w1501:dbl)
                n651 = Subtract(x=w1501, y=w1496) -> (x-y=w1494:dbl)
                n652 = Build Array (concatenate)(w1512, w1494) -> (w1500:dbl[])
                n653 = call "format into Sonde Vertical Graph Data Input.vi"("Sonde Measurement Array"=w1499, "Time Array"=w1500) -> ("Sonde Data Display"=w1498:T14, "Temperature"=w1497:cluster{"X":dbl[], "Y":dbl[]}[])  [unwired: 8 in]
                n654 = local write "Temperature"(w1497) -> ()
                n655 = local write "Sonde Data Display Graphs"(w1498) -> ()
                n656 = local write "Current Time (s)"(w1494) -> ()
              }
            }
            n657 = local write "Sample Sheet Data Row Cluster 2"(w1423) -> ()
            n658 = call "write out sonde row.vi"("NI_report in"=w1425, "Columns"=w1428, "Column of Volume"=w1427, "Sample Sheet Data Row Cluster"=w1423, "row index"=w1412, "error in (no error)"=w1426, "start of last occupied row"=w1394) -> ("NI_report out"=w1418:refnum<class "NI_report.lvclass">, "row index out"=w1411:i32, "error out"=w1419:errorcluster)  [unwired: 6 in]
            n659 = disable-structure shown="Enabled" {
              disable-tunnel: w1419 -> [w1457 w1473]
              disable-tunnel: w1418 -> [w1456 w1474]
              disable-tunnel: [w1455 w1474] -> w1417
              disable-tunnel: [w1454 w1473] -> w1414
              disable-tunnel: [w1453 w1472] -> w1413
              disable-tunnel: w1394 -> [_ w1472]
              frame Disabled {
                n660 = flat-sequence {
                  tunnel: w1457 -> [w1471]
                  tunnel: w1456 -> [w1470]
                  tunnel: [w1469] -> w1455
                  tunnel: [w1464] -> w1454
                  tunnel: [w1462] -> w1453
                  frame #0 {
                    (unwired) 3 ("Header Rows to remove")
                    n661 = local read "Current Sample Sheet"() -> (w1460:string)
                    n662 = call <vilib>:"Clear Errors.vi"("error in (no error)"=w1471) -> ("error out"=w1458:errorcluster)  [unwired: 5 in, 1 out]
                    n663 = call "get sample sheet data cells.vi"("error in (no error)"=w1458, "NI_report in"=w1470) -> ("error out"=w1465:errorcluster, "data"=w1466:string[][], "NI_report out"=w1469:refnum<class "NI_report.lvclass">, "left edge output cluster"=w1463:cluster{"row":i32, "column":i32})  [unwired: 5 in, 1 out]
                    n664 = Array Subset(array=w1466, index (col)=2 ("index")) -> ()  [unwired: 3 in, 1 out]
                    n665 = call "find last occupied cell.vi"("data"=w1466, "Active Sheet"=w1460, "Header Rows to remove"=3, "sub array start"=w1463, "error in (no error)"=w1465) -> ("row max value"=w1461:i32, 13:"start of last occupied row"=w1462:cluster{"row":i32, "column":i32}, 14:"start of last occupied row"=w1459:string, "error out"=w1464:errorcluster)  [unwired: 4 in, 3 out]
                    n666 = local write "row max value"(w1461) -> ()
                    n667 = local write "last occupied cell's name"(w1459) -> ()
                  }
                }
              }
              frame Enabled {
              }
            }
          }
          frame "ORP Calibration Standard" {
            n668 = local read "Found Quanta Sonde Com Port"() -> (w1540:refnum<visa-resource-name>)
            n669 = Equal?(x=w1540, y=refnum<visa-resource-name> refnum ("RS232 Port Out")) -> (x = y?=w1542:bool)
            n670 = invoke on="Record Single Sample" class="Bool" method="Reinit To Default"(error in=w1536) -> (error out=w1535:errorcluster)  [unwired: 2 in, 2 out]
            n671 = call <vilib>:"Clear Errors.vi"("error in (no error)"=w1535) -> ("error out"=w1525:errorcluster)  [unwired: 5 in, 1 out]
            n672 = disable-structure shown="Disabled" {
              disable-tunnel: w1550 -> [w1558 w1572]
              disable-tunnel: [w1554 w1571] -> w1549
              disable-tunnel: [w1553 w1572] -> w1545
              disable-tunnel: w1525 -> [w1552 w1571]
              disable-tunnel: [w1551 w1570] -> w1515
              disable-tunnel: w1514 -> [_ w1570]
              frame Disabled {
                n673 = flat-sequence {
                  tunnel: w1555 -> [w1569]
                  tunnel: [w1562] -> _
                  tunnel: w1556 -> [w1567]
                  tunnel: [w1566] -> w1554
                  tunnel: [w1565] -> _
                  tunnel: [w1564] -> w1551
                  tunnel: w1557 -> [w1562]
                  frame #0 {
                    n674 = local read "Current Sample Sheet"() -> (w1561:string)
                    n675 = call "find last occupied cell.vi"("data"=w1562, "Active Sheet"=w1561, "Header Rows to remove"=3, "sub array start"=w1567, "error in (no error)"=w1569) -> ("row max value"=w1565:i32, "column max value"=w1560:i32, 13:"start of last occupied row"=w1564:cluster{"row":i32, "column":i32}, 14:"start of last occupied row"=w1559:string, "error out"=w1566:errorcluster)  [unwired: 4 in, 2 out]
                    n676 = local write "row max value"(w1560) -> ()
                    n677 = Array Subset(array=w1562, index (col)=2 ("index")) -> ()  [unwired: 3 in, 1 out]
                    n678 = local write "last occupied cell's name"(w1559) -> ()
                  }
                }
                n679 = call "get sample sheet data cells.vi"("error in (no error)"=w1552, "NI_report in"=w1558) -> ("error out"=w1555:errorcluster, "data"=w1557:string[][], "NI_report out"=w1553:refnum<class "NI_report.lvclass">, "left edge output cluster"=w1556:cluster{"row":i32, "column":i32})  [unwired: 5 in, 1 out]
              }
              frame Enabled {
              }
            }
            n680 = case shown="False" w1542 {
              tunnel: w1540 -> [w1596 _]
              tunnel: [w1606 w1630] -> w1543
              tunnel: w1549 -> [w1598 w1633]
              tunnel: [w1609 w1633] -> w1546
              tunnel: w1530 -> [w1605 w1632]
              tunnel: [w1604 w1620] -> w1529
              tunnel: [w1603 w1619] -> w1518
              tunnel: w1517 -> [w1602 w1631]
              tunnel: w1528 -> [_ w1616]
              frame False {
                n681 = control-ref of="Sonde Data Display"() -> (w1610:refnum<vi>)
                n682 = call "Calibrate ORP Sensor2.vi"("Calibration Standard"="ORP Reference", "Error In (No Error)"=w1598, "Sensor Address In"="0", "RS232 Port In"=w1596) -> ("Error Out"=w1597:errorcluster, "Sensor Calibrate Response"=→"ORP  Reference\nCalibrate Response":bool, "RS232 Port Out"=w1595:refnum<visa-resource-name>)  [unwired: 3 in, 2 out]
                n683 = call "SDI-12 Single Operation with output cluster.vi"("RS232 Port In"=w1595, "Sensor Address In"="0", "Sonde Data Ctl Refnum"=w1610, "Error In (No Error)"=w1597, "Time Array In"=w1605, "Measurement Array In"=w1602) -> ("time array out"=w1604:dbl[], "Measurement  array Out"=w1603:dbl[][], "output cluster"=w1608:T1, "Temperature"=w1612:cluster{"Y":dbl[], "Y":dbl[]}[], "Sonde Data Display"=w1611:T14, "Error Out"=w1609:errorcluster)  [unwired: 12 in, 4 out]
                n684 = local write "Temperature"(w1612) -> ()
                n685 = local write "Sonde Data Display Graphs"(w1611) -> ()
                n686 = local read "Sample Sheet Data Row Cluster 2"() -> (w1607:T2)
                n687 = Bundle By Name(cluster=w1607, "Sonde Data Cluster"=w1608) -> (w1606:T2)
              }
              frame True {
                n688 = local read "Sample Sheet Data Row Cluster 2"() -> (w1630:T2)
                n689 = Unbundle By Name(w1630) -> ("Sonde Data Cluster.Temp\ndeg C"=w1615:dbl, "Sonde Data Cluster.pH"=w1629:dbl, "Sonde Data Cluster.Specific\nCond (mS)"=w1628:dbl, "Sonde Data Cluster.Salinity"=w1627:dbl, "Sonde Data Cluster.Dissolved\nOxygen mg/L"=w1626:dbl, "Sonde Data Cluster.ORP"=w1625:dbl)  [unwired: 1 out]
                n690 = Build Array(w1615, w1629, w1628, w1627, w1626, 0.0 ("element"), w1625) -> (w1623:dbl[])
                n691 = Build Array (concatenate)(w1631, w1623) -> (w1619:dbl[][])
                n692 = Get Date/Time In Seconds() -> (seconds since 1Jan1904=w1622:timestamp)
                n693 = To Double Precision Float(number=w1622) -> (double precision float=w1621:dbl)
                n694 = Subtract(x=w1621, y=w1616) -> (x-y=w1614:dbl)
                n695 = Build Array (concatenate)(w1632, w1614) -> (w1620:dbl[])
                n696 = call "format into Sonde Vertical Graph Data Input.vi"("Sonde Measurement Array"=w1619, "Time Array"=w1620) -> ("Sonde Data Display"=w1618:T14, "Temperature"=w1617:cluster{"X":dbl[], "Y":dbl[]}[])  [unwired: 8 in]
                n697 = local write "Temperature"(w1617) -> ()
                n698 = local write "Sonde Data Display Graphs"(w1618) -> ()
                n699 = local write "Current Time (s)"(w1614) -> ()
              }
            }
            n700 = local write "Sample Sheet Data Row Cluster 2"(w1543) -> ()
            n701 = call "write out sonde row.vi"("NI_report in"=w1545, "Columns"=w1548, "Column of Volume"=w1547, "Sample Sheet Data Row Cluster"=w1543, "row index"=w1532, "error in (no error)"=w1546, "start of last occupied row"=w1515) -> ("NI_report out"=w1538:refnum<class "NI_report.lvclass">, "row index out"=w1531:i32, "error out"=w1539:errorcluster)  [unwired: 6 in]
            n702 = disable-structure shown="Enabled" {
              disable-tunnel: w1539 -> [w1577 w1593]
              disable-tunnel: w1538 -> [w1576 w1594]
              disable-tunnel: [w1575 w1594] -> w1537
              disable-tunnel: [w1574 w1593] -> w1534
              disable-tunnel: [w1573 w1592] -> w1533
              disable-tunnel: w1515 -> [_ w1592]
              frame Disabled {
                n703 = flat-sequence {
                  tunnel: w1577 -> [w1591]
                  tunnel: w1576 -> [w1590]
                  tunnel: [w1589] -> w1575
                  tunnel: [w1584] -> w1574
                  tunnel: [w1582] -> w1573
                  frame #0 {
                    (unwired) 3 ("Header Rows to remove")
                    n704 = local read "Current Sample Sheet"() -> (w1580:string)
                    n705 = call <vilib>:"Clear Errors.vi"("error in (no error)"=w1591) -> ("error out"=w1578:errorcluster)  [unwired: 5 in, 1 out]
                    n706 = call "get sample sheet data cells.vi"("error in (no error)"=w1578, "NI_report in"=w1590) -> ("error out"=w1585:errorcluster, "data"=w1586:string[][], "NI_report out"=w1589:refnum<class "NI_report.lvclass">, "left edge output cluster"=w1583:cluster{"row":i32, "column":i32})  [unwired: 5 in, 1 out]
                    n707 = Array Subset(array=w1586, index (col)=2 ("index")) -> ()  [unwired: 3 in, 1 out]
                    n708 = call "find last occupied cell.vi"("data"=w1586, "Active Sheet"=w1580, "Header Rows to remove"=3, "sub array start"=w1583, "error in (no error)"=w1585) -> ("row max value"=w1581:i32, 13:"start of last occupied row"=w1582:cluster{"row":i32, "column":i32}, 14:"start of last occupied row"=w1579:string, "error out"=w1584:errorcluster)  [unwired: 4 in, 3 out]
                    n709 = local write "row max value"(w1581) -> ()
                    n710 = local write "last occupied cell's name"(w1579) -> ()
                  }
                }
              }
              frame Enabled {
              }
            }
          }
          frame "Salinity Calibration Standard" {
            n711 = local read "Found Quanta Sonde Com Port"() -> (w1660:refnum<visa-resource-name>)
            n712 = Equal?(x=w1660, y=refnum<visa-resource-name> refnum ("RS232 Port Out")) -> (x = y?=w1662:bool)
            n713 = invoke on="Record Single Sample" class="Bool" method="Reinit To Default"(error in=w1656) -> (error out=w1655:errorcluster)  [unwired: 2 in, 2 out]
            n714 = call <vilib>:"Clear Errors.vi"("error in (no error)"=w1655) -> ("error out"=w1643:errorcluster)  [unwired: 5 in, 1 out]
            n715 = disable-structure shown="Enabled" {
              disable-tunnel: w1670 -> [w1678 w1692]
              disable-tunnel: [w1674 w1691] -> w1669
              disable-tunnel: [w1673 w1692] -> w1665
              disable-tunnel: w1643 -> [w1672 w1691]
              disable-tunnel: [w1671 w1690] -> w1635
              disable-tunnel: w1634 -> [_ w1690]
              frame Disabled {
                n716 = flat-sequence {
                  tunnel: w1675 -> [w1689]
                  tunnel: [w1682] -> _
                  tunnel: w1676 -> [w1687]
                  tunnel: [w1686] -> w1674
                  tunnel: [w1685] -> _
                  tunnel: [w1684] -> w1671
                  tunnel: w1677 -> [w1682]
                  frame #0 {
                    n717 = local read "Current Sample Sheet"() -> (w1681:string)
                    n718 = call "find last occupied cell.vi"("data"=w1682, "Active Sheet"=w1681, "Header Rows to remove"=3, "sub array start"=w1687, "error in (no error)"=w1689) -> ("row max value"=w1685:i32, "column max value"=w1680:i32, 13:"start of last occupied row"=w1684:cluster{"row":i32, "column":i32}, 14:"start of last occupied row"=w1679:string, "error out"=w1686:errorcluster)  [unwired: 4 in, 2 out]
                    n719 = local write "row max value"(w1680) -> ()
                    n720 = Array Subset(array=w1682, index (col)=2 ("index")) -> ()  [unwired: 3 in, 1 out]
                    n721 = local write "last occupied cell's name"(w1679) -> ()
                  }
                }
                n722 = call "get sample sheet data cells.vi"("error in (no error)"=w1672, "NI_report in"=w1678) -> ("error out"=w1675:errorcluster, "data"=w1677:string[][], "NI_report out"=w1673:refnum<class "NI_report.lvclass">, "left edge output cluster"=w1676:cluster{"row":i32, "column":i32})  [unwired: 5 in, 1 out]
              }
              frame Enabled {
              }
            }
            n723 = case shown="False" w1662 {
              tunnel: w1660 -> [w1719 _]
              tunnel: [w1726 w1750] -> w1663
              tunnel: w1669 -> [w1717 w1753]
              tunnel: [w1729 w1753] -> w1666
              tunnel: w1650 -> [w1725 w1752]
              tunnel: [w1724 w1740] -> w1649
              tunnel: [w1723 w1739] -> w1648
              tunnel: w1647 -> [w1722 w1751]
              tunnel: w1646 -> [_ w1736]
              frame False {
                n724 = control-ref of="Sonde Data Display"() -> (w1730:refnum<vi>)
                n725 = call "Calibrate Salinity Sensor2.vi"("Calibration Standard"="Salinity \nReference", "Error In (No Error)"=w1717, "Sensor Address In"="0", "RS232 Port In"=w1719) -> ("Error Out"=w1716:errorcluster, "Sensor Calibrate Response"=→"Salinity  Reference\nCalibrate Response":bool, "RS232 Port Out"=w1718:refnum<visa-resource-name>)  [unwired: 3 in, 2 out]
                n726 = call "SDI-12 Single Operation with output cluster.vi"("RS232 Port In"=w1718, "Sensor Address In"="0", "Sonde Data Ctl Refnum"=w1730, "Error In (No Error)"=w1716, "Time Array In"=w1725, "Measurement Array In"=w1722) -> ("time array out"=w1724:dbl[], "Measurement  array Out"=w1723:dbl[][], "output cluster"=w1728:T1, "Temperature"=w1732:cluster{"Y":dbl[], "Y":dbl[]}[], "Sonde Data Display"=w1731:T14, "Error Out"=w1729:errorcluster)  [unwired: 12 in, 4 out]
                n727 = local write "Temperature"(w1732) -> ()
                n728 = local write "Sonde Data Display Graphs"(w1731) -> ()
                n729 = local read "Sample Sheet Data Row Cluster 2"() -> (w1727:T2)
                n730 = Bundle By Name(cluster=w1727, "Sonde Data Cluster"=w1728) -> (w1726:T2)
              }
              frame True {
                n731 = local read "Sample Sheet Data Row Cluster 2"() -> (w1750:T2)
                n732 = Unbundle By Name(w1750) -> ("Sonde Data Cluster.Temp\ndeg C"=w1735:dbl, "Sonde Data Cluster.pH"=w1749:dbl, "Sonde Data Cluster.Specific\nCond (mS)"=w1748:dbl, "Sonde Data Cluster.Salinity"=w1747:dbl, "Sonde Data Cluster.Dissolved\nOxygen mg/L"=w1746:dbl, "Sonde Data Cluster.ORP"=w1745:dbl)  [unwired: 1 out]
                n733 = Build Array(w1735, w1749, w1748, w1747, w1746, 0.0 ("element"), w1745) -> (w1743:dbl[])
                n734 = Build Array (concatenate)(w1751, w1743) -> (w1739:dbl[][])
                n735 = Get Date/Time In Seconds() -> (seconds since 1Jan1904=w1742:timestamp)
                n736 = To Double Precision Float(number=w1742) -> (double precision float=w1741:dbl)
                n737 = Subtract(x=w1741, y=w1736) -> (x-y=w1734:dbl)
                n738 = Build Array (concatenate)(w1752, w1734) -> (w1740:dbl[])
                n739 = call "format into Sonde Vertical Graph Data Input.vi"("Sonde Measurement Array"=w1739, "Time Array"=w1740) -> ("Sonde Data Display"=w1738:T14, "Temperature"=w1737:cluster{"X":dbl[], "Y":dbl[]}[])  [unwired: 8 in]
                n740 = local write "Temperature"(w1737) -> ()
                n741 = local write "Sonde Data Display Graphs"(w1738) -> ()
                n742 = local write "Current Time (s)"(w1734) -> ()
              }
            }
            n743 = local write "Sample Sheet Data Row Cluster 2"(w1663) -> ()
            n744 = call "write out sonde row.vi"("NI_report in"=w1665, "Columns"=w1668, "Column of Volume"=w1667, "Sample Sheet Data Row Cluster"=w1663, "row index"=w1652, "error in (no error)"=w1666, "start of last occupied row"=w1635) -> ("NI_report out"=w1658:refnum<class "NI_report.lvclass">, "row index out"=w1651:i32, "error out"=w1659:errorcluster)  [unwired: 6 in]
            n745 = disable-structure shown="Enabled" {
              disable-tunnel: w1659 -> [w1697 w1713]
              disable-tunnel: w1658 -> [w1696 w1714]
              disable-tunnel: [w1695 w1714] -> w1657
              disable-tunnel: [w1694 w1713] -> w1654
              disable-tunnel: [w1693 w1712] -> w1653
              disable-tunnel: w1635 -> [_ w1712]
              frame Disabled {
                n746 = flat-sequence {
                  tunnel: w1697 -> [w1711]
                  tunnel: w1696 -> [w1710]
                  tunnel: [w1709] -> w1695
                  tunnel: [w1704] -> w1694
                  tunnel: [w1702] -> w1693
                  frame #0 {
                    (unwired) 3 ("Header Rows to remove")
                    n747 = local read "Current Sample Sheet"() -> (w1700:string)
                    n748 = call <vilib>:"Clear Errors.vi"("error in (no error)"=w1711) -> ("error out"=w1698:errorcluster)  [unwired: 5 in, 1 out]
                    n749 = call "get sample sheet data cells.vi"("error in (no error)"=w1698, "NI_report in"=w1710) -> ("error out"=w1705:errorcluster, "data"=w1706:string[][], "NI_report out"=w1709:refnum<class "NI_report.lvclass">, "left edge output cluster"=w1703:cluster{"row":i32, "column":i32})  [unwired: 5 in, 1 out]
                    n750 = Array Subset(array=w1706, index (col)=2 ("index")) -> ()  [unwired: 3 in, 1 out]
                    n751 = call "find last occupied cell.vi"("data"=w1706, "Active Sheet"=w1700, "Header Rows to remove"=3, "sub array start"=w1703, "error in (no error)"=w1705) -> ("row max value"=w1701:i32, 13:"start of last occupied row"=w1702:cluster{"row":i32, "column":i32}, 14:"start of last occupied row"=w1699:string, "error out"=w1704:errorcluster)  [unwired: 4 in, 3 out]
                    n752 = local write "row max value"(w1701) -> ()
                    n753 = local write "last occupied cell's name"(w1699) -> ()
                  }
                }
              }
              frame Enabled {
              }
            }
          }
          frame "DO Calibration Standard" {
            n754 = local read "Found Quanta Sonde Com Port"() -> (w1779:refnum<visa-resource-name>)
            n755 = Equal?(x=w1779, y=refnum<visa-resource-name> refnum ("RS232 Port Out")) -> (x = y?=w1781:bool)
            n756 = invoke on="Record Single Sample" class="Bool" method="Reinit To Default"(error in=w1775) -> (error out=w1774:errorcluster)  [unwired: 2 in, 2 out]
            n757 = call <vilib>:"Clear Errors.vi"("error in (no error)"=w1774) -> ("error out"=w1762:errorcluster)  [unwired: 5 in, 1 out]
            n758 = disable-structure shown="Enabled" {
              disable-tunnel: w1790 -> [w1798 w1812]
              disable-tunnel: [w1794 w1811] -> w1789
              disable-tunnel: [w1793 w1812] -> w1785
              disable-tunnel: [w1792 w1810] -> w1783
              disable-tunnel: w1762 -> [w1791 w1811]
              disable-tunnel: w1754 -> [_ w1810]
              frame Disabled {
                n759 = flat-sequence {
                  tunnel: w1795 -> [w1809]
                  tunnel: [w1802] -> _
                  tunnel: w1796 -> [w1807]
                  tunnel: [w1806] -> w1794
                  tunnel: [w1805] -> _
                  tunnel: [w1804] -> w1792
                  tunnel: w1797 -> [w1802]
                  frame #0 {
                    n760 = local read "Current Sample Sheet"() -> (w1801:string)
                    n761 = call "find last occupied cell.vi"("data"=w1802, "Active Sheet"=w1801, "Header Rows to remove"=3, "sub array start"=w1807, "error in (no error)"=w1809) -> ("row max value"=w1805:i32, "column max value"=w1800:i32, 13:"start of last occupied row"=w1804:cluster{"row":i32, "column":i32}, 14:"start of last occupied row"=w1799:string, "error out"=w1806:errorcluster)  [unwired: 4 in, 2 out]
                    n762 = local write "row max value"(w1800) -> ()
                    n763 = Array Subset(array=w1802, index (col)=2 ("index")) -> ()  [unwired: 3 in, 1 out]
                    n764 = local write "last occupied cell's name"(w1799) -> ()
                  }
                }
                n765 = call "get sample sheet data cells.vi"("error in (no error)"=w1791, "NI_report in"=w1798) -> ("error out"=w1795:errorcluster, "data"=w1797:string[][], "NI_report out"=w1793:refnum<class "NI_report.lvclass">, "left edge output cluster"=w1796:cluster{"row":i32, "column":i32})  [unwired: 5 in, 1 out]
              }
              frame Enabled {
              }
            }
            n766 = case shown="True" w1781 {
              tunnel: w1779 -> [w1837 _]
              tunnel: [w1844 w1868] -> w1782
              tunnel: w1789 -> [w1839 w1871]
              tunnel: [w1847 w1871] -> w1786
              tunnel: w1769 -> [w1843 w1870]
              tunnel: [w1842 w1858] -> w1768
              tunnel: [w1841 w1857] -> w1767
              tunnel: w1766 -> [w1840 w1869]
              tunnel: w1765 -> [_ w1854]
              frame False {
                n767 = control-ref of="Sonde Data Display"() -> (w1848:refnum<vi>)
                n768 = call "Calibrate DO Sensor.vi"("Calibration Standard"="DO \nReference", "Error In (No Error)"=w1839, "Sensor Address In"="0", "RS232 Port In"=w1837) -> ("Error Out"=w1838:errorcluster, "Sensor Calibrate Response"=→"DO  Reference\nCalibrate Response":bool, "RS232 Port Out"=w1836:refnum<visa-resource-name>)  [unwired: 4 in, 1 out]
                n769 = call "SDI-12 Single Operation with output cluster.vi"("RS232 Port In"=w1836, "Sensor Address In"="0", "Sonde Data Ctl Refnum"=w1848, "Error In (No Error)"=w1838, "Time Array In"=w1843, "Measurement Array In"=w1840) -> ("time array out"=w1842:dbl[], "Measurement  array Out"=w1841:dbl[][], "output cluster"=w1846:T1, "Temperature"=w1850:cluster{"Y":dbl[], "Y":dbl[]}[], "Sonde Data Display"=w1849:T14, "Error Out"=w1847:errorcluster)  [unwired: 12 in, 4 out]
                n770 = local write "Temperature"(w1850) -> ()
                n771 = local write "Sonde Data Display Graphs"(w1849) -> ()
                n772 = local read "Sample Sheet Data Row Cluster 2"() -> (w1845:T2)
                n773 = Bundle By Name(cluster=w1845, "Sonde Data Cluster"=w1846) -> (w1844:T2)
              }
              frame True {
                n774 = local read "Sample Sheet Data Row Cluster 2"() -> (w1868:T2)
                n775 = Unbundle By Name(w1868) -> ("Sonde Data Cluster.Temp\ndeg C"=w1853:dbl, "Sonde Data Cluster.pH"=w1867:dbl, "Sonde Data Cluster.Specific\nCond (mS)"=w1866:dbl, "Sonde Data Cluster.Salinity"=w1865:dbl, "Sonde Data Cluster.Dissolved\nOxygen mg/L"=w1864:dbl, "Sonde Data Cluster.ORP"=w1863:dbl)  [unwired: 1 out]
                n776 = Build Array(w1853, w1867, w1866, w1865, w1864, 0.0 ("element"), w1863) -> (w1861:dbl[])
                n777 = Build Array (concatenate)(w1869, w1861) -> (w1857:dbl[][])
                n778 = Get Date/Time In Seconds() -> (seconds since 1Jan1904=w1860:timestamp)
                n779 = To Double Precision Float(number=w1860) -> (double precision float=w1859:dbl)
                n780 = Subtract(x=w1859, y=w1854) -> (x-y=w1852:dbl)
                n781 = Build Array (concatenate)(w1870, w1852) -> (w1858:dbl[])
                n782 = call "format into Sonde Vertical Graph Data Input.vi"("Sonde Measurement Array"=w1857, "Time Array"=w1858) -> ("Sonde Data Display"=w1856:T14, "Temperature"=w1855:cluster{"X":dbl[], "Y":dbl[]}[])  [unwired: 8 in]
                n783 = local write "Temperature"(w1855) -> ()
                n784 = local write "Sonde Data Display Graphs"(w1856) -> ()
                n785 = local write "Current Time (s)"(w1852) -> ()
              }
            }
            n786 = local write "Sample Sheet Data Row Cluster 2"(w1782) -> ()
            n787 = call "write out sonde row.vi"("NI_report in"=w1785, "Columns"=w1788, "Column of Volume"=w1787, "Sample Sheet Data Row Cluster"=w1782, "row index"=w1771, "error in (no error)"=w1786, "start of last occupied row"=w1783) -> ("NI_report out"=w1777:refnum<class "NI_report.lvclass">, "row index out"=w1770:i32, "error out"=w1778:errorcluster)  [unwired: 6 in]
            n788 = disable-structure shown="Enabled" {
              disable-tunnel: w1778 -> [w1817 w1831]
              disable-tunnel: w1777 -> [w1816 w1832]
              disable-tunnel: [w1815 w1832] -> w1776
              disable-tunnel: [w1814 w1831] -> w1773
              disable-tunnel: [w1813 _] -> w1772
              frame Disabled {
                n789 = flat-sequence {
                  tunnel: w1817 -> [w1830]
                  tunnel: w1816 -> [w1829]
                  tunnel: [w1828] -> w1815
                  tunnel: [w1824] -> w1814
                  tunnel: [w1822] -> w1813
                  frame #0 {
                    n790 = local read "Current Sample Sheet"() -> (w1820:string)
                    n791 = call <vilib>:"Clear Errors.vi"("error in (no error)"=w1830) -> ("error out"=w1818:errorcluster)  [unwired: 5 in, 1 out]
                    n792 = call "get sample sheet data cells.vi"("error in (no error)"=w1818, "NI_report in"=w1829) -> ("error out"=w1825:errorcluster, "data"=w1826:string[][], "NI_report out"=w1828:refnum<class "NI_report.lvclass">, "left edge output cluster"=w1823:cluster{"row":i32, "column":i32})  [unwired: 5 in, 1 out]
                    n793 = call "find last occupied cell.vi"("data"=w1826, "Active Sheet"=w1820, "Header Rows to remove"=3, "sub array start"=w1823, "error in (no error)"=w1825) -> ("row max value"=w1821:i32, 13:"start of last occupied row"=w1822:cluster{"row":i32, "column":i32}, 14:"start of last occupied row"=w1819:string, "error out"=w1824:errorcluster)  [unwired: 4 in, 3 out]
                    n794 = local write "row max value"(w1821) -> ()
                    n795 = local write "last occupied cell's name"(w1819) -> ()
                  }
                }
              }
              frame Enabled {
              }
            }
          }
          frame "SC Calibration Standard" {
            n796 = local read "Found Quanta Sonde Com Port"() -> (w1898:refnum<visa-resource-name>)
            n797 = Equal?(x=w1898, y=refnum<visa-resource-name> refnum ("RS232 Port Out")) -> (x = y?=w1900:bool)
            n798 = invoke on="Record Single Sample" class="Bool" method="Reinit To Default"(error in=w1894) -> (error out=w1893:errorcluster)  [unwired: 2 in, 2 out]
            n799 = call <vilib>:"Clear Errors.vi"("error in (no error)"=w1893) -> ("error out"=w1881:errorcluster)  [unwired: 5 in, 1 out]
            n800 = disable-structure shown="Disabled" {
              disable-tunnel: w1908 -> [w1916 w1929]
              disable-tunnel: [w1912 w1928] -> w1907
              disable-tunnel: [w1911 w1929] -> w1903
              disable-tunnel: w1881 -> [w1910 w1928]
              disable-tunnel: [w1909 w1927] -> w1873
              disable-tunnel: w1872 -> [_ w1927]
              frame Disabled {
                n801 = flat-sequence {
                  tunnel: w1913 -> [w1926]
                  tunnel: [w1920] -> _
                  tunnel: w1914 -> [w1924]
                  tunnel: [w1923] -> w1912
                  tunnel: [w1922] -> _
                  tunnel: [w1921] -> w1909
                  tunnel: w1915 -> [w1920]
                  frame #0 {
                    n802 = local read "Current Sample Sheet"() -> (w1919:string)
                    n803 = call "find last occupied cell.vi"("data"=w1920, "Active Sheet"=w1919, "Header Rows to remove"=3, "sub array start"=w1924, "error in (no error)"=w1926) -> ("row max value"=w1922:i32, "column max value"=w1918:i32, 13:"start of last occupied row"=w1921:cluster{"row":i32, "column":i32}, 14:"start of last occupied row"=w1917:string, "error out"=w1923:errorcluster)  [unwired: 4 in, 2 out]
                    n804 = local write "row max value"(w1918) -> ()
                    n805 = local write "last occupied cell's name"(w1917) -> ()
                  }
                }
                n806 = call "get sample sheet data cells.vi"("error in (no error)"=w1910, "NI_report in"=w1916) -> ("error out"=w1913:errorcluster, "data"=w1915:string[][], "NI_report out"=w1911:refnum<class "NI_report.lvclass">, "left edge output cluster"=w1914:cluster{"row":i32, "column":i32})  [unwired: 5 in, 1 out]
              }
              frame Enabled {
              }
            }
            n807 = case shown="False" w1900 {
              tunnel: w1898 -> [w1957 _]
              tunnel: [w1963 w1987] -> w1901
              tunnel: w1907 -> [w1955 w1990]
              tunnel: [w1966 w1990] -> w1904
              tunnel: w1888 -> [w1962 w1989]
              tunnel: [w1961 w1977] -> w1887
              tunnel: [w1960 w1976] -> w1886
              tunnel: w1885 -> [w1959 w1988]
              tunnel: w1884 -> [_ w1973]
              frame False {
                n808 = call "Calibrate SC Sensor2.vi"("Calibration Standard"="SC \nReference", "Error In (No Error)"=w1955, "Sensor Address In"="0", "RS232 Port In"=w1957) -> ("Error Out"=w1954:errorcluster, "Sensor Calibrate Response"=→"SC  Reference\nCalibrate Response":bool, "RS232 Port Out"=w1956:refnum<visa-resource-name>)  [unwired: 3 in, 2 out]
                n809 = call <vilib>:"Clear Errors.vi"("error in (no error)"=w1954) -> ("error out"=w1951:errorcluster)  [unwired: 5 in, 1 out]
                n810 = local read "Sample Sheet Data Row Cluster 2"() -> (w1964:T2)
                n811 = control-ref of="Sonde Data Display"() -> (w1967:refnum<vi>)
                n812 = call "SDI-12 Single Operation with output cluster.vi"("RS232 Port In"=w1956, "Sensor Address In"="0", "Sonde Data Ctl Refnum"=w1967, "Error In (No Error)"=w1951, "Time Array In"=w1962, "Measurement Array In"=w1959) -> ("time array out"=w1961:dbl[], "Measurement  array Out"=w1960:dbl[][], "output cluster"=w1965:T1, "Temperature"=w1969:cluster{"Y":dbl[], "Y":dbl[]}[], "Sonde Data Display"=w1968:T14, "Error Out"=w1966:errorcluster)  [unwired: 12 in, 4 out]
                n813 = Bundle By Name(cluster=w1964, "Sonde Data Cluster"=w1965) -> (w1963:T2)
                n814 = local write "Temperature"(w1969) -> ()
                n815 = local write "Sonde Data Display Graphs"(w1968) -> ()
              }
              frame True {
                n816 = local read "Sample Sheet Data Row Cluster 2"() -> (w1987:T2)
                n817 = Unbundle By Name(w1987) -> ("Sonde Data Cluster.Temp\ndeg C"=w1972:dbl, "Sonde Data Cluster.pH"=w1986:dbl, "Sonde Data Cluster.Specific\nCond (mS)"=w1985:dbl, "Sonde Data Cluster.Salinity"=w1984:dbl, "Sonde Data Cluster.Dissolved\nOxygen mg/L"=w1983:dbl, "Sonde Data Cluster.ORP"=w1982:dbl)  [unwired: 1 out]
                n818 = Build Array(w1972, w1986, w1985, w1984, w1983, 0.0 ("element"), w1982) -> (w1980:dbl[])
                n819 = Build Array (concatenate)(w1988, w1980) -> (w1976:dbl[][])
                n820 = Get Date/Time In Seconds() -> (seconds since 1Jan1904=w1979:timestamp)
                n821 = To Double Precision Float(number=w1979) -> (double precision float=w1978:dbl)
                n822 = Subtract(x=w1978, y=w1973) -> (x-y=w1971:dbl)
                n823 = Build Array (concatenate)(w1989, w1971) -> (w1977:dbl[])
                n824 = call "format into Sonde Vertical Graph Data Input.vi"("Sonde Measurement Array"=w1976, "Time Array"=w1977) -> ("Sonde Data Display"=w1975:T14, "Temperature"=w1974:cluster{"X":dbl[], "Y":dbl[]}[])  [unwired: 8 in]
                n825 = local write "Temperature"(w1974) -> ()
                n826 = local write "Sonde Data Display Graphs"(w1975) -> ()
                n827 = local write "Current Time (s)"(w1971) -> ()
              }
            }
            n828 = local write "Sample Sheet Data Row Cluster 2"(w1901) -> ()
            n829 = call "write out sonde row.vi"("NI_report in"=w1903, "Columns"=w1906, "Column of Volume"=w1905, "Sample Sheet Data Row Cluster"=w1901, "row index"=w1890, "error in (no error)"=w1904, "start of last occupied row"=w1873) -> ("NI_report out"=w1896:refnum<class "NI_report.lvclass">, "row index out"=w1889:i32, "error out"=w1897:errorcluster)  [unwired: 6 in]
            n830 = disable-structure shown="Enabled" {
              disable-tunnel: w1897 -> [w1934 w1950]
              disable-tunnel: w1896 -> [w1933 w1949]
              disable-tunnel: [w1932 w1949] -> w1895
              disable-tunnel: [w1931 w1950] -> w1892
              disable-tunnel: [w1930 w1948] -> w1891
              disable-tunnel: w1873 -> [_ w1948]
              frame Disabled {
                n831 = flat-sequence {
                  tunnel: w1934 -> [w1947]
                  tunnel: w1933 -> [w1946]
                  tunnel: [w1945] -> w1932
                  tunnel: [w1941] -> w1931
                  tunnel: [w1939] -> w1930
                  frame #0 {
                    (unwired) 2 ("index")
                    n832 = local read "Current Sample Sheet"() -> (w1937:string)
                    n833 = call <vilib>:"Clear Errors.vi"("error in (no error)"=w1947) -> ("error out"=w1935:errorcluster)  [unwired: 5 in, 1 out]
                    n834 = call "get sample sheet data cells.vi"("error in (no error)"=w1935, "NI_report in"=w1946) -> ("error out"=w1942:errorcluster, "data"=w1943:string[][], "NI_report out"=w1945:refnum<class "NI_report.lvclass">, "left edge output cluster"=w1940:cluster{"row":i32, "column":i32})  [unwired: 5 in, 1 out]
                    n835 = call "find last occupied cell.vi"("data"=w1943, "Active Sheet"=w1937, "Header Rows to remove"=3, "sub array start"=w1940, "error in (no error)"=w1942) -> ("row max value"=w1938:i32, 13:"start of last occupied row"=w1939:cluster{"row":i32, "column":i32}, 14:"start of last occupied row"=w1936:string, "error out"=w1941:errorcluster)  [unwired: 4 in, 3 out]
                    n836 = local write "row max value"(w1938) -> ()
                    n837 = local write "last occupied cell's name"(w1936) -> ()
                  }
                }
              }
              frame Enabled {
              }
            }
          }
          frame "Write Sonde Sample Sheet" {
            n838 = disable-structure shown="Disabled" {
              disable-tunnel: [w2022 w2039] -> w2015
              disable-tunnel: [w2021 w2037] -> w2008
              disable-tunnel: w2007 -> [w2020 w2038]
              disable-tunnel: w2006 -> [w2019 w2039]
              disable-tunnel: [w2018 w2038] -> w2000
              disable-tunnel: w1991 -> [_ w2037]
              frame Disabled {
                n839 = flat-sequence {
                  tunnel: [w2035] -> w2022
                  tunnel: [w2034] -> w2021
                  tunnel: w2020 -> [w2033]
                  tunnel: w2019 -> [w2032]
                  tunnel: [w2024] -> w2018
                  frame #0 {
                    n840 = local read "Current Sample Sheet"() -> (w2026:string)
                    n841 = call "get sample sheet data cells.vi"("error in (no error)"=w2033, "NI_report in"=w2032) -> ("error out"=w2036:errorcluster, "data"=w2030:string[][], "NI_report out"=w2035:refnum<class "NI_report.lvclass">, "left edge output cluster"=w2028:cluster{"row":i32, "column":i32})  [unwired: 5 in, 1 out]
                    n842 = Array Subset(array=w2030, index (col)=2 ("index")) -> ()  [unwired: 3 in, 1 out]
                    n843 = call "find last occupied cell.vi"("Active Sheet"=w2026, "Header Rows to remove"=3, "sub array start"=w2028, "error in (no error)"=w2036) -> ("row max value"=w2027:i32, 13:"start of last occupied row"=w2034:cluster{"row":i32, "column":i32}, 14:"start of last occupied row"=w2025:string, "error out"=w2024:errorcluster)  [unwired: 5 in, 3 out]
                    n844 = local write "row max value"(w2027) -> ()
                    n845 = local write "last occupied cell's name"(w2025) -> ()
                    n846 = local write "Sonde Data Array"(T25[] [{"Head"=0.0, "Depth"=0.0, "Time"="19:00", "Cumulative\nVolume"=0.0, "Sp. Conductance"={"Value"=0.506, "%"=0.0, "Tol."=TRUE}, "Dissolved Oxygen"={"Value"=35.14, "%"=0.0, "Tol."=TRUE}, "pH"={"Value"=4.81, "%"=0.0, "Tol."=TRUE}, "ORP"={"Value"=390.0, "%"=0.0, "Tol."=TRUE}, "Temperature"={"Value"=23.86, "%"=0.0, "Tol."=TRUE}, "Salinity"={"Value"=0.24, "%"=0.0, "Tol."=TRUE}, "Final Tol."=TRUE, "Final"=FALSE, "Time 2"=""}, {"Head"=0.0, "Depth"=0.0, "Time"="19:00", "Cumulative\nVolume"=0.0, "Sp. Conductance"={"Value"=0.506, "%"=0.0, "Tol."=TRUE}, "Dissolved Oxygen"={"Value"=35.12, "%"=0.0, "Tol."=TRUE}, "pH"={"Value"=4.81, "%"=0.0, "Tol."=TRUE}, "ORP"={"Value"=390.0, "%"=0.0, "Tol."=TRUE}, "Temperature"={"Value"=23.89, "%"=0.0, "Tol."=TRUE}, "Salinity"={"Value"=0.24, "%"=0.0, "Tol."=TRUE}, "Final Tol."=TRUE, "Final"=FALSE, "Time 2"=""}, {"Head"=0.0, "Depth"=0.0, "Time"="19:00", "Cumulative\nVolume"=0.0, "Sp. Conductance"={"Value"=0.506, "%"=0.0, "Tol."=TRUE}, "Dissolved Oxygen"={"Value"=35.14, "%"=0.0, "Tol."=TRUE}, "pH"={"Value"=4.81, "%"=0.0, "Tol."=TRUE}, "ORP"={"Value"=390.0, "%"=0.0, "Tol."=TRUE}, "Temperature"={"Value"=23.86, "%"=0.0, "Tol."=TRUE}, "Salinity"={"Value"=0.24, "%"=0.0, "Tol."=TRUE}, "Final Tol."=TRUE, "Final"=FALSE, "Time 2"=""}, {"Head"=0.0, "Depth"=0.0, "Time"="", "Cumulative\nVolume"=0.0, "Sp. Conductance"={"Value"=0.0, "%"=0.0, "Tol."=FALSE}, "Dissolved Oxygen"={"Value"=0.0, "%"=0.0, "Tol."=FALSE}, "pH"={"Value"=0.0, "%"=0.0, "Tol."=FALSE}, "ORP"={"Value"=0.0, "%"=0.0, "Tol."=FALSE}, "Temperature"={"Value"=0.0, "%"=0.0, "Tol."=FALSE}, "Salinity"={"Value"=0.0, "%"=0.0, "Tol."=FALSE}, "Final Tol."=FALSE, "Final"=FALSE, "Time 2"=""}, {"Head"=0.0, "Depth"=0.0, "Time"="", "Cumulative\nVolume"=0.0, "Sp. Conductance"={"Value"=0.0, "%"=0.0, "Tol."=FALSE}, "Dissolved Oxygen"={"Value"=0.0, "%"=0.0, "Tol."=FALSE}, "pH"={"Value"=0.0, "%"=0.0, "Tol."=FALSE}, "ORP"={"Value"=0.0, "%"=0.0, "Tol."=FALSE}, "Temperature"={"Value"=0.0, "%"=0.0, "Tol."=FALSE}, "Salinity"={"Value"=0.0, "%"=0.0, "Tol."=FALSE}, "Final Tol."=FALSE, "Final"=FALSE, "Time 2"=""}, {"Head"=0.0, "Depth"=0.0, "Time"="", "Cumulative\nVolume"=0.0, "Sp. Conductance"={"Value"=0.0, "%"=0.0, "Tol."=FALSE}, "Dissolved Oxygen"={"Value"=0.0, "%"=0.0, "Tol."=FALSE}, "pH"={"Value"=0.0, "%"=0.0, "Tol."=FALSE}, "ORP"={"Value"=0.0, "%"=0.0, "Tol."=FALSE}, "Temperature"={"Value"=0.0, "%"=0.0, "Tol."=FALSE}, "Salinity"={"Value"=0.0, "%"=0.0, "Tol."=FALSE}, "Final Tol."=FALSE, "Final"=FALSE, "Time 2"=""}, {"Head"=0.0, "Depth"=0.0, "Time"="", "Cumulative\nVolume"=0.0, "Sp. Conductance"={"Value"=0.0, "%"=0.0, "Tol."=FALSE}, "Dissolved Oxygen"={"Value"=0.0, "%"=0.0, "Tol."=FALSE}, "pH"={"Value"=0.0, "%"=0.0, "Tol."=FALSE}, "ORP"={"Value"=0.0, "%"=0.0, "Tol."=FALSE}, "Temperature"={"Value"=0.0, "%"=0.0, "Tol."=FALSE}, "Salinity"={"Value"=0.0, "%"=0.0, "Tol."=FALSE}, "Final Tol."=FALSE, "Final"=FALSE, "Time 2"=""}, {"Head"=0.0, "Depth"=0.0, "Time"="", "Cumulative\nVolume"=0.0, "Sp. Conductance"={"Value"=0.0, "%"=0.0, "Tol."=FALSE}, "Dissolved Oxygen"={"Value"=0.0, "%"=0.0, "Tol."=FALSE}, "pH"={"Value"=0.0, "%"=0.0, "Tol."=FALSE}, "ORP"={"Value"=0.0, "%"=0.0, "Tol."=FALSE}, "Temperature"={"Value"=0.0, "%"=0.0, "Tol."=FALSE}, "Salinity"={"Value"=0.0, "%"=0.0, "Tol."=FALSE}, "Final Tol."=FALSE, "Final"=FALSE, "Time 2"=""}, {"Head"=0.0, "Depth"=0.0, "Time"="", "Cumulative\nVolume"=0.0, "Sp. Conductance"={"Value"=0.0, "%"=0.0, "Tol."=FALSE}, "Dissolved Oxygen"={"Value"=0.0, "%"=0.0, "Tol."=FALSE}, "pH"={"Value"=0.0, "%"=0.0, "Tol."=FALSE}, "ORP"={"Value"=0.0, "%"=0.0, "Tol."=FALSE}, "Temperature"={"Value"=0.0, "%"=0.0, "Tol."=FALSE}, "Salinity"={"Value"=0.0, "%"=0.0, "Tol."=FALSE}, "Final Tol."=FALSE, "Final"=FALSE, "Time 2"=""}] ("Sonde Data Array")) -> ()
                  }
                }
              }
              frame Enabled {
              }
            }
            n847 = flat-sequence {
              tunnel: w1994 -> [w2108]
              frame #0 {
                n848 = local read "Sonde Data Array"() -> (w2111:T12[])
                n849 = Index Array(array=w2111, index=w2108) -> (element=w2113:T12)
                n850 = Bundle By Name(cluster=w2113, "Final"=TRUE) -> (w2109:T12)
                n851 = Replace Array Subset(array=w2111, new element=w2109, index=w2108) -> (w2110:T12[])
                n852 = local write "Sonde Data Array"(w2110) -> ()
              }
            }
            n853 = flat-sequence {
              tunnel: w2017 -> [w2040]
              tunnel: w2016 -> [w2054]
              tunnel: w2014 -> [w2052]
              tunnel: w2013 -> [w2051]
              tunnel: w2012 -> [w2050]
              tunnel: [w2049] -> w2011
              tunnel: w2010 -> [w2048]
              tunnel: w2009 -> [w2047]
              tunnel: w1991 -> [_]
              tunnel: [w2045] -> w2007
              tunnel: [w2044] -> w2006
              tunnel: [w2041] -> w2005
              tunnel: w1994 -> [w2043]
              frame #0 {
                # "uses feedback node so \nfile is only written once"
                n854 = Decrement(x=w2043) -> (x-1=w2042:i32)
                n855 = Not Equal?(x=w2048, y=w2047) -> (x != y?=w2046:bool)
                n856 = invoke on="Update Sonde" class="Bool (strict)" method="Reinit To Default"() -> ()  [unwired: 3 in, 3 out]
                n857 = case shown="False" w2046 {
                  tunnel: w2040 -> [_ _]
                  tunnel: w2054 -> [w2067 w2076]
                  tunnel: [w2067 w2075] -> w2053
                  tunnel: w2040 -> [_ _]
                  tunnel: w2050 -> [w2066 w2074]
                  tunnel: [w2066 w2073] -> w2049
                  tunnel: w2042 -> [w2065 w2072]
                  tunnel: [w2065 w2071] -> w2041
                  frame False {
                  }
                  frame True {
                    n858 = flat-sequence {
                      tunnel: w2076 -> [w2080]
                      tunnel: w2074 -> [w2078]
                      tunnel: w2072 -> [w2077]
                      tunnel: [w2079] -> w2070
                      tunnel: [w2086] -> w2069
                      tunnel: [0] -> w2068
                      tunnel: [w2105] -> w2071
                      tunnel: [w2106] -> w2073
                      tunnel: [w2107] -> w2075
                      tunnel: w2070 -> [w2107]
                      tunnel: w2069 -> [w2106]
                      tunnel: w2068 -> [w2105]
                      frame #0 {
                        n859 = Increment(x=w2078) -> (x+1=w2086:i32)
                        n860 = local read "Sonde Data File"() -> (w2084:path)
                        n861 = call <vilib>:"Check if File or Folder Exists.vi"("error in (no error)"=w2080, "path"=w2084) -> ("error out"=w2082:errorcluster, "file or folder exists?"=w2081:bool, "dup path"=w2083:path)  [unwired: 7 in]
                        n862 = case shown="True" w2081 {
                          tunnel: w2082 -> [w2087 w2099]
                          tunnel: w2083 -> [_ w2098]
                          tunnel: [w2087 w2097] -> w2079
                          tunnel: w2078 -> [_ w2095]
                          tunnel: w2077 -> [_ w2092]
                          frame False {
                          }
                          frame True {
                            n863 = local read "Sonde Data Array"() -> (w2094:T12[])
                            n864 = Index Array(array=w2094, index=w2092) -> (element=w2093:T12)
                            n865 = Bundle By Name(cluster=w2093, "Final"=TRUE) -> (w2091:T12)
                            n866 = Replace Array Subset(array=w2094, new element=w2091, index=w2092) -> (w2088:T12[])
                            n867 = local write "Sonde Data Array"(w2088) -> ()
                            n868 = for {
                              tunnel: w2095 -> [w2104]
                              tunnel: [w2103] -> w2089 mode=indexing
                              tunnel: w2088 -> [w2102] mode=indexing
                              n869 = call "convert sonde cluster to spreadsheet array.vi"("Cluster"=w2102, "Sheet"=w2104) -> ("Sonde Data Array (String)"=w2103:string[])  [unwired: 6 in, 3 out]
                            }
                            n870 = call-poly <vilib>:"Write Delimited Spreadsheet.vi"("file path (dialog if empty)"=w2098, "2D data"=w2089, "append to file? (new file:F)"=TRUE, "error in (no error)"=w2099, "transpose? (no:F)"=FALSE, "delimiter (\\t)"="," ("delimiter (\\t)")) -> ("error out"=w2097:errorcluster)  [unwired: 8 in, 1 out]
                          }
                        }
                      }
                      frame #1 {
                        (unwired) T12 {"Head"=0.0, "Depth"=0.0, "Time"="", "Cumulative\nVolume"=0.0, "Sp. Conductance"={"Value"=0.0, "%"=0.0, "Tol."=FALSE}, "Dissolved Oxygen"={"Value"=0.0, "%"=0.0, "Tol."=FALSE}, "pH"={"Value"=0.0, "%"=0.0, "Tol."=FALSE}, "ORP"={"Value"=0.0, "%"=0.0, "Tol."=FALSE}, "Temperature"={"Value"=0.0, "%"=0.0, "Tol."=FALSE}, "Salinity"={"Value"=0.0, "%"=0.0, "Tol."=FALSE}, "Final Tol."=FALSE, "Final"=FALSE, "Time 2"=timestamp(0 s since 1904-01-01), "Aux 1"=0.0, "Aux 2"=0.0, "Aux 3"=0.0} ("Cluster")
                      }
                    }
                  }
                }
                n871 = disable-structure shown="Enabled" {
                  disable-tunnel: w2053 -> [w2062 w2064]
                  disable-tunnel: w2052 -> [w2061 _]
                  disable-tunnel: w2051 -> [w2060 _]
                  disable-tunnel: w2049 -> [w2059 _]
                  disable-tunnel: [w2057 w2064] -> w2045
                  disable-tunnel: [w2056 w2063] -> w2044
                  disable-tunnel: w2040 -> [w2055 w2063]
                  frame Disabled {
                    n872 = call "open select sample sheet.vi"("Number of Sample Sheets"=w2060, "error in (no error)"=w2062, "Worksheet Names"=w2061, "input 1"=w2059, "NI_report in"=w2055) -> ("error out"=w2057:errorcluster, "Current Sample Sheet"=w2058:string, "NI_report out"=w2056:refnum<class "NI_report.lvclass">)  [unwired: 4 in]
                    n873 = local write "Current Sample Sheet"(w2058) -> ()
                  }
                  frame Enabled {
                  }
                }
              }
            }
          }
          frame "Init" {
            n874 = flat-sequence {
              tunnel: "Read String Pot" -> [_]
              tunnel: [w2558] -> w2123
              tunnel: w2130 -> [w2542]
              tunnel: w2126 -> [w2543]
              frame #0 {
                w2548 = 0.0
                w2549 = TRUE
                # "Initialize Incrementer if using hand incrementer,\nDon't use Debug,\nPut use string pot into shift register first pass to avoid allowing\na change in which method is the source of the depth reading."
                n875 = flat-sequence {
                  tunnel: w2559 -> [w2561]
                  tunnel: [w2560] -> w2558
                  frame #0 {
                    w2562 = 15  # Filter Size
                    # "Functional Global in \nBoxcar Integrator\nInitialize filter array to \ncurrent string pot value"
                    n876 = call "Boxcar filter2016.vi"("Initialize"=TRUE, "Filter Size"=w2562, "Filter Input"=w2561) -> ("Filter Output"=w2560:dbl)
                  }
                }
                n877 = global write "Global_SIM_switch.vi" "enable_kpro_file"("enable_kpro_file") -> ()
                n878 = local read "Sensor Voltage Cluster"() -> (w2550:T9)
                n879 = local read "Input Variables and Slopes"() -> (w2556:T11)
                n880 = Unbundle By Name(w2556) -> ("String Pot Slope"=w2555:dbl, "Up Hole Pressure Slope"=w2551:dbl)  [unwired: 1 out]
                n881 = call "In-Line-Pressure 2016.vi"("Zero Pressure\n(F = leave as is)"=w2549, "In-Line Pressure Slope"=w2551, "Sensor Voltages Cluster"=w2550, "In-Line Pressure Offset"=w2548) -> ("Pressure"=w2552:dbl)  [unwired: 7 in]
                n882 = local read "Sample Sheet Data Row Cluster 2"() -> (w2539:T2)
                n883 = local read "Descriptions"() -> (w2541:string[])
                n884 = call "up hole Pressure 2016.vi"("Sensor Cluster"=w2550, "Pressure Offset"=w2548, "Array in"=w2543, "Pressure \nSlope"=w2551, "Descriptions"=w2541, "Zero Pressure\n(F = leave as is)"=w2549) -> ("Array out"=w2540:refnum<k24>[], "Uphole Pressure"=w2537:dbl)  [unwired: 6 in, 2 out]
                n885 = Bundle By Name(cluster="Corrected Pressure Cluster", "Up hole Corrected Pressure"=w2537, "Down hole Corrected Pressure"=w2552) -> (w2553:T20)
                n886 = Bundle By Name(cluster=w2539, "Head\nPressure"=w2537) -> (w2538:T2)
                n887 = local write "Corrected Pressure Cluster"(w2553) -> ()
                n888 = local write "Sample Sheet Data Row Cluster 2"(w2538) -> ()
                n889 = local read "Sensor Voltage Cluster"() -> (w2557:T9)
                n890 = call "depth read from string pot 2016.vi"("Descriptions"=w2541, "error in (no error)"=w2542, "String Pot \nSlope"=w2555, "Array in"=w2540, "Sensor Cluster In"=w2557) -> ("Depth"=w2559:dbl)  [unwired: 11 in, 3 out]
                n891 = global write "Global_SIM_switch.vi" "Simulate AD6B"("Simulate AD6B") -> ()
                n892 = global write "Global_SIM_switch.vi" "enable_slug_file"("enable_slug_file") -> ()
                n893 = global write "Global_SIM_switch.vi" "enable_IKMGS_file"("enable_IKMGS_file") -> ()
              }
            }
            n894 = flat-sequence {
              tunnel: [w2529] -> w2132
              tunnel: w2133 -> [w2532]
              tunnel: [w2531] -> _
              tunnel: w2124 -> [w2531]
              tunnel: w2120 -> [w2530]
              tunnel: w2117 -> [w2528]
              frame #0 {
                n895 = Bundle By Name(cluster=w2528, "Absolute Depth In"=w2531, "Previous Relative Depth"=w2530, "Current Relative Depth"=w2530, "First Relative Depth"=w2530, "Current Absolute Depth"=w2531, "Last Filed Depth"=0.0, "Current Measurement Time"=w2532, "Previous Measurement Time"=w2532, "First Absolute Depth"=w2531) -> (w2529:T17)
              }
            }
            n896 = flat-sequence {
              tunnel: [w2524] -> w2131
              tunnel: [w2523] -> w2124
              tunnel: w2123 -> [w2521]
              tunnel: [w2521] -> w2120
              frame #0 {
                n897 = local read "Input Depths \nand Parameters Cluster"() -> (w2522:T16)
                n898 = Unbundle By Name(w2522) -> ("Start Depth"=w2525:sgl)
                n899 = Less Or Equal To 0?(x=w2525) -> (x <= 0?=w2527:bool)
                n900 = Negate(x=w2525) -> (-x=w2526:sgl)
                n901 = Select(t=w2525, s=w2527, f=w2526) -> (s? t:f=w2523:sgl)
                n902 = Bundle By Name(cluster=w2522, "Abs Start Depth"=w2523, "Current Depth"=w2521) -> (w2524:T16)
                n903 = local write "Input Depths \nand Parameters Cluster"(w2524) -> ()
              }
            }
            n904 = flat-sequence {
              tunnel: w2137 -> [w2589]
              tunnel: [w2576] -> w2127
              tunnel: [w2575] -> w2126
              frame #0 {
                n905 = flat-sequence {
                  tunnel: [w2595] -> w2575
                  tunnel: w2578 -> [w2593]
                  tunnel: w2576 -> [w2592]
                  frame #0 {
                    n906 = local read "Descriptions"() -> (w2596:string[])
                    n907 = call "Measure DAQ Voltages.vi"("error in (no error)"=w2592, "Descriptions"=w2596, "Array in"=w2593) -> ("Raw Voltages"=w2594:dbl[], "Array out"=w2595:refnum<k24>[], "Sensor Cluster"=w2591:T9)  [unwired: 6 in]
                    n908 = local write "Sensor Voltage Cluster"(w2591) -> ()
                    n909 = local write "Raw Voltages"(w2594) -> ()
                  }
                }
                n910 = call "create DAQ strings.vi"("error in (no error)"=w2589, "MCC USB-DAQ Setup"="MCC USB-DAQ Setup") -> ("error IO"=w2582:errorcluster, "Descriptions"=w2580:string[], "delimited string"=w2583:string, "Array"=w2581:string[], "Voltage Range"=w2588:dbl[])  [unwired: 5 in]
                "delimited string" <- w2583
                "Active Channel Array" <- w2581
                "Voltage Range" <- w2588
                "Descriptions" <- w2580
                n911 = call "Physical Channels to Number of channels.vi"("error in (no error)"=w2582, "Physical Channel in"=w2583) -> ("error out"=w2584:errorcluster, "Number of Channels"=w2586:i32)  [unwired: 7 in, 1 out]
                "Number \nof Channels" <- w2586
                n912 = call "Calculate Rate from Num Channels and Max Rate.vi"("error in (no error)"=w2584, "Channel Data Rate S/s"="Channel \nData Rate S/s", "Number of Channels"=w2586) -> ("error out"=w2579:errorcluster, "Rate"=→"Rate":dbl)  [unwired: 7 in]
                n913 = for {
                  tunnel: w2581 -> [w2602] mode=indexing
                  tunnel: w2588 -> [w2601] mode=indexing
                  tunnel: [w2598] -> w2578 mode=indexing
                  shift-right: [w2599] -> w2577
                  shift-left: w2579 -> [w2597]
                  n914 = Negate(x=w2601) -> (-x=w2600:dbl)
                  n915 = call-poly <vilib>:"ULx Create Virtual Channel.vi"("maximum value"=w2601, "minimum value"=w2600, "physical channels"=w2602, "error in"=w2597) -> ("task out"=w2598:refnum<k24>, "error out"=w2599:errorcluster)  [unwired: 10 in]
                }
                n916 = call "get 9V monitor voltage.vi"("error in (no error)"=w2577, "Descriptions"=w2580, "Array"=w2581, "Array 2"=w2578) -> ("error out"=w2576:errorcluster, "9V Voltage Monitor"=w2574:dbl)  [unwired: 6 in]
                "DAQ Error" <- w2576
                "9V Voltage Monitor" <- w2574
                n917 = Greater Or Equal?(x=w2574, y=8.5) -> (x >= y?=→"DAQ On":bool)
              }
            }
            n918 = flat-sequence {
              tunnel: [w2534] -> w2133
              frame #0 {
                n919 = Tick Count (ms)() -> (millisecond timer value=w2536:u32)
                n920 = Divide(x=w2536, y=u32 1000) -> (x/y=w2534:dbl)
              }
            }
            n921 = local write "Initialization"(-1 ("Initialization")) -> ()
            n922 = flat-sequence {
              tunnel: w2127 -> [w2565]
              tunnel: [w2565] -> w2135
              frame #0 {
                w2566 = T24."Enabled" ("Disabled")
                n923 = property on="Write Data to csv file" class="Bool"("DisabledEnum"=w2566) -> (error out=w2569:errorcluster)  [unwired: 2 in, 1 out]
                n924 = property on="Record Continuous Samples" class="Bool"(error in=w2569, "DisabledEnum"=T24."Disabled and Grayed Out" ("Disabled")) -> (error out=w2568:errorcluster)  [unwired: 1 in, 1 out]
                n925 = property on="Record Single Sample" class="Bool"(error in=w2568, "DisabledEnum"=w2566) -> (error out=w2567:errorcluster)  [unwired: 1 in, 1 out]
                n926 = property on="Sample Not Collected" class="Bool"(error in=w2567, "DisabledEnum"=w2566) -> (error out=w2564:errorcluster)  [unwired: 1 in, 1 out]
                n927 = invoke on="Sonde Data Array" class="Arr (strict)" method="Reinit To Default"(error in=w2564) -> ()  [unwired: 2 in, 3 out]
                "Initialization Finished" <- TRUE
              }
            }
            n928 = local read "Descriptions"() -> (w2115:string[])
            n929 = call <vilib>:"Clear Errors.vi"("error in (no error)"=w2127) -> ("error out"=w2114:errorcluster)  [unwired: 5 in, 1 out]
            n930 = stacked-sequence {
              seq-local: [w2144 _ _ _ _ _ _ _ _ _ _] -> [_ w2173 _ _ _ _ _ _ _ _ _]
              seq-local: [_ w2174 _ _ _ _ _ _ _ _ _] -> [_ _ w2203 _ _ _ _ _ _ _ _]
              seq-local: [_ _ w2199 _ _ _ _ _ _ _ _] -> [_ _ _ _ _ _ _ _ _ _ w2512]
              tunnel: [_ _ w2207 _ _ _ _ _ _ _ _] -> _
              tunnel: [_ _ _ _ _ _ errorcluster {"status"=FALSE, "code"=0, "source"=""} ("error out") _ _ _ _] -> _
              tunnel: w2129 -> [_ _ _ _ _ _ _ _ _ _ w2516]
              tunnel: [_ _ _ _ _ _ _ _ _ _ w2515] -> w2128
              tunnel: w2114 -> [w2146 _ _ _ _ _ _ _ _ _ _]
              tunnel: w2126 -> [_ _ w2205 w2390 w2418 w2444 _ _ _ w2483 _]
              tunnel: w2115 -> [_ _ w2204 w2391 w2417 w2443 _ _ _ w2481 _]
              tunnel: [_ _ _ w2392 _ _ _ _ _ _ _] -> _
              tunnel: [_ _ _ _ _ _ _ _ _ _ w2512] -> w2130
              tunnel: w2118 -> [_ _ w2202 _ _ _ _ _ _ _ _]
              tunnel: [_ _ w2201 _ _ _ _ _ _ _ _] -> w2117
              frame #0 {
                n931 = flat-sequence {
                  tunnel: [w2151] -> w2144
                  tunnel: w2146 -> [w2152]
                  frame #0 {
                    n932 = local read "Groundwater Header"() -> (w2158:T10)
                    n933 = Unbundle By Name(w2158) -> ("Kpro box Serial"=w2148:string)
                    n934 = Equal?(x=w2148, y="") -> (x = y?=w2149:bool)
                    n935 = Scan From String(format string="%d", input string=w2148, error in=w2152, default 1=800.0 ("default value 1")) -> (error out=w2153:errorcluster, output 1=w2157:dbl)  [unwired: 1 in, 2 out]
                    n936 = case shown="True" w2149 {
                      tunnel: "KPRO Box Number\n\nEnter the number of the KPRO box you are using." ("prompt") -> [_ w2172]
                      tunnel: w2158 -> [w2162 w2171]
                      tunnel: w2157 -> [w2160 w2170]
                      tunnel: [w2160 w2169] -> w2156
                      tunnel: [w2162 w2167] -> w2154
                      tunnel: w2153 -> [w2161 w2165]
                      tunnel: [w2161 w2164] -> w2151
                      frame False {
                      }
                      frame True {
                        n937 = call <vilib>:"Clear Errors.vi"("error in (no error)"=w2165) -> ("error out"=w2163:errorcluster)  [unwired: 5 in, 1 out]
                        n938 = call "prompt_and_enter_value2.vi"("prompt_IN"=w2172, "Enter value"=w2170) -> ("Numeric"=w2169:dbl)  [unwired: 9 in]
                        n939 = Format Into String(format string="%d", error in=w2163, w2169) -> (resulting string=w2166:string, error out=w2164:errorcluster)  [unwired: 1 in]
                        n940 = Bundle By Name(cluster=w2171, "Kpro box Serial"=w2166) -> (w2167:T10)
                      }
                    }
                    n941 = local write "Groundwater Header"(w2154) -> ()
                    n942 = global write "Kpro Globals.vi" "KPRO Box Number"(w2156) -> ()
                  }
                }
                "Initialization" <- 0
              }
              frame #1 {
                n943 = local write "Initialization"(1 ("Initialization")) -> ()
                n944 = flat-sequence {
                  tunnel: w2173 -> [w2184]
                  tunnel: [w2184] -> w2174
                  frame #0 {
                    n945 = local read "Groundwater Header"() -> (w2189:T10)
                    n946 = Unbundle By Name(w2189) -> ("Profile ID"=w2188:string)
                    n947 = Equal?(x=w2188, y="") -> ()  [unwired: 1 out]
                    n948 = local read "Temporary csv Data Files Directory"() -> (w2185:path)
                    n949 = Path To String(path=w2185) -> (string=w2179:string)
                    n950 = case shown="True" TRUE {
                      tunnel: "Profile ID\n\nEnter the profile ID" ("prompt") -> [_ w2198]
                      tunnel: [w2195 w2197] -> w2177
                      tunnel: w2188 -> [w2195 w2196]
                      frame False {
                      }
                      frame True {
                        n951 = call "prompt_string.vi"("prompt_IN"=w2198, "Enter value"=w2196) -> ("String"=w2197:string)  [unwired: 9 in]
                        n952 = global write "Kpro Globals.vi" "Profile ID"(w2197) -> ()
                      }
                    }
                    n953 = Bundle By Name(cluster=w2189, "Profile ID"=w2177) -> (w2190:T10)
                    n954 = local write "Groundwater Header"(w2190) -> ()
                    n955 = Concatenate Strings(w2179, "\\" ("string"), w2177) -> (w2178:string)
                    n956 = String To Path(string=w2178) -> (path=w2180:path)
                    n957 = call <vilib>:"Check if File or Folder Exists.vi"("error in (no error)"=w2184, "path"=w2180) -> ("error out"=w2183:errorcluster, "file or folder exists?"=w2182:bool, "dup path"=w2181:path)  [unwired: 7 in]
                    n958 = case shown="False" w2182 {
                      tunnel: w2183 -> [w2194 _]
                      tunnel: w2181 -> [w2193 _]
                      frame False {
                        n959 = call <userlib>:"Create Dir if Non-Existant__ogtk.vi"("error in (no error)"=w2194, "Directory Path"=w2193) -> ("dup Directory Path"=w2192:path)  [unwired: 7 in, 2 out]
                        n960 = local write "Output File Directory"(w2192) -> ()
                      }
                      frame True {
                      }
                    }
                  }
                }
              }
              frame #2 {
                n961 = flat-sequence {
                  tunnel: [w2340] -> w2207
                  tunnel: w2203 -> [w2346]
                  tunnel: w2205 -> [w2344]
                  tunnel: w2204 -> [w2343]
                  tunnel: [w2319] -> w2200
                  tunnel: w2202 -> [w2323]
                  tunnel: [w2322] -> w2201
                  frame #0 {
                    n962 = call <vilib>:"Clear Errors.vi"("error in (no error)"=w2346) -> ("error out"=w2324:errorcluster)  [unwired: 5 in, 1 out]
                    n963 = local read "Input Variables and Slopes"() -> (w2350:T11)
                    n964 = Unbundle By Name(w2350) -> ("Up Hole Pressure Slope"=w2353:dbl, "String Pot Slope"=w2352:dbl, "Flow Slope"=w2351:dbl, "DH Pressure Trans Slope"=w2316:dbl, "Aux 1 Slope"=w2315:dbl, "Aux 2 Slope"=w2314:dbl, "Aux 3 Slope"=w2313:dbl, "DH Pressure Offset"=w2304:dbl)
                    n965 = local read "Temporary csv Data Files Directory"() -> (w2345:path)
                    n966 = call "FILE_DIALOG 2016.vi"("flow_slope_IN"=w2351, "pressure_slope_IN"=w2353, "DHT_Pressure_In"=w2316, "string_pot_slope_IN"=w2352, "Descriptions"=w2343, "DHT_Pressure_In Offset"=w2304, "error in (no error)"=w2324, "start path"=w2345, "Aux1_In"=w2315, "Array in"=w2344, "Aux2_In"=w2314, "Aux3_In"=w2313) -> ("path"=w2333:path, "exists"=w2342:bool, "flow_slope_OUT"=w2348:dbl, "pressure_slope_OUT"=w2347:dbl, "Record Output Slopes to  Record File"=w2320:path, "string_pot_slope_OUT"=w2349:dbl, "Record Output Slopes for slopes.csv File"=w2321:path, "error out"=w2339:errorcluster)  [unwired: 6 in, 2 out]
                    n967 = Bundle By Name(cluster=w2350, "String Pot Slope"=w2349, "Flow Slope"=w2348, "Up Hole Pressure Slope"=w2347) -> (w2341:T11)
                    n968 = call-poly <userlib>:"Strip Path Extension__ogtk.vi"("path"=w2333) -> ("root"=w2334:string, "extension"=w2332:string)
                    n969 = String Length(string=w2332) -> (length=w2331:i32)
                    n970 = Equal To 0?(x=w2331) -> (x = 0?=w2330:bool)
                    n971 = Path To String(path=w2333) -> (string=w2335:string)
                    n972 = Match Pattern(string=w2335, regular expression="_KPRO.csv") -> (offset past match=w2337:i32)  [unwired: 1 in, 3 out]
                    n973 = Equal?(x=w2337, y=-1) -> (x = y?=w2329:bool)
                    n974 = Or(x=w2329, y=w2330) -> (x .or. y?=w2328:bool)
                    n975 = global write "Kpro Globals.vi" "Flow Slope"(w2348) -> ()
                    n976 = global write "Kpro Globals.vi" "Pressure \nSlope"(w2347) -> ()
                    n977 = call <vilib>:"Clear Errors.vi"("error in (no error)"=w2339) -> ("error out"=w2312:errorcluster)  [unwired: 5 in, 1 out]
                    n978 = local write "Slopes History File Path"(w2320) -> ()
                    n979 = global write "Kpro Globals.vi" "String Pot \nSlope"(w2349) -> ()
                    n980 = local write "Slopes File Path"(w2321) -> ()
                    n981 = local write "Input Variables and Slopes"(w2341) -> ()
                    n982 = case shown="False" w2328 {
                      tunnel: w2334 -> [_ w2355]
                      tunnel: w2333 -> [w2354 _]
                      tunnel: [w2354 w2356] -> w2307
                      frame False {
                      }
                      frame True {
                        n983 = String To Path(string=w2355) -> (path=w2356:path)
                      }
                    }
                    "Output File Directory" <- w2307
                    n984 = call "append filename to Cascade csv data file.vi"("new ending (none)"="", "Output File Path"=w2307) -> ("Path"=→"appended path":path)  [unwired: 9 in]
                    n985 = call "append filename to Cascade csv data file.vi"("new ending (none)"="_GroundwaterLog.xlsx", "Output File Path"=w2307) -> ("Path"=w2308:path)  [unwired: 9 in]
                    n986 = call "append filename to Cascade csv data file.vi"("new ending (none)"="_KPRO_Session.csv", "Output File Path"=w2307) -> ("Path"=→"KPRO Session Output File Path":path)  [unwired: 9 in]
                    n987 = local write "Excel report file path"(w2308) -> ()
                    n988 = call "append filename to Cascade csv data file.vi"("new ending (none)"="_KPRO.csv", "Output File Path"=w2307) -> ("Path"=w2305:path)  [unwired: 9 in]
                    "KPRO Cumulative Output File Path" <- w2305
                    n989 = call <vilib>:"Check if File or Folder Exists.vi"("path"=w2305) -> ("file or folder exists?"=w2325:bool, "dup path"=w2327:path)  [unwired: 8 in, 1 out]
                    n990 = And(x=w2325, y=w2342) -> (x .and. y?=w2326:bool)
                    n991 = case shown="True" w2326 {
                      selector: w2326 -> [_ w2363]
                      tunnel: w2327 -> [_ w2374]
                      tunnel: w2341 -> [w2359 w2369]
                      tunnel: [w2359 w2368] -> w2340
                      tunnel: w2312 -> [w2358 w2364]
                      tunnel: [w2358 w2364] -> w2319
                      tunnel: w2323 -> [w2357 w2362]
                      tunnel: [w2357 w2361] -> w2322
                      frame False {
                      }
                      frame True {
                        n992 = local read "Culmulative Graph Cluster"() -> (w2373:T19)
                        n993 = call "Get_KPRO_data_from_file 2016.vi"("Output File KPRO Test"=w2374) -> ("Last_height_of_box"=w2366:dbl, "Last_depth_to_water"=w2367:dbl, "Last_depth"=w2365:dbl, "Output_array"=w2360:sgl[][])  [unwired: 7 in]
                        "Cumulative_data_from_file" <- w2360
                        n994 = Bundle By Name(cluster=w2362, "Absolute Depth In"=w2365, "Current Absolute Depth"=w2365) -> (w2361:T17)
                        n995 = Bundle By Name(cluster=w2369, "Depth to Water Table"=w2367, "Height of Sample Box"=w2366) -> (w2368:T11)
                        n996 = call "Array to Plot 2016.vi"("Input Cumulative Array"=w2360) -> ("Cumulative - Depth vs.Drive Rate"=w2370:cluster{dbl[], dbl[]}, "Cumulative - Depth vs. Ik"=w2371:cluster{dbl[], dbl[]})  [unwired: 3 in, 4 out]
                        n997 = Bundle By Name(cluster=w2373, "Cumulative - Depth vs. Ik"=w2371, "Cumulative - Depth vs. Drive Rate"=w2370) -> (w2372:T19)
                        n998 = local write "Culmulative Graph Cluster"(w2372) -> ()
                        n999 = local write "Input Variables and Slopes"(w2368) -> ()
                        "Cumulative_data_ready" <- w2363
                      }
                    }
                  }
                }
                n1000 = local write "Initialization"(2 ("Initialization")) -> ()
                n1001 = flat-sequence {
                  tunnel: [w2284] -> _
                  tunnel: w2200 -> [w2283]
                  frame #0 {
                    n1002 = call <vilib>:"Clear Errors.vi"("error in (no error)"=w2283) -> ("error out"=w2279:errorcluster)  [unwired: 5 in, 1 out]
                    n1003 = call <vilib>:"Check if File or Folder Exists.vi"("error in (no error)"=w2279, "path"="Slopes File Path") -> ("error out"=w2282:errorcluster, "file or folder exists?"=w2280:bool, "dup path"=w2286:path)  [unwired: 7 in]
                    n1004 = case shown="True" w2280 {
                      tunnel: w2286 -> [_ w2303]
                      tunnel: "Input Variables and Slopes" -> [w2290 w2302]
                      tunnel: [w2290 w2301] -> w2285
                      tunnel: w2282 -> [w2289 w2297]
                      tunnel: [w2289 w2297] -> w2284
                      tunnel: [_ w2293] -> _
                      frame False {
                        n1005 = local write "Data Setup Indicator"("Slope file not found." ("Data Setup Indicator")) -> ()
                      }
                      frame True {
                        n1006 = call "Get_SLOPE_data_from_file 2016.vi"("Slopes File Path"=w2303) -> ("Last Aux 1 Slope"=w2296:dbl, "Output_array"=w2293:sgl[][], "Last_String_Pot_Slope"=w2300:dbl, "DHT Offset"=w2291:dbl, "DHT Slope"=w2292:dbl, "Last_Flow_Slope"=w2299:dbl, "Last Aux 2 Slope"=w2295:dbl, "Last Aux 3 Slope"=w2294:dbl, "Last_Pressure_Slope"=w2298:dbl)  [unwired: 6 in]
                        n1007 = Bundle By Name(cluster=w2302, "String Pot Slope"=w2300, "Flow Slope"=w2299, "Up Hole Pressure Slope"=w2298, "Aux 1 Slope"=w2296, "Aux 2 Slope"=w2295, "Aux 3 Slope"=w2294, "DH Pressure Trans Slope"=w2292, "DH Pressure Offset"=w2291) -> (w2301:T11)
                      }
                    }
                    n1008 = local write "Input Variables and Slopes"(w2285) -> ()
                  }
                }
                n1009 = stacked-sequence {
                  seq-local: [_ _ _ _ _ _ w2230 _ _ _] -> [_ _ _ _ _ _ _ _ w2259 _]
                  seq-local: [_ _ _ _ _ _ _ _ w2258 _] -> [_ _ _ _ _ _ _ _ _ w2269]
                  tunnel: w2200 -> [_ _ _ _ _ _ w2227 w2245 _ _]
                  tunnel: [_ _ _ _ _ _ _ _ _ w2271] -> w2199
                  frame #0 {
                    n1010 = local read "Output File Directory"() -> (w2210:path)
                    n1011 = call "append filename to Cascade csv data file.vi"("new ending (none)"="_Sample failure.csv", "Output File Path"=w2210) -> ("Path"=→"Sonde Recording Failure Path" →"Sonde Recording Error file":path)  [unwired: 9 in]
                  }
                  frame #1 {
                    n1012 = local read "Output File Directory"() -> (w2213:path)
                    n1013 = call "append filename to Cascade csv data file.vi"("new ending (none)"="_SondeData.csv", "Output File Path"=w2213) -> ("Path"=→"Sonde Data File":path)  [unwired: 9 in]
                  }
                  frame #2 {
                    n1014 = local read "Output File Directory"() -> (w2216:path)
                    n1015 = call "append filename to Cascade csv data file.vi"("new ending (none)"="_DHTData.csv", "Output File Path"=w2216) -> ("Path"=w2214:path)  [unwired: 9 in]
                    n1016 = local write "Down hole Pressure Transducer CSV"(w2214) -> ()
                  }
                  frame #3 {
                    n1017 = local read "Output File Directory"() -> (w2219:path)
                    n1018 = call "append filename to Cascade csv data file.vi"("new ending (none)"="_IK Behavior.csv", "Output File Path"=w2219) -> ("Path"=→"Sonde IK Behavior Path" →"IK Recording Error file":path)  [unwired: 9 in]
                  }
                  frame #4 {
                    n1019 = local read "Output File Directory"() -> (w2221:path)
                    n1020 = call "append filename to Cascade csv data file.vi"("new ending (none)"="_Static IK.csv", "Output File Path"=w2221) -> ("Path"=→"Static IK path":path)  [unwired: 9 in]
                  }
                  frame #5 {
                    n1021 = local read "Output File Directory"() -> (w2224:path)
                    n1022 = call "append filename to Cascade csv data file.vi"("new ending (none)"="_DHT.csv", "Output File Path"=w2224) -> ("Path"=→"Down hole Pressure Transducer CSV":path)  [unwired: 9 in]
                  }
                  frame #6 {
                    n1023 = local read "Static IK path"() -> (w2231:path)
                    n1024 = call <vilib>:"Check if File or Folder Exists.vi"("error in (no error)"=w2227, "path"=w2231) -> ("error out"=w2226:errorcluster, "file or folder exists?"=w2228:bool, "dup path"=w2229:path)  [unwired: 7 in]
                    n1025 = case shown="True" w2228 {
                      tunnel: w2226 -> [w2234 w2242]
                      tunnel: w2229 -> [w2233 _]
                      tunnel: [w2232 w2242] -> w2230
                      frame False {
                        n1026 = Build Array("Profile ID   " ("string"), "Depth    " ("string"), "Flow " ("string"), "Ik    " ("string")) -> (w2240:string[])
                        n1027 = call-poly <vilib>:"Write Delimited Spreadsheet.vi"("file path (dialog if empty)"=w2233, "1D data"=w2240, "append to file? (new file:F)"=FALSE, "error in (no error)"=w2234, "delimiter (\\t)"="," ("delimiter (\\t)")) -> ("error out"=w2232:errorcluster)  [unwired: 9 in, 1 out]
                      }
                      frame True {
                      }
                    }
                  }
                  frame #7 {
                    n1028 = local read "Sonde Data File"() -> (w2247:path)
                    n1029 = call <vilib>:"Check if File or Folder Exists.vi"("error in (no error)"=w2245, "path"=w2247) -> ("error out"=w2244:errorcluster, "file or folder exists?"=w2243:bool, "dup path"=w2246:path)  [unwired: 7 in]
                    n1030 = case shown="False" w2243 {
                      tunnel: w2244 -> [w2252 w2255]
                      tunnel: w2246 -> [w2251 _]
                      tunnel: [w2250 w2255] -> _
                      frame False {
                        n1031 = call "convert sonde cluster to spreadsheet array.vi"() -> ("sonde labels"=w2249:string[])  [unwired: 8 in, 3 out]
                        n1032 = call-poly <vilib>:"Write Delimited Spreadsheet.vi"("file path (dialog if empty)"=w2251, "1D data"=w2249, "append to file? (new file:F)"=FALSE, "error in (no error)"=w2252, "transpose? (no:F)"=FALSE, "delimiter (\\t)"="," ("delimiter (\\t)")) -> ("error out"=w2250:errorcluster)  [unwired: 8 in, 1 out]
                      }
                      frame True {
                      }
                    }
                  }
                  frame #8 {
                    n1033 = local read "KPRO Session Output File Path"() -> (w2257:path)
                    n1034 = call <vilib>:"Check if File or Folder Exists.vi"("path"=w2257) -> ("file or folder exists?"=w2256:bool)  [unwired: 8 in, 2 out]
                    n1035 = case shown="False" w2256 {
                      tunnel: w2257 -> [w2263 _]
                      tunnel: w2259 -> [w2262 w2266]
                      tunnel: [w2260 w2266] -> w2258
                      frame False {
                        n1036 = local read "KPRO test report header"() -> (w2261:string[])
                        n1037 = call-poly <vilib>:"Write Delimited Spreadsheet.vi"("file path (dialog if empty)"=w2263, "1D data"=w2261, "append to file? (new file:F)"=FALSE, "error in (no error)"=w2262, "delimiter (\\t)"="," ("delimiter (\\t)")) -> ("error out"=w2260:errorcluster)  [unwired: 9 in, 1 out]
                      }
                      frame True {
                      }
                    }
                  }
                  frame #9 {
                    n1038 = local read "KPRO Cumulative Output File Path"() -> (w2270:path)
                    n1039 = call <vilib>:"Check if File or Folder Exists.vi"("path"=w2270) -> ("file or folder exists?"=w2267:bool, "dup path"=w2268:path)  [unwired: 8 in, 1 out]
                    n1040 = case shown="True" w2267 {
                      tunnel: [w2275 w2278] -> w2271
                      tunnel: w2268 -> [w2274 _]
                      tunnel: w2269 -> [w2272 w2278]
                      frame False {
                        n1041 = local read "KPRO test report header"() -> (w2273:string[])
                        n1042 = call-poly <vilib>:"Write Delimited Spreadsheet.vi"("file path (dialog if empty)"=w2274, "1D data"=w2273, "append to file? (new file:F)"=FALSE, "error in (no error)"=w2272, "delimiter (\\t)"="," ("delimiter (\\t)")) -> ("error out"=w2275:errorcluster)  [unwired: 9 in, 1 out]
                      }
                      frame True {
                      }
                    }
                  }
                }
              }
              frame #3 {
                # "Take offset and put\n into Pressure VI."
                n1043 = local write "Initialization"(3 ("Initialization")) -> ()
                n1044 = local read "Input Variables and Slopes"() -> (w2380:T11)
                n1045 = local read "Corrected Pressure Cluster"() -> (w2396:T20)
                n1046 = local read "Groundwater Header"() -> (w2382:T10)
                n1047 = Unbundle By Name(w2382) -> ("Atmospheric Pressure"=w2379:string)
                n1048 = Equal?(x=w2379, y="") -> ()  [unwired: 1 out]
                n1049 = global read "Kpro Globals.vi" "Pressure Offset"() -> (w2375:dbl)
                n1050 = case shown="False" TRUE {
                  tunnel: "ATMOSPHERIC PRESSURE READING\n\nHold Kpro effluent facing up and level with the pressure transducer.\nTurn on Kpro water, turn off when water flows with no air bubbles.\n\nPress OK when the reading equilibrates." ("message") -> [_ w2416]
                  tunnel: [w2407 w2415] -> w2397
                  tunnel: [w2406 w2409] -> w2394
                  tunnel: w2391 -> [_ w2414]
                  tunnel: w2390 -> [w2404 w2413]
                  tunnel: [w2405 w2412] -> w2389
                  tunnel: [w2401 w2411] -> w2384
                  tunnel: [w2404 w2410] -> w2383
                  tunnel: w2380 -> [w2406 w2409]
                  tunnel: w2379 -> [w2402 _]
                  tunnel: [w2400 w2408] -> w2376
                  tunnel: w2375 -> [w2400 w2408]
                  frame False {
                    n1051 = Unbundle By Name(w2406) -> ("Up Hole Pressure Slope"=w2405:dbl)
                    n1052 = local read "Sensor Voltage Cluster"() -> (w2407:T9)
                    n1053 = Scan From String(input string=w2402, default 1=35.0 ("default value 1")) -> (output 1=w2401:dbl)  [unwired: 3 in, 3 out]
                  }
                  frame True {
                    n1054 = Unbundle By Name(w2409) -> ("Up Hole Pressure Slope"=w2412:dbl)
                    n1055 = local read "Sensor Voltage Cluster"() -> (w2415:T9)
                    n1056 = call "Up Hole PRESSURE_CAL 2016.vi"("Pressure Offset"=w2408, "Descriptions"=w2414, "Array in"=w2413, "Pressure \nSlope"=w2412, "Sensor Cluster"=w2415, "Prompt_IN"=w2416) -> ("PRESSURE\nFt of water"=w2411:dbl, "Array out"=w2410:refnum<k24>[])  [unwired: 4 in]
                    "Pressure Offset" <- w2408
                  }
                }
                n1057 = call "up hole Pressure 2016.vi"("Sensor Cluster"=w2397, "Pressure Offset"=w2384, "Array in"=w2383, "Pressure \nSlope"=w2389, "Descriptions"=w2391, "Zero Pressure\n(F = leave as is)"=TRUE) -> ("Array out"=w2392:refnum<k24>[], "Uphole Pressure"=w2377:dbl, "Sensor Cluster 2"=w2387:T9)  [unwired: 6 in, 1 out]
                n1058 = Bundle By Name(cluster=w2396, "Up hole Corrected Pressure"=w2377) -> (w2395:T20)
                n1059 = local write "Uphole Pressure"(w2377) -> ()
                n1060 = global write "Kpro Globals.vi" "Atmospheric Pressure"(w2384) -> ()
                n1061 = local write "Corrected Pressure Cluster"(w2395) -> ()
                n1062 = local write "Sensor Voltage Cluster"(w2387) -> ()
                n1063 = Format Into String(w2384) -> (resulting string=w2385:string)  [unwired: 3 in, 1 out]
                n1064 = Bundle By Name(cluster=w2382, "Atmospheric Pressure"=w2385) -> (w2386:T10)
                n1065 = local write "Groundwater Header"(w2386) -> ()
                n1066 = Bundle By Name(cluster=w2394, "Atmospheric Pressure"=w2384, "Up Hole  Pressure Offset"=w2376) -> (w2393:T11)
                n1067 = local write "Input Variables and Slopes"(w2393) -> ()
              }
              frame #4 {
                n1068 = disable-structure shown="Disabled" {
                  disable-tunnel: w2418 -> [w2422 _]
                  disable-tunnel: w2417 -> [w2421 _]
                  frame Disabled {
                    w2430 = 0.0  # Offset
                    (unwired) FALSE
                    # "Take offset and put\n into Pressure VI."
                    n1069 = local read "Input Variables and Slopes"() -> (w2429:T11)
                    n1070 = Unbundle By Name(w2429) -> ()  [unwired: 2 out]
                    n1071 = local read item#-1() -> (w2426)
                    n1072 = local read "Input Variables and Slopes"() -> (w2436:T11)
                    n1073 = Unbundle By Name(w2436) -> ("Up Hole Pressure Slope"=w2423:dbl, "Flow Slope"=w2431:dbl)
                    n1074 = call "Flow 2016.vi"("Descriptions"=w2421, "Array in"=w2422, "Flow Slope"=w2431, "Offset"=w2430) -> ("Flow (ml/min)"=w2424:dbl)  [unwired: 4 in, 2 out]
                    n1075 = Bundle By Name(cluster=w2426, "Flow"=w2424) -> (w2425:cluster{})
                    n1076 = local write item#-1(w2425) -> ()
                    n1077 = local read "Corrected Pressure Cluster"() -> (w2435:T20)
                    n1078 = local read "Sensor Voltage Cluster"() -> (w2432:T9)
                    n1079 = Unbundle By Name(w2432) -> ()  [unwired: 1 out]
                    n1080 = call "Up Hole PRESSURE_CAL 2016.vi"("Descriptions"=w2421, "Array in"=w2422, "Pressure \nSlope"=w2423, "Sensor Cluster"=w2432, "Prompt_IN"="ZERO PRESSURE TRANSDUCER\n\nHold Kpro effluent in a grad cylinder with 800mL (1 ft) of water.\nHold grad cylinder with its bottom level with the pressure transducer.\n\nPress OK when the reading equilibrates. " ("message")) -> ("PRESSURE\nFt of water"=w2437:dbl)  [unwired: 5 in, 1 out]
                    n1081 = Subtract(x=w2437, y=1.0) -> (x-y=w2440:dbl)
                    n1082 = call "up hole Pressure 2016.vi"("Sensor Cluster"=w2432, "Pressure Offset"=w2440, "Array in"=w2422, "Pressure \nSlope"=w2423, "Descriptions"=w2421, "Zero Pressure\n(F = leave as is)"=TRUE) -> ("Uphole Pressure"=w2433:dbl, "Sensor Cluster 2"=w2419:T9)  [unwired: 6 in, 2 out]
                    n1083 = Bundle By Name(cluster=w2435, "Up hole Corrected Pressure"=w2433) -> (w2434:T20)
                    n1084 = local write "Sensor Voltage Cluster"(w2419) -> ()
                    n1085 = local write "Corrected Pressure Cluster"(w2434) -> ()
                    n1086 = local read "Input Variables and Slopes"() -> (w2428:T11)
                    n1087 = Unbundle By Name(w2428) -> ()  [unwired: 2 out]
                    n1088 = local write "Initialization"(4 ("Initialization")) -> ()
                    n1089 = local read "Input Variables and Slopes"() -> (w2427:T11)
                    n1090 = Unbundle By Name(w2427) -> ()  [unwired: 2 out]
                  }
                  frame Enabled {
                  }
                }
              }
              frame #5 {
                n1091 = flat-sequence {
                  tunnel: w2444 -> [w2453]
                  tunnel: w2443 -> [w2452]
                  frame #0 {
                    n1092 = local read "Sensor Voltage Cluster"() -> (w2456:T9)
                    n1093 = local read "Input Variables and Slopes"() -> (w2451:T11)
                    n1094 = Unbundle By Name(w2451) -> ("Up Hole Pressure Slope"=w2450:dbl)
                    n1095 = global read "Kpro Globals.vi" "Pressure Offset"() -> (w2449:dbl)
                    n1096 = call "Up Hole PRESSURE_CAL 2016.vi"("Pressure Offset"=w2449, "Descriptions"=w2452, "Array in"=w2453, "Pressure \nSlope"=w2450, "Sensor Cluster"=w2456, "Prompt_IN"="CHECK RESERVOIR PRESSURE\n\nTurn on Kpro. Unplug Kpro Out quick connect from sample box.\nReservoir pressure should be 69.2 +/- 5%(65.7 - 72.7).\n\nPress OK when the reading equilibrates within range." ("message")) -> ("PRESSURE\nFt of water"=w2446:dbl)  [unwired: 4 in, 1 out]
                    n1097 = Bundle By Name(cluster=w2451, "Reservoir Pressure"=w2446) -> (w2454:T11)
                    n1098 = global write "Kpro Globals.vi" "Reservoir Pressure"(w2446) -> ()
                    n1099 = Format Into String(w2446) -> (resulting string=w2445:string)  [unwired: 3 in, 1 out]
                    n1100 = local write "Input Variables and Slopes"(w2454) -> ()
                    n1101 = local read "Groundwater Header"() -> (w2448:T10)
                    n1102 = Bundle By Name(cluster=w2448, "KPRO N2 Pressure"=w2445) -> (w2447:T10)
                    n1103 = local write "Groundwater Header"(w2447) -> ()
                  }
                }
                n1104 = local write "Initialization"(5 ("Initialization")) -> ()
              }
              frame #6 {
                n1105 = local write "Initialization"(6 ("Initialization")) -> ()
                n1106 = flat-sequence {
                  frame #0 {
                    n1107 = local read "Input Depths \nand Parameters Cluster"() -> (w2462:T16)
                    n1108 = Unbundle By Name(w2462) -> ("Start Depth"=w2459:sgl)
                    n1109 = call "prompt_and_enter_value 2016.vi"("prompt_IN"="ENTER START DEPTH", "Enter value"=w2459) -> ("Numeric"=w2464:dbl)  [unwired: 9 in]
                    n1110 = Absolute Value(x=w2464) -> (abs(x)=w2463:dbl)
                    n1111 = Negate(x=w2463) -> (-x=w2460:dbl)
                    n1112 = Bundle By Name(cluster=w2462, "Start Depth"=w2460) -> (w2461:T16)
                    n1113 = local write "Input Depths \nand Parameters Cluster"(w2461) -> ()
                  }
                }
              }
              frame #7 {
                n1114 = local write "Initialization"(7 ("Initialization")) -> ()
                n1115 = local read "Input Variables and Slopes"() -> (w2470:T11)
                n1116 = Unbundle By Name(w2470) -> ("Height of Sample Box"=w2468:dbl)
                n1117 = call "prompt_and_enter_value 2016.vi"("prompt_IN"="HEIGHT FROM GROUND SURFACE TO SAMPLE BOX\n\nMeasure the vertical distance between the ground surface and the pressure transducer." ("prompt"), "Enter value"=w2468) -> ("Numeric"=w2467:dbl)  [unwired: 9 in]
                n1118 = Bundle By Name(cluster=w2470, "Height of Sample Box"=w2467) -> (w2469:T11)
                n1119 = global write "Kpro Globals.vi" "height_of_box"(w2467) -> ()
                n1120 = local write "Input Variables and Slopes"(w2469) -> ()
              }
              frame #8 {
                n1121 = flat-sequence {
                  frame #0 {
                    n1122 = local read "Input Variables and Slopes"() -> (w2475:T11)
                    n1123 = Unbundle By Name(w2475) -> ("Depth to Water Table"=w2476:dbl)
                    n1124 = call "prompt_and_enter_value 2016.vi"("prompt_IN"="DEPTH TO WATER TABLE\n\nEnter the depth to the water table." ("prompt"), "Enter value"=w2476) -> ("Numeric"=w2478:dbl)  [unwired: 9 in]
                    n1125 = Absolute Value(x=w2478) -> (abs(x)=w2477:dbl)
                    n1126 = Negate(x=w2477) -> (-x=w2474:dbl)
                    n1127 = Bundle By Name(cluster=w2475, "Depth to Water Table"=w2474) -> (w2473:T11)
                    n1128 = local write "Input Variables and Slopes"(w2473) -> ()
                    n1129 = global write "Kpro Globals.vi" "Depth to Water Table"(w2474) -> ()
                  }
                }
                n1130 = local write "Initialization"(8 ("Initialization")) -> ()
              }
              frame #9 {
                n1131 = local read "Corrected Pressure Cluster"() -> (w2487:T20)
                n1132 = local write "Initialization"(9 ("Initialization")) -> ()
                n1133 = local read "Input Variables and Slopes"() -> (w2484:T11)
                n1134 = Unbundle By Name(w2484) -> ("Up Hole Pressure Slope"=w2482:dbl)
                n1135 = stacked-sequence {
                  tunnel: [_ w2507] -> w2485
                  tunnel: w2482 -> [w2494 w2506]
                  tunnel: w2481 -> [w2489 w2505]
                  tunnel: w2483 -> [w2488 w2501]
                  tunnel: w2482 -> [_ w2504]
                  tunnel: w2481 -> [_ w2502]
                  frame #0 {
                    # "Set to raw pressure mode"
                    n1136 = local read "Corrected Pressure Cluster"() -> (w2491:T20)
                    n1137 = local read "Sensor Voltage Cluster"() -> (w2493:T9)
                    n1138 = call "up hole Pressure 2016.vi"("Sensor Cluster"=w2493, "Pressure Offset"=0.0, "Array in"=w2488, "Pressure \nSlope"=w2494, "Descriptions"=w2489, "Zero Pressure\n(F = leave as is)"=TRUE) -> ("Uphole Pressure"=w2492:dbl)  [unwired: 6 in, 3 out]
                    n1139 = Bundle By Name(cluster=w2491, "Up hole Corrected Pressure"=w2492) -> (w2490:T20)
                    n1140 = local write "Corrected Pressure Cluster"(w2490) -> ()
                  }
                  frame #1 {
                    # "adjust for 1 foot head"
                    # "Take offset and put\n into Pressure VI."
                    n1141 = local read "Sensor Voltage Cluster"() -> (w2508:T9)
                    n1142 = global read "Kpro Globals.vi" "Pressure Offset"() -> (w2503:dbl)
                    n1143 = call "Up Hole PRESSURE_CAL 2016.vi"("Pressure Offset"=w2503, "Descriptions"=w2502, "Array in"=w2501, "Pressure \nSlope"=w2504, "Sensor Cluster"=w2508, "Prompt_IN"="ZERO TO GROUND SURFACE\n\nFill a grad cylinder to 750mL.\nPlace it on the ground at the profile location.\nImmerse the Kpro effluent and turn on Kpro flow.\nTurn off after water is flowing with no bubbles\nand the water has reached 800mL (1 foot).\n\nPress OK when the reading equilibrates." ("message")) -> ("PRESSURE\nFt of water"=w2509:dbl)  [unwired: 4 in, 1 out]
                    n1144 = Decrement(x=w2509) -> (x-1=w2500:dbl)
                    n1145 = call "up hole Pressure 2016.vi"("Sensor Cluster"=w2508, "Pressure Offset"=w2500, "Array in"=w2501, "Pressure \nSlope"=w2506, "Descriptions"=w2505, "Zero Pressure\n(F = leave as is)"=TRUE) -> ("Uphole Pressure"=w2507:dbl, "Pressure Offset 2"=w2497:dbl)  [unwired: 6 in, 2 out]
                    n1146 = local read "Input Variables and Slopes"() -> (w2499:T11)
                    n1147 = Bundle By Name(cluster=w2499, "Up Hole  Pressure Offset"=w2497) -> (w2498:T11)
                    n1148 = local write "Input Variables and Slopes"(w2498) -> ()
                  }
                }
                n1149 = Bundle By Name(cluster=w2487, "Up hole Corrected Pressure"=w2485) -> (w2486:T20)
                n1150 = local write "Corrected Pressure Cluster"(w2486) -> ()
              }
              frame #10 {
                n1151 = local write "Initialization"(10 ("Initialization")) -> ()
                n1152 = local read "Cumulative_data_ready"() -> (w2517:bool)
                n1153 = case shown="True" w2517 {
                  tunnel: w2516 -> [w2518 _]
                  tunnel: [w2518 w2519] -> w2515
                  frame False {
                  }
                  frame True {
                    n1154 = local write "Cumulative_data_ready"(FALSE ("Get_KPRO_data")) -> ()
                    n1155 = local read "Cumulative_data_from_file"() -> (w2519:sgl[][])
                  }
                }
                "Zero Pressure\nIndicator" <- FALSE ("Zero Pressure\nIndicator")
              }
            }
          }
          frame "Acq. DAQ data" {
            n1156 = flat-sequence {
              tunnel: w2612 -> [w2629]
              tunnel: w2611 -> [w2628]
              tunnel: [w2625] -> w2610
              frame #0 {
                n1157 = local read "Descriptions"() -> (w2626:string[])
                n1158 = call "Measure DAQ Voltages.vi"("error in (no error)"=w2628, "Descriptions"=w2626, "Array in"=w2629) -> ("Raw Voltages"=→"Raw Voltages":dbl[], "Array out"=w2625:refnum<k24>[], "Sensor Cluster"=w2621:T9)  [unwired: 6 in]
                "Sensor Voltage Cluster" <- w2621
                n1159 = local read "Sensor  Real \nMeasurements"() -> (w2624:T6)
                n1160 = local read "Input Variables and Slopes"() -> (w2622:T11)
                n1161 = call "convert sensor voltage to real measurements.vi"("Input Variables and Slopes"=w2622, "Sensor  Real Measurements in"=w2624, "Sensor Cluster"=w2621) -> ("Sensor  Real Measurements out"=w2623:T9)  [unwired: 8 in]
                n1162 = local write "Sensor  Real \nMeasurements"(w2623) -> ()
              }
            }
          }
          frame "Exit" {
            n1163 = case shown="No Error" w2645 {
              tunnel: w2641 -> [w2688 _]
              tunnel: w2645 -> [w2687 w2699]
              tunnel: [w2686 w2699] -> w2643
              frame No Error {
                n1164 = for {
                  shift-right: [w2690] -> w2686
                  shift-left: w2687 -> [w2691]
                  tunnel: w2688 -> [w2689] mode=indexing
                  n1165 = while {
                    shift-right: [w2698] -> w2693
                    shift-left: w2691 -> [w2696]
                    shift-right: [w2697] -> w2692
                    shift-left: w2689 -> [w2695]
                    stop <- w2694 stop-if-true
                    n1166 = call <vilib>:"ULx Is Task Done.vi"("task in"=w2695, "error in"=w2696) -> ("task out"=w2697:refnum<k24>, "task done?"=w2694:bool, "error out"=w2698:errorcluster)  [unwired: 11 in]
                  }
                  n1167 = call <vilib>:"ULx Clear Task.vi"("task in"=w2692, "error in"=w2693) -> ("error out"=w2690:errorcluster)  [unwired: 13 in]
                }
              }
              frame Error {
              }
            }
            n1168 = flat-sequence {
              tunnel: w2654 -> [w2674]
              tunnel: w2652 -> [w2672]
              tunnel: [w2670] -> w2646
              frame #0 {
                (unwired) FALSE ("Write Ini")
                n1169 = case shown="False" "Save Configuration File?" {
                  tunnel: [errorcluster {"status"=FALSE, "code"=0, "source"=""} ("error IO") w2683] -> w2671
                  frame False {
                  }
                  frame True {
                    n1170 = local read "Config File Path"() -> (w2682:path)
                    n1171 = call <vilib>:"Open Config Data.vi"("create file if necessary (T)"=TRUE ("Read Ini"), "configuration file path"=w2682) -> ("error out"=w2680:errorcluster, "refnum"=w2677:T23)  [unwired: 7 in, 1 out]
                    n1172 = control-ref of="This VI"() -> (w2676:refnum<vi>)
                    n1173 = call <userlib>:"Write Panel to INI__ogtk.vi"("error in (no error)"=w2680, "VI ref"=w2676, "refnum"=w2677) -> ("error out"=w2679:errorcluster, "refnum out"=w2678:T23)  [unwired: 7 in]
                    n1174 = call <vilib>:"Clear Errors.vi"("error in (no error)"=w2679) -> ("error out"=w2685:errorcluster)  [unwired: 5 in, 1 out]
                    n1175 = call <vilib>:"Close Config Data.vi"("error in (no error)"=w2685, "refnum"=w2678) -> ("error out"=w2684:errorcluster)  [unwired: 8 in, 1 out]
                    n1176 = Merge Errors(w2684, w2679) -> (w2683:errorcluster)
                  }
                }
                n1177 = call-dynamic "Dispose Report.vi"("report in"=w2672, "save changes? (F)"=FALSE, "error in (no error)"=w2674) -> ("error out"=w2669:errorcluster)  [unwired: 12 in]
                n1178 = Merge Errors(w2671, w2669) -> (w2670:errorcluster)
              }
            }
            n1179 = flat-sequence {
              tunnel: [w2657] -> _
              tunnel: [w2664] -> w2634
              tunnel: w2637 -> [w2659]
              tunnel: w2636 -> [w2657]
              tunnel: [w2656] -> w2635
              frame #0 {
                w2663 = "Groundwater Profile Log" ("Worksheet Name in")
                n1180 = local write "Current Sample Sheet"(w2663) -> ()
                n1181 = local read "Worksheet Names"() -> (w2661:string[])
                n1182 = call "find and open select worksheet.vi"("Worksheet Names"=w2661, "error in (no error)"=w2657, "milliseconds to wait"=u32 100, "Worksheet Name in"=w2663, "NI_report in"=w2659) -> ("error out"=w2660:errorcluster, "NI_report out"=w2658:refnum<class "NI_report.lvclass">)  [unwired: 4 in, 1 out]
                n1183 = call "groundwater log header.vi"("Worksheet Names"=w2661, "Groundwater Header"="Groundwater Header", "error in (no error)"=w2660, "NI_report in"=w2658) -> ("error out"=w2656:errorcluster, "NI_report out"=w2664:refnum<class "NI_report.lvclass">)  [unwired: 6 in]
              }
            }
            n1184 = flat-sequence {
              tunnel: [w2705] -> w2652
              tunnel: [w2704] -> w2653
              tunnel: w2635 -> [w2702]
              tunnel: w2634 -> [w2701]
              frame #0 {
                n1185 = local read "Excel report file path"() -> (w2700:path)
                n1186 = call-dynamic "Save Report to File.vi"("report in"=w2701, "report file path"=w2700, "prompt to replace? (F)"=FALSE, "error in (no error)"=w2702) -> ("report out"=w2705:refnum<class "NI_report.lvclass">, "error out"=w2704:errorcluster)  [unwired: 10 in]
              }
            }
            n1187 = flat-sequence {
              tunnel: [TRUE ("aborted?")] -> w2644
              tunnel: [w2666] -> w2642
              tunnel: w2643 -> [w2666]
              frame #0 {
              }
            }
            n1188 = call <userlib>:"Wait (ms)__ogtk.vi"("error in (no error)"=w2653, "milliseconds to wait"=u32 5) -> ("error out"=w2654:errorcluster)  [unwired: 8 in, 1 out]
          }
          frame "Create Excel Files" {
            n1189 = flat-sequence {
              tunnel: w2710 -> [w2757]
              tunnel: [w2751] -> w2707
              tunnel: [w2747] -> w2708
              tunnel: [w2738] -> w2709
              frame #0 {
                n1190 = flat-sequence {
                  tunnel: w2748 -> [w2776]
                  tunnel: [w2775] -> _
                  tunnel: [w2773] -> w2738
                  tunnel: [w2771] -> w2747
                  tunnel: w2744 -> [w2770]
                  tunnel: w2743 -> [w2769]
                  frame #0 {
                    w2759 = "Sample 1" ("Worksheet Name in")
                    n1191 = call "find and open select worksheet.vi"("Worksheet Names"=w2776, "error in (no error)"=w2769, "milliseconds to wait"=u32 100, "Worksheet Name in"=w2759, "NI_report in"=w2770) -> ("error out"=w2772:errorcluster, "Select Worksheet Index"=w2775:i32, "NI_report out"=w2774:refnum<class "NI_report.lvclass">)  [unwired: 4 in]
                    "Select Worksheet Index" <- w2775
                    n1192 = call "get sample sheet data cells.vi"("error in (no error)"=w2772, "NI_report in"=w2774) -> ("error out"=w2765:errorcluster, "data"=w2766:string[][], "NI_report out"=w2773:refnum<class "NI_report.lvclass">, "left edge output cluster"=w2764:cluster{"row":i32, "column":i32})  [unwired: 5 in, 1 out]
                    "NI_report out" <- w2773
                    n1193 = Array Subset(array=w2766, index (col)=2 ("index")) -> (→"subarray":string[][])  [unwired: 3 in]
                    n1194 = call "find last occupied cell.vi"("data"=w2766, "Active Sheet"=w2759, "Header Rows to remove"=3, "sub array start"=w2764, "error in (no error)"=w2765) -> ("row max value"=w2763:i32, "column max value"=→"column max value":i32, "start of last occupied row"=→"last occupied cell's name":string, "error out"=w2771:errorcluster)  [unwired: 4 in, 3 out]
                    n1195 = local write "row max value"(w2763) -> ()
                    "Current Sample Sheet" <- w2759
                  }
                }
                n1196 = call "get sample header columns.vi"("report file path"="Header path", "Start Cell Name"="a3", "Stop Cell name"="b22", "error in (no error)"=w2757) -> ("Column of Volume"=→"row max value":i32, "Columns"=→"Columns":i32[], "error out"=w2758:errorcluster)  [unwired: 2 in, 7 out]
                n1197 = call "close excel file if open.vi"("error in (no error)"=w2758, "report file path in"="Excel report file path") -> ("error out"=w2752:errorcluster, "report file path out"=w2746:path)  [unwired: 8 in]
                n1198 = call "copy excel template.vi"("error in (no error)"=w2752, "report file path in"=w2746, "template file path in"="template file path") -> ("error out"=w2753:errorcluster, "report file path out"=w2755:path)  [unwired: 7 in]
                n1199 = call "open excel get worksheet names.vi"("window state (normal)"=T26."normal", "error in (no error)"=w2753, "milliseconds to wait"=u32 5, "report file path"=w2755) -> ("error out"=w2743:errorcluster, "Number of Sample Sheets"=w2751:i32, "NI_report out"=w2744:refnum<class "NI_report.lvclass">, "Worksheet Names"=w2748:string[])  [unwired: 2 in, 2 out]
                "Worksheet Names" <- w2748
                "Number of Sample Sheets" <- w2751
              }
            }
            n1200 = flat-sequence {
              tunnel: [w2785] -> w2727
              tunnel: [w2784] -> w2728
              tunnel: w2708 -> [w2782]
              tunnel: w2709 -> [w2781]
              frame #0 {
                n1201 = local read "Excel report file path"() -> (w2780:path)
                n1202 = call-dynamic "Save Report to File.vi"("report in"=w2781, "report file path"=w2780, "prompt to replace? (F)"=FALSE, "error in (no error)"=w2782) -> ("report out"=w2785:refnum<class "NI_report.lvclass">, "error out"=w2784:errorcluster)  [unwired: 10 in]
              }
            }
            n1203 = flat-sequence {
              tunnel: w2707 -> [w2737]
              tunnel: w2706 -> [w2733]
              tunnel: w2708 -> [w2732]
              tunnel: [w2731] -> _
              frame #0 {
                n1204 = local read "Worksheet Names"() -> (w2730:string[])
                n1205 = call "open select sample sheet.vi"("Number of Sample Sheets"=w2737, "error in (no error)"=w2732, "Worksheet Names"=w2730, "input 1"=w2733) -> ("error out"=w2735:errorcluster, "Current Sample Sheet"=w2736:string)  [unwired: 5 in, 1 out]
                n1206 = local write "Current Sample Sheet"(w2736) -> ()
                n1207 = Scan From String(format string="Sample %d", input string=w2736, error in=w2735) -> (error out=w2731:errorcluster)  [unwired: 3 in, 2 out]
              }
            }
            n1208 = flat-sequence {
              tunnel: [FALSE ("aborted?")] -> w2722
              tunnel: [w2778] -> w2721
              tunnel: w2712 -> [w2778]
              frame #0 {
              }
            }
            n1209 = call <userlib>:"Wait (ms)__ogtk.vi"("error in (no error)"=w2728, "milliseconds to wait"=u32 5) -> ("error out"=w2711:errorcluster)  [unwired: 8 in, 1 out]
          }
        }
        n1210 = local write "Depth Cluster"(w389) -> ()
      }
    }
  }
